vi "comm.vi"() -> ()   [LabVIEW 2015]
uses:
  G_SEN.vi
  G_NAV.vi
panel:
  out "time loop":dbl
  out "time IBEO":dbl format="%#_20g"
  out "Waveform Chart":T1(graph)
  out "output cluster 2":T2 {"Header"."Data type" format="%x"}
  out "value":T3 {"Data type" format="%x"}
  out "scan data 2202":string
  out "object data 2221":string
  out "Ibeo error out":errorcluster
  in  "Ibeo reconn?":bool=TRUE
  in  "Sensor reconn?":bool=TRUE
  in  "Sensor Port":u16=6553
  out "error out":errorcluster
  out "send error":errorcluster
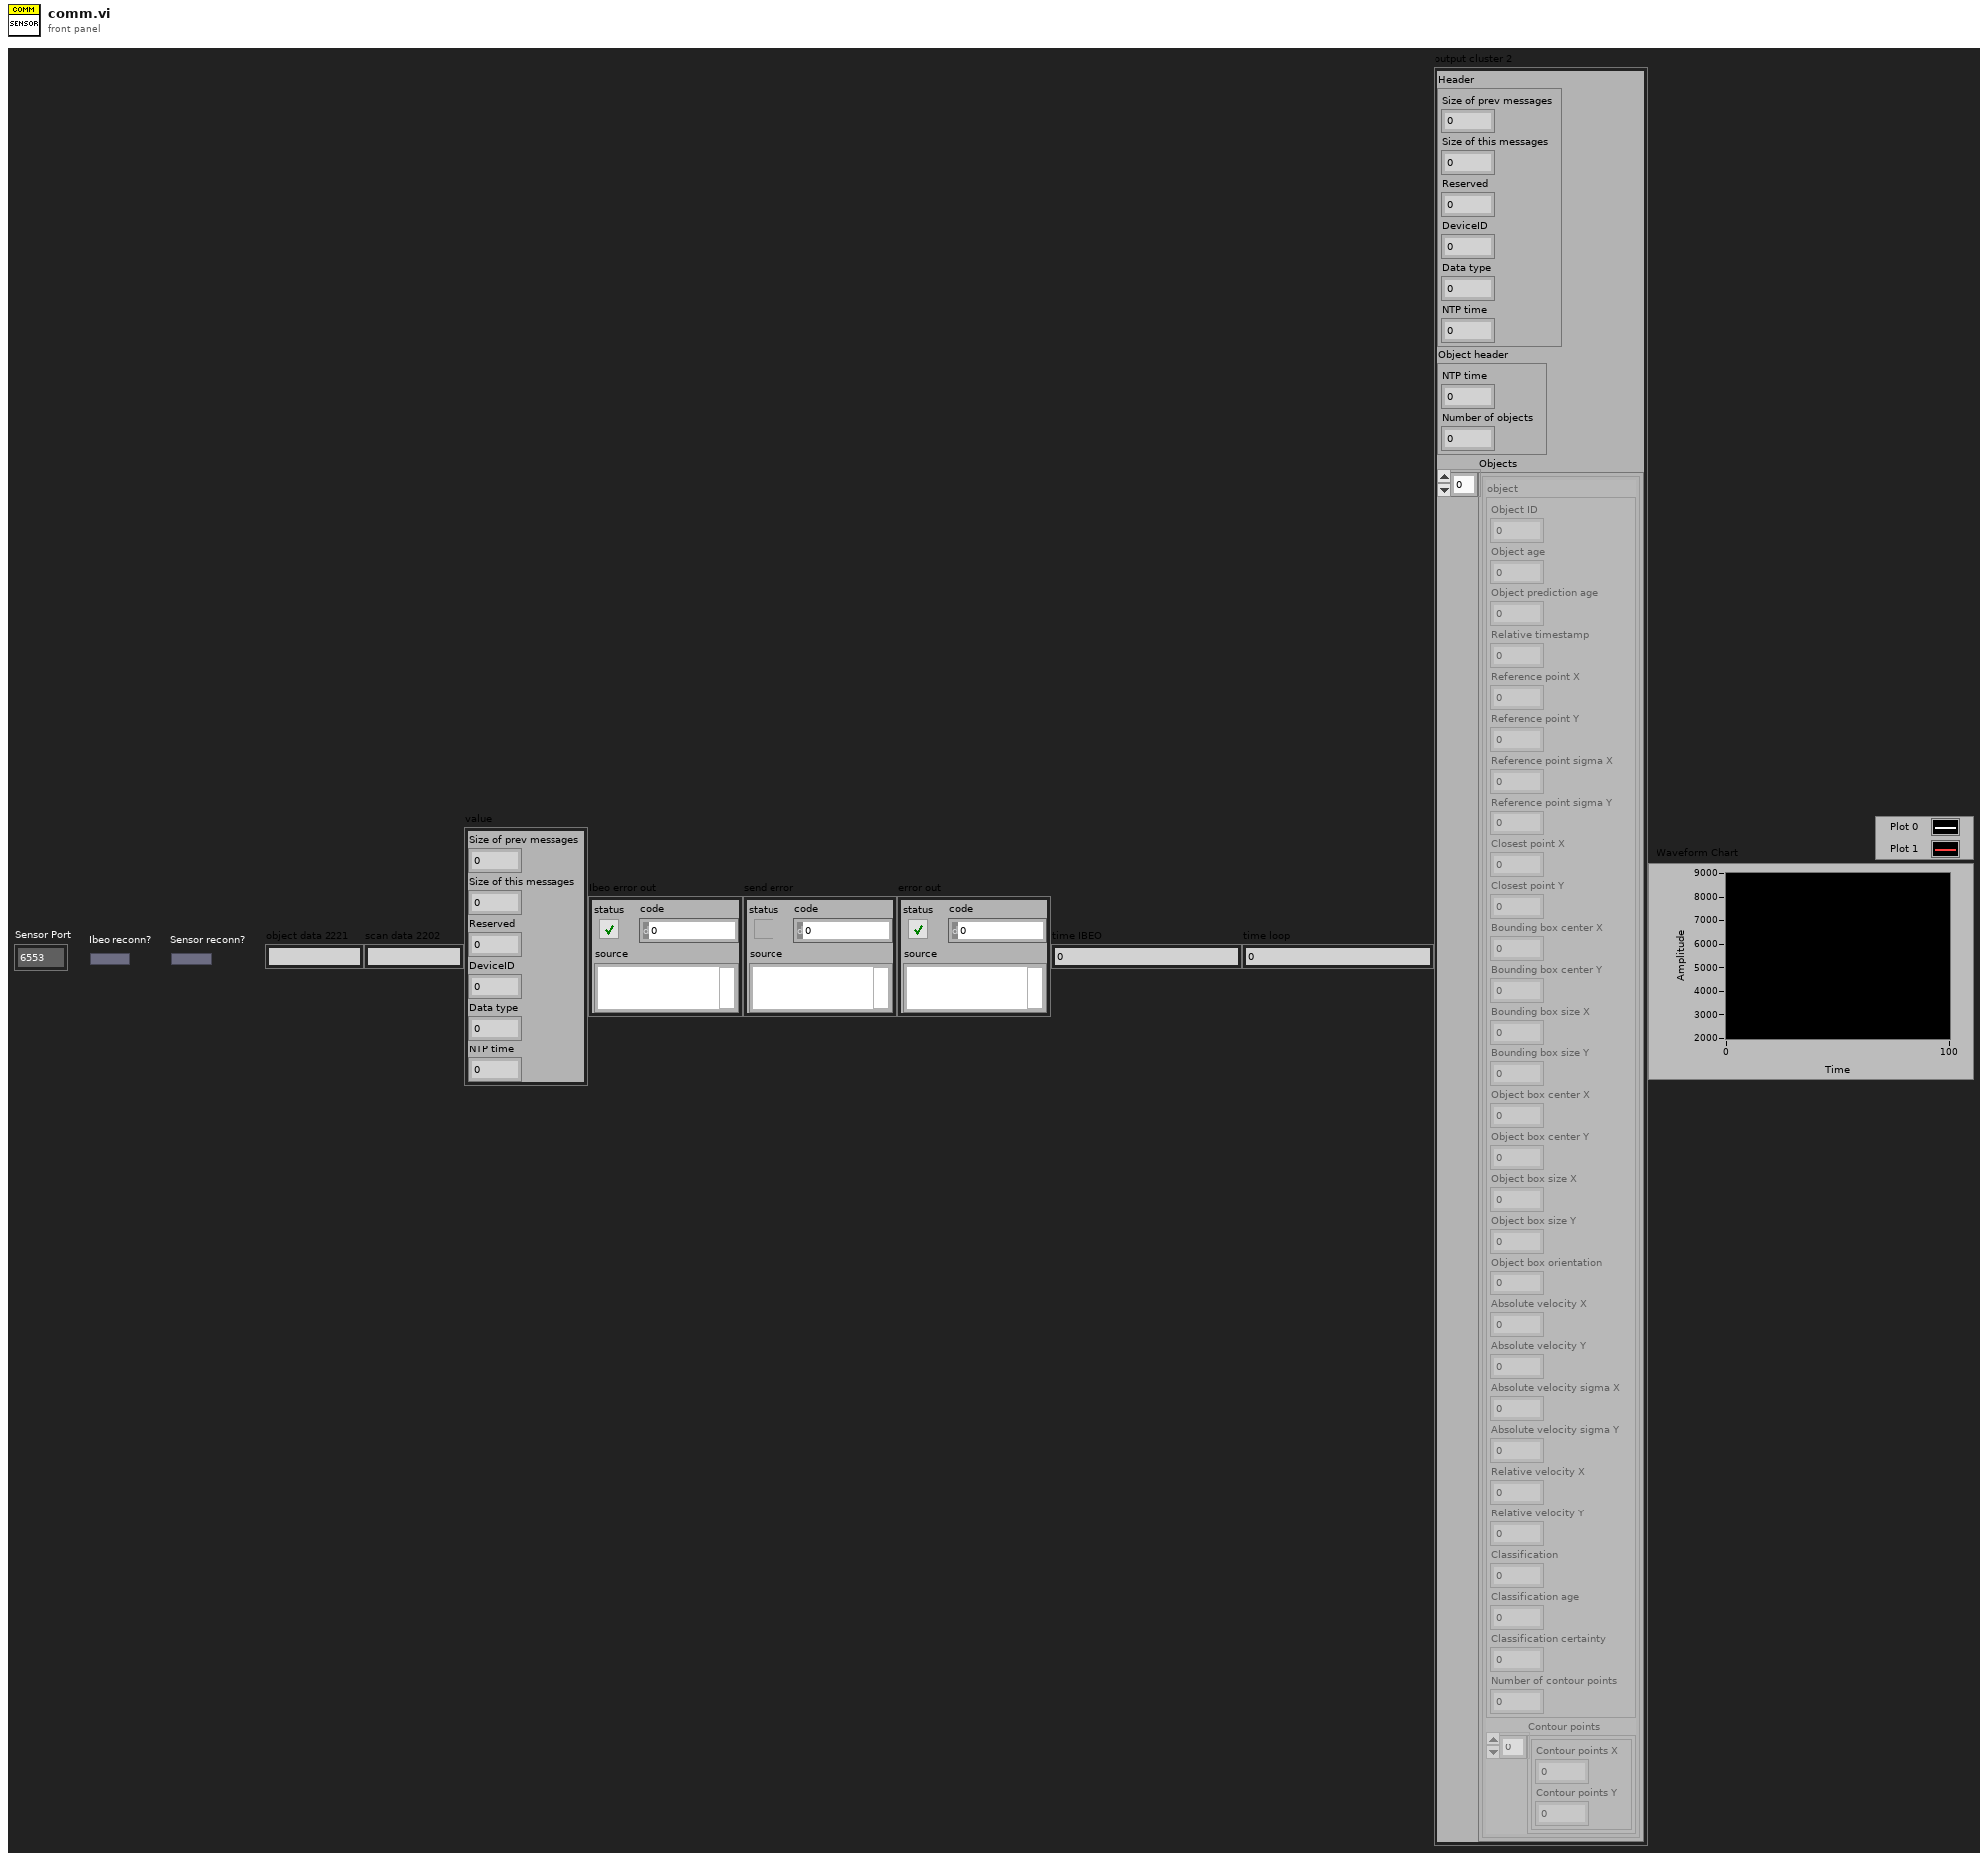
[diagram p1: front panel]
types:
  T1 = cluster{"Data type":u16, "Size of this messages":u32}
  T2 = cluster{"Header":cluster{"Size of prev messages":u32, "Size of this messages":u32, "Reserved":u8, "DeviceID":u8, "Data type":u16, "NTP time":u64}, "Object header":cluster{"NTP time":u64, "Number of objects":u16}, "Objects":cluster{"object":cluster{"Object ID":u16, "Object age ":u16, "Object prediction age":u16, "Relative timestamp":u16, "Reference point X":dbl, "Reference point Y":dbl, "Reference point sigma X":dbl, "Reference point sigma Y":dbl, "Closest point X":dbl, "Closest point Y":dbl, "Bounding box center X":dbl, "Bounding box center Y":dbl, "Bounding box size X":dbl, "Bounding box size Y":dbl, "Object box center X":dbl, "Object box center Y":dbl, "Object box size X":dbl, "Object box size Y":dbl, "Object box orientation":dbl, "Absolute velocity X":dbl, "Absolute velocity Y":dbl, "Absolute velocity sigma X":dbl, "Absolute velocity sigma Y":dbl, "Relative velocity X":dbl, "Relative velocity Y":dbl, "Classification":u16, "Classification age":u16, "Classification certainty":u16, "Number of contour points":u16}, "Contour points":cluster{"Contour points X":dbl, "Contour points Y":dbl}[]}[]}
  T3 = cluster{"Size of prev messages":u32, "Size of this messages":u32, "Reserved":u8, "DeviceID":u8, "Data type":u16, "NTP time":u64}
  T4 = cluster{"global_x":sgl, " global_y":sgl, "yaw":sgl, "objCount":u16, "total":u16}
  T5 = enum16{"big-endian, network order", "native, host order", "little-endian"}
  T6 = cluster{"GPSTime":dbl, "attitude[2]":dbl, "lcc[0]":dbl, "lcc[1]":dbl, "heading_GPS":dbl}
  T7 = cluster{"Header":cluster{"Size of prev messages":u32, "Size of this messages":u32, "Reserved":u8, "DeviceID":u8, "Data type":u16, "NTP time":u64}, "Scan header":cluster{"Scan number":u16, "scanner status":u16, "Sync phase offset":u16, "Scan start time NTP":u64, "Scan end time NTP":u64, "Angle ticks per rotation":u16, "Start angle":dbl, "End angle":dbl, "Scan points":u16, "Mounting position yaw angle ":dbl, "Mounting position pitch angle":dbl, "Mounting position roll angle":dbl, "Mounting position x":dbl, "Mounting position y":dbl, "Mounting position z":dbl, "Reserved":u16}, "Scan points":cluster{"flags":u8, "Echo":u8, "Radial distance":dbl, "Horizontal angle":dbl, "Vertical angle":dbl, "Echo pulse width":u16, "Reserved":u16}[]}
  T8 = cluster{"Header":cluster{"Size of prev messages":u32, "Size of this messages":u32, "Reserved":u8, "DeviceID":u8, "Data type":u16, "NTP time":u64}, "Scan header":cluster{"NTP time":u64, "Scan end Time offset":u32, "flags":u32, "Scan number":u16, "Scan points":u16, "Number of Scan infos":u8, "reserved":u8, "reserved 2":u16}, "Scanner info":cluster{"Device ID ":u8, "Scanner type":u8, "Scan number":u16, "Reserved 4":u32, "Start angle":sgl, "End angle":sgl, "Scan start time ":u64, "Scan end time ":u64, "Scan start time from device":u64, "Scan end time from device":u64, "Scan frequency":sgl, "Beam tilt":sgl, "scan flags":u32, "Yaw angle ":sgl, "Pitch angle ":sgl, "Roll angle":sgl, "Offset x ":sgl, "Offset y":sgl, "Offset z":sgl, "Reserved 8 1":u64, "Reserved 8 2":u64, "Reserved 8 3":u64, "Reserved 8 4":u64, "Reserved 8 5":u64, "Reserved 8 6":u64, "Reserved 8 7":u64, "Reserved 8 8":u64}, "Scan points":cluster{"X  position":sgl, "Y  position":sgl, "Z  position":sgl, "Echo width":sgl, "Device ID ":u8, "Layer":u8, "Echo":u8, "Reserved":u8, "Timestamp":u32, "flags":u16, "Reserved 2":u16}[]}
  T9 = cluster{"Header":cluster{"Size of prev messages":u32, "Size of this messages":u32, "Reserved":u8, "DeviceID":u8, "Data type":u16, "NTP time":u64}, "Object header":cluster{"NTP time":u64, "Number of objects":u16}, "Objects":cluster{"object":cluster{"Object ID":u16, "Reserved 2 1":u16, "Object age ":u32, "Timestamp NTP ":u64, "Object hidden status age":u16, "Classification":u8, "Classification certainty":u8, "Classification age":u32, "Bounding box center X":sgl, "Bounding box center Y":sgl, "Bounding box size X":sgl, "Bounding box size Y":sgl, "Object box center X":sgl, "Object box center Y":sgl, "Object box center sigma X":sgl, "Object box center sigma Y":sgl, "Object box size X":sgl, "Object box size Y":sgl, "Reserved 8 1":u64, "Yaw angle":sgl, "Reserved 4":u32, "Relative velocity X":sgl, "Relative velocity Y":sgl, "Relative velocity sigma X":sgl, "Relative velocity sigma Y":sgl, "Absolute velocity X":sgl, "Absolute velocity Y":sgl, "Absolute velocity sigma X":sgl, "Absolute velocity sigma Y":sgl, "Reserved 8 3":u64, "Reserved 8 4":u64, "Reserved 2 2":u16, "Number of contour points":u8, "Index of closest point":u8}, "Contour Points":cluster{"contour points X":sgl, "contour points Y":sgl}[]}[]}
  T10 = cluster{"Scan number":u16, "scanner status":u16, "Sync phase offset":u16, "Scan start time NTP":u64, "Scan end time NTP":u64, "Angle ticks per rotation":u16, "Start angle":i16, "End angle":i16, "Scan points":u16, "Mounting position yaw angle ":i16, "Mounting position pitch angle":i16, "Mounting position roll angle":i16, "Mounting position x":i16, "Mounting position y":i16, "Mounting position z":i16, "Reserved":u16}
  T11 = cluster{"flags":u8, "Echo":u8, "Radial distance":dbl, "Horizontal angle":dbl, "Vertical angle":dbl, "Echo pulse width":u16, "Reserved":u16}
  T12 = cluster{"Layer/Echo":u8, "flags":u8, "Horizontal angle":i16, "Radial distance":u16, "Echo pulse width":u16, "Reserved":u16}
  T13 = cluster{"Scan number":u16, "scanner status":u16, "Sync phase offset":u16, "Scan start time NTP":u64, "Scan end time NTP":u64, "Angle ticks per rotation":u16, "Start angle":dbl, "End angle":dbl, "Scan points":u16, "Mounting position yaw angle ":dbl, "Mounting position pitch angle":dbl, "Mounting position roll angle":dbl, "Mounting position x":dbl, "Mounting position y":dbl, "Mounting position z":dbl, "Reserved":u16}
  T14 = cluster{"Device ID ":u8, "Scanner type":u8, "Scan number":u16, "Reserved 4":u32, "Start angle":sgl, "End angle":sgl, "Scan start time ":u64, "Scan end time ":u64, "Scan start time from device":u64, "Scan end time from device":u64, "Scan frequency":sgl, "Beam tilt":sgl, "scan flags":u32, "Yaw angle ":sgl, "Pitch angle ":sgl, "Roll angle":sgl, "Offset x ":sgl, "Offset y":sgl, "Offset z":sgl, "Reserved 8 1":u64, "Reserved 8 2":u64, "Reserved 8 3":u64, "Reserved 8 4":u64, "Reserved 8 5":u64, "Reserved 8 6":u64, "Reserved 8 7":u64, "Reserved 8 8":u64}
  T15 = cluster{"NTP time":u64, "Scan end Time offset":u32, "flags":u32, "Scan number":u16, "Scan points":u16, "Number of Scan infos":u8, "reserved":u8, "reserved 2":u16}
  T16 = cluster{"X  position":sgl, "Y  position":sgl, "Z  position":sgl, "Echo width":sgl, "Device ID ":u8, "Layer":u8, "Echo":u8, "Reserved":u8, "Timestamp":u32, "flags":u16, "Reserved 2":u16}
  T17 = cluster{"Object ID":u16, "Object age ":u16, "Object prediction age":u16, "Relative timestamp":u16, "Reference point X":i16, "Reference point Y":i16, "Reference point sigma X":i16, "Reference point sigma Y":i16, "Closest point X":i16, "Closest point Y":i16, "Bounding box center X":i16, "Bounding box center Y":i16, "Bounding box size X":u16, "Bounding box size Y":u16, "Object box center X":i16, "Object box center Y":i16, "Object box size X":u16, "Object box size Y":u16, "Object box orientation":i16, "Absolute velocity X":i16, "Absolute velocity Y":i16, "Absolute velocity sigma X":u16, "Absolute velocity sigma Y":u16, "Relative velocity X":i16, "Relative velocity Y":i16, "Classification":u16, "Classification age":u16, "Classification certainty":u16, "Number of contour points":u16}
  T18 = cluster{"contour points X":i16, "contour points Y":i16}
  T19 = cluster{"contour points X":dbl, "contour points Y":dbl}
  T20 = cluster{"Object ID":u16, "Object age ":u16, "Object prediction age":u16, "Relative timestamp":u16, "Reference point X":dbl, "Reference point Y":dbl, "Reference point sigma X":dbl, "Reference point sigma Y":dbl, "Closest point X":dbl, "Closest point Y":dbl, "Bounding box center X":dbl, "Bounding box center Y":dbl, "Bounding box size X":dbl, "Bounding box size Y":dbl, "Object box center X":dbl, "Object box center Y":dbl, "Object box size X":dbl, "Object box size Y":dbl, "Object box orientation":dbl, "Absolute velocity X":dbl, "Absolute velocity Y":dbl, "Absolute velocity sigma X":dbl, "Absolute velocity sigma Y":dbl, "Relative velocity X":dbl, "Relative velocity Y":dbl, "Classification":u16, "Classification age":u16, "Classification certainty":u16, "Number of contour points":u16}
  T21 = cluster{"Object ID":dbl, "Object age ":dbl, "Object prediction age":dbl, "Relative timestamp":dbl, "Reference point X":dbl, "Reference point Y":dbl, "Reference point sigma X":dbl, "Reference point sigma Y":dbl, "Closest point X":dbl, "Closest point Y":dbl, "Bounding box center X":dbl, "Bounding box center Y":dbl, "Bounding box size X":dbl, "Bounding box size Y":dbl, "Object box center X":dbl, "Object box center Y":dbl, "Object box size X":dbl, "Object box size Y":dbl, "Object box orientation":dbl, "Absolute velocity X":dbl, "Absolute velocity Y":dbl, "Absolute velocity sigma X":dbl, "Absolute velocity sigma Y":dbl, "Relative velocity X":dbl, "Relative velocity Y":dbl, "Classification":dbl, "Classification age":dbl, "Classification certainty":dbl, "Number of contour points":dbl}
  T22 = cluster{"object":cluster{"Object ID":u16, "Object age ":u16, "Object prediction age":u16, "Relative timestamp":u16, "Reference point X":dbl, "Reference point Y":dbl, "Reference point sigma X":dbl, "Reference point sigma Y":dbl, "Closest point X":dbl, "Closest point Y":dbl, "Bounding box center X":dbl, "Bounding box center Y":dbl, "Bounding box size X":dbl, "Bounding box size Y":dbl, "Object box center X":dbl, "Object box center Y":dbl, "Object box size X":dbl, "Object box size Y":dbl, "Object box orientation":dbl, "Absolute velocity X":dbl, "Absolute velocity Y":dbl, "Absolute velocity sigma X":dbl, "Absolute velocity sigma Y":dbl, "Relative velocity X":dbl, "Relative velocity Y":dbl, "Classification":u16, "Classification age":u16, "Classification certainty":u16, "Number of contour points":u16}, cluster{"contour points X":dbl, "contour points Y":dbl}[]}
  T23 = cluster{"Object ID":u16, "Reserved 2 1":u16, "Object age ":u32, "Timestamp NTP ":u64, "Object hidden status age":u16, "Classification":u8, "Classification certainty":u8, "Classification age":u32, "Bounding box center X":sgl, "Bounding box center Y":sgl, "Bounding box size X":sgl, "Bounding box size Y":sgl, "Object box center X":sgl, "Object box center Y":sgl, "Object box center sigma X":sgl, "Object box center sigma Y":sgl, "Object box size X":sgl, "Object box size Y":sgl, "Reserved 8 1":u64, "Yaw angle":sgl, "Reserved 4":u32, "Relative velocity X":sgl, "Relative velocity Y":sgl, "Relative velocity sigma X":sgl, "Relative velocity sigma Y":sgl, "Absolute velocity X":sgl, "Absolute velocity Y":sgl, "Absolute velocity sigma X":sgl, "Absolute velocity sigma Y":sgl, "Reserved 8 3":u64, "Reserved 8 4":u64, "Reserved 2 2":u16, "Number of contour points":u8, "Index of closest point":u8}
  T24 = cluster{"contour points X":sgl, "contour points Y":sgl}
  T25 = cluster{"object":cluster{"Object ID":u16, "Reserved 2 1":u16, "Object age ":u32, "Timestamp NTP ":u64, "Object hidden status age":u16, "Classification":u8, "Classification certainty":u8, "Classification age":u32, "Bounding box center X":sgl, "Bounding box center Y":sgl, "Bounding box size X":sgl, "Bounding box size Y":sgl, "Object box center X":sgl, "Object box center Y":sgl, "Object box center sigma X":sgl, "Object box center sigma Y":sgl, "Object box size X":sgl, "Object box size Y":sgl, "Reserved 8 1":u64, "Yaw angle":sgl, "Reserved 4":u32, "Relative velocity X":sgl, "Relative velocity Y":sgl, "Relative velocity sigma X":sgl, "Relative velocity sigma Y":sgl, "Absolute velocity X":sgl, "Absolute velocity Y":sgl, "Absolute velocity sigma X":sgl, "Absolute velocity sigma Y":sgl, "Reserved 8 3":u64, "Reserved 8 4":u64, "Reserved 2 2":u16, "Number of contour points":u8, "Index of closest point":u8}, cluster{"contour points X":sgl, "contour points Y":sgl}[]}
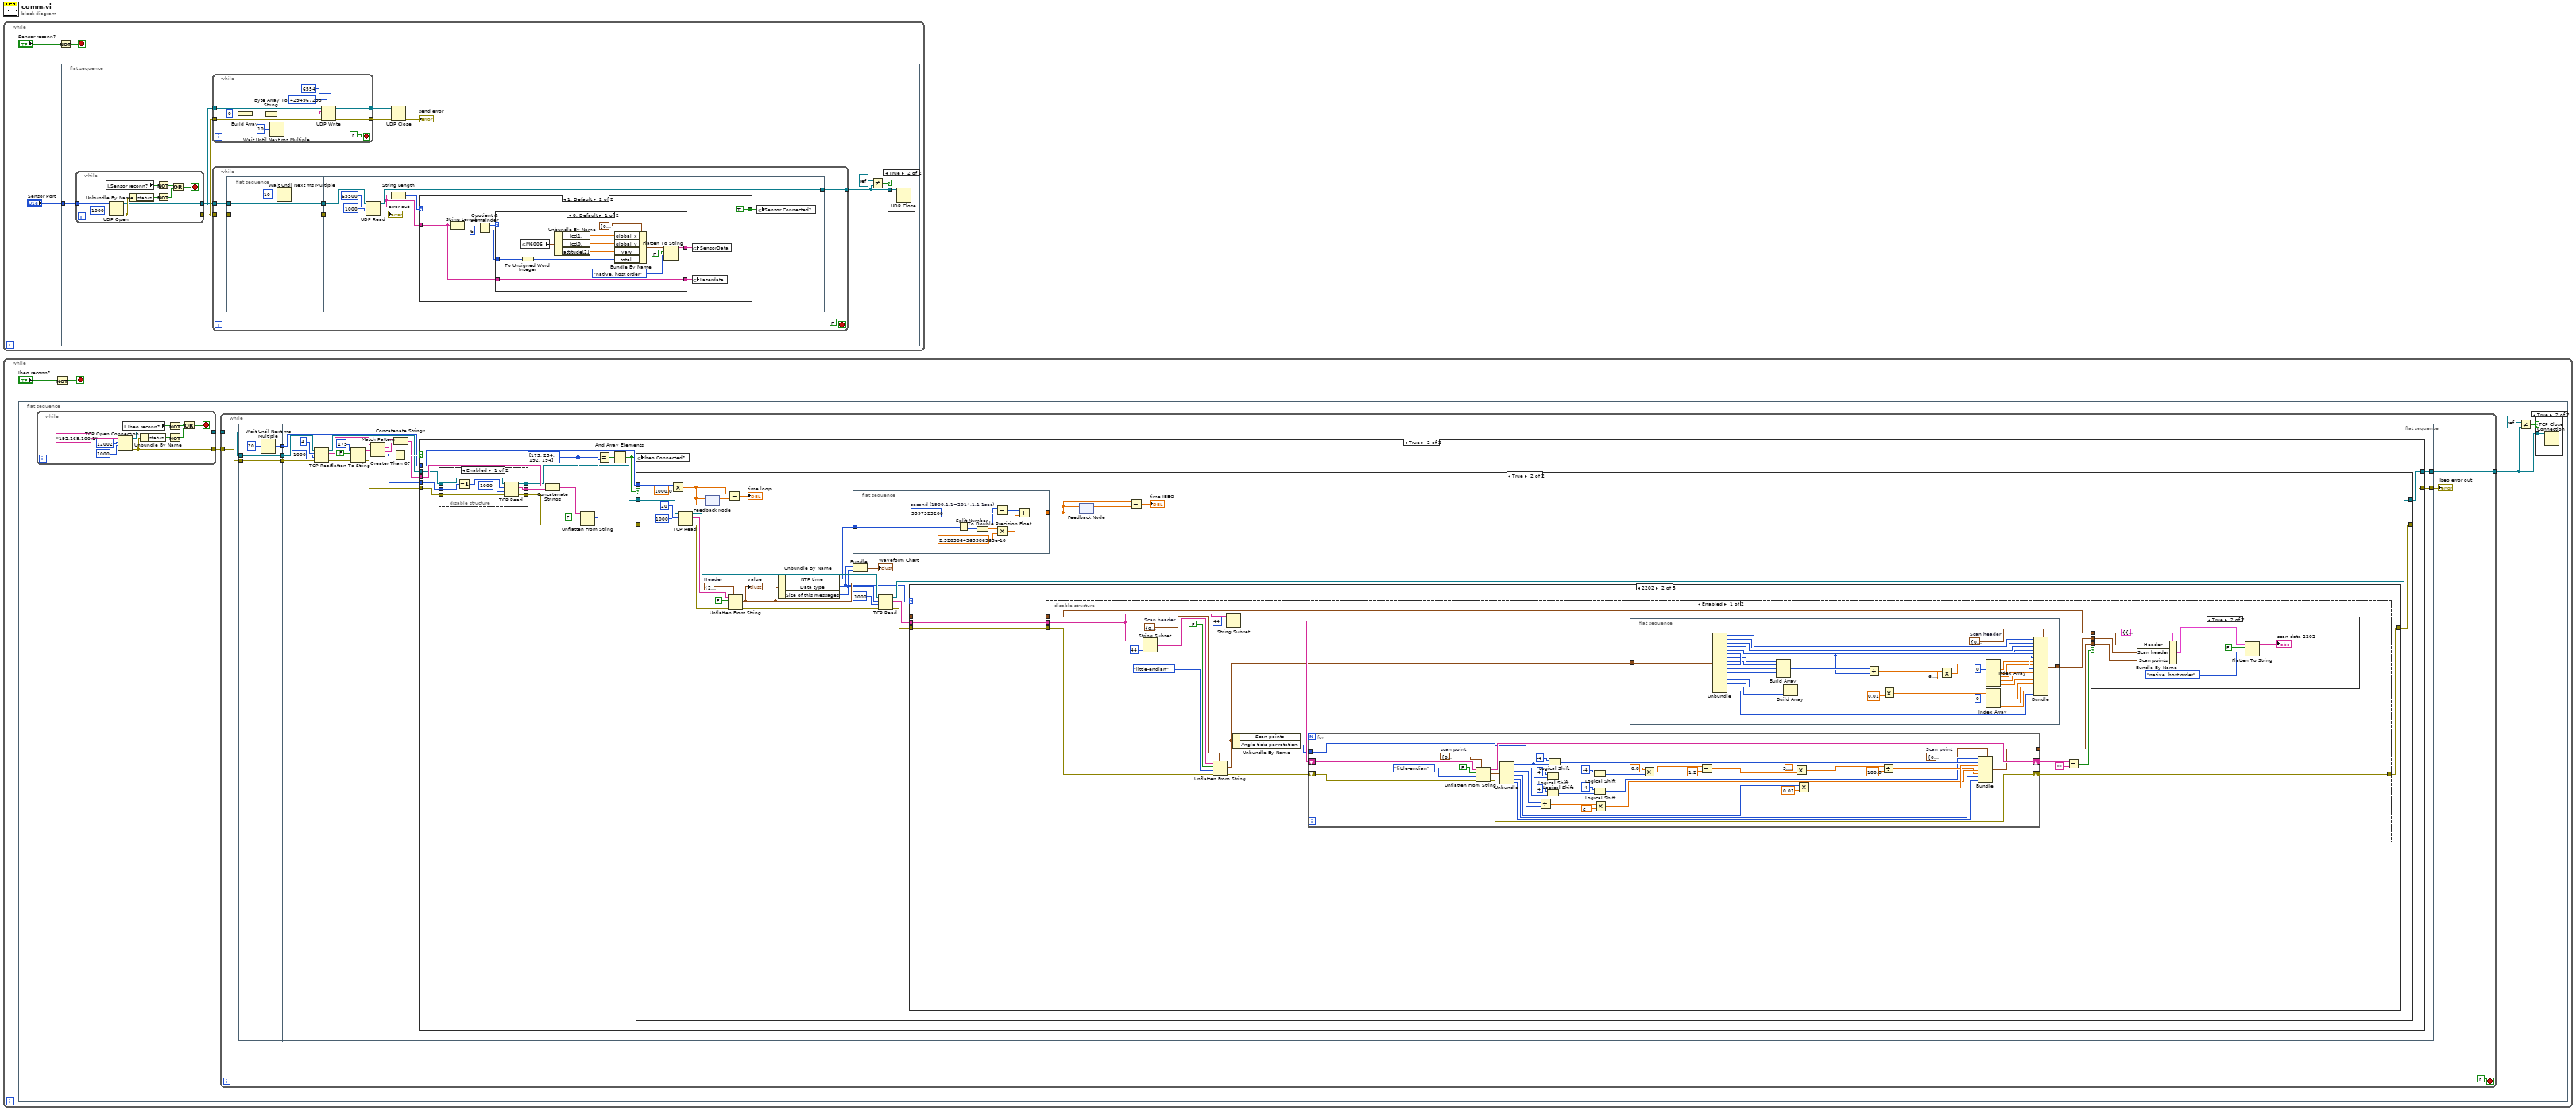
[diagram p0: block diagram]
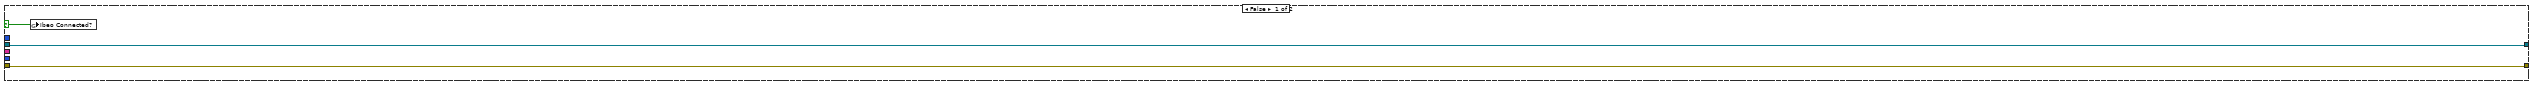
[diagram p3: hidden frame]
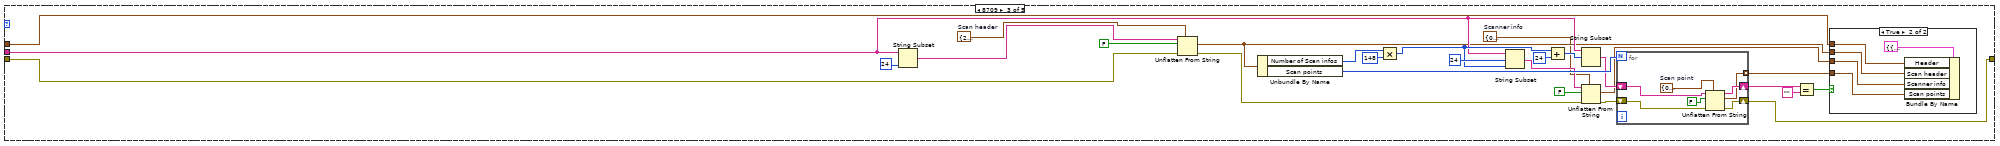
[diagram p9: hidden frame]
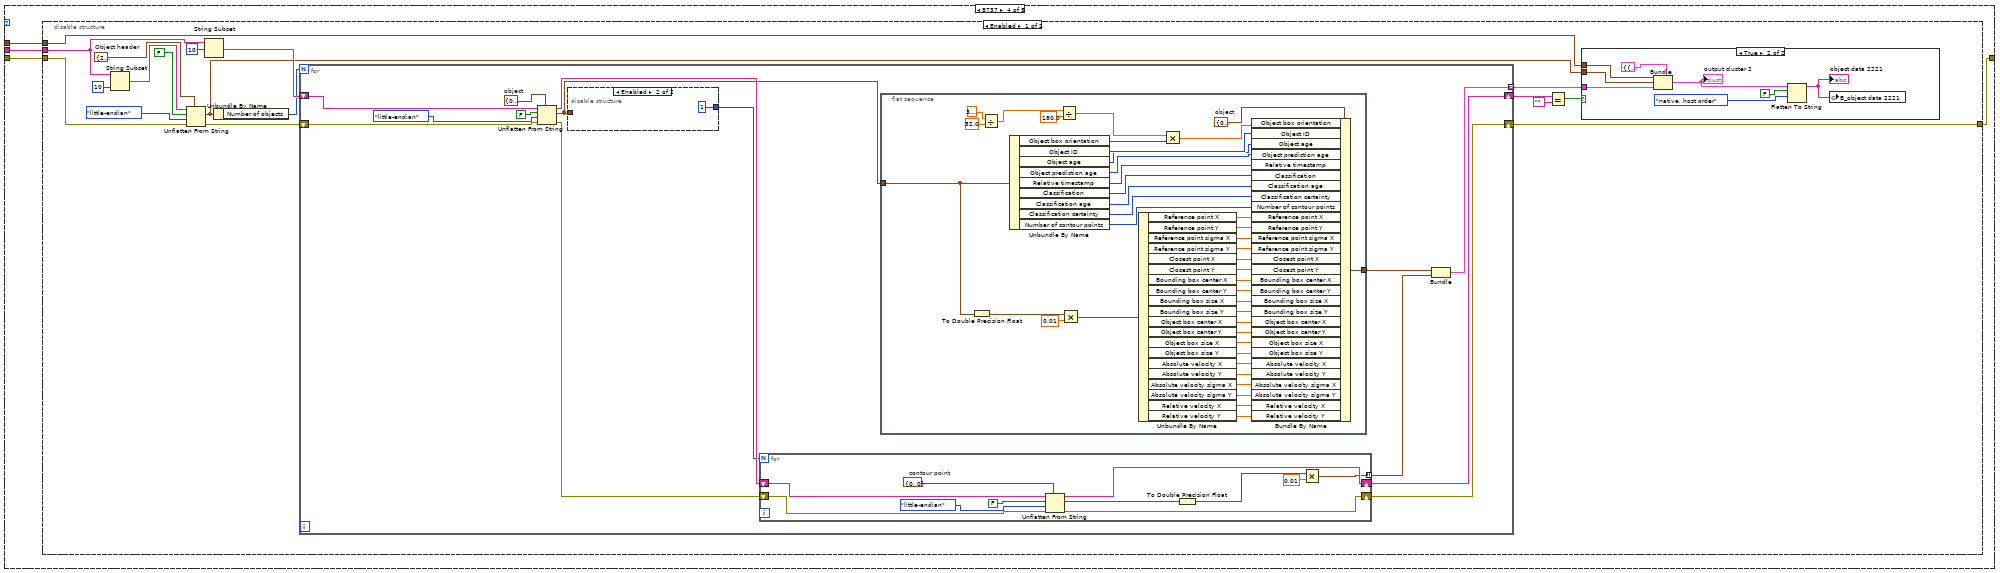
[diagram p11: hidden frame]
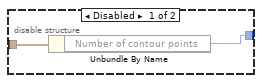
[diagram p13: hidden frame]
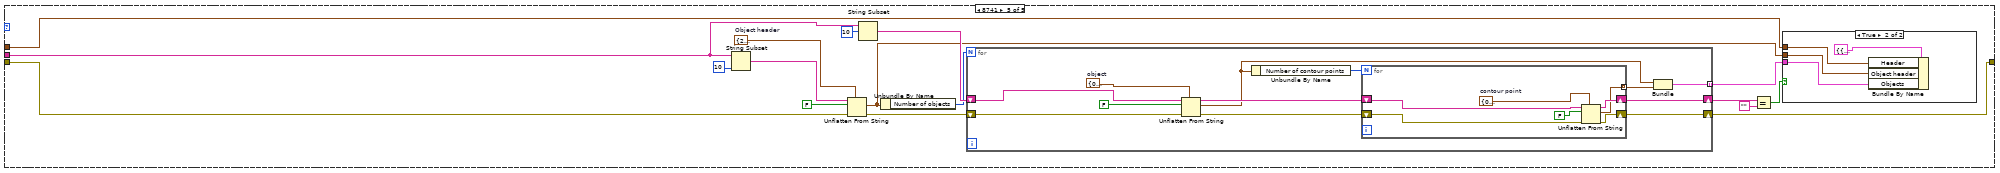
[diagram p15: hidden frame]
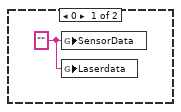
[diagram p18: hidden frame]
diagram:
  n1 = while {
    stop <- w2 stop-if-true
    n2 = Not(x="Sensor reconn?") -> (.not. x?=w2:bool)
    n3 = flat-sequence {
      tunnel: "Sensor Port" -> [w10]
      frame #0 {
        n4 = while {
          tunnel: [w64] -> w5
          tunnel: [w67] -> w6
          tunnel: w10 -> [w66]
          stop <- w68 stop-if-true
          n5 = local read "Sensor reconn?"() -> (w70:bool)
          n6 = UDP Open(9:1000 ("timeout ms (25000)"), 11:w66) -> (port=w64:refnum<k16>, 0:w67:errorcluster)  [unwired: 3 in, 1 out]
          n7 = Unbundle By Name(w67) -> ("status"=w69:bool)
          n8 = Not(x=w70) -> (.not. x?=w71:bool)
          n9 = Not(x=w69) -> (.not. x?=w65:bool)
          n10 = Or(x=w71, y=w65) -> (x .or. y?=w68:bool)
        }
        n11 = while {
          tunnel: w5 -> [w22]
          tunnel: w6 -> [w21]
          tunnel: [w20] -> w7
          tunnel: [w19] -> w8
          stop <- FALSE stop-if-true
          n12 = Build Array(u8 0 ("element")) -> (w13:u8[])
          n13 = Byte Array To String(unsigned byte array=w13) -> (string=w17:string)
          n14 = Wait Until Next ms Multiple(millisecond multiple=u32 10) -> ()  [unwired: 1 out]
          n15 = UDP Write(address=u32 4294967295, port or service name=u16 6554, connection ID=w22, data in=w17, 8:w21) -> (error out=w20:errorcluster, 3:w19:refnum<k16>)  [unwired: 1 in]
        }
        n16 = while {
          tunnel: w6 -> [w29]
          tunnel: w5 -> [w30]
          tunnel: [w25] -> w4
          stop <- FALSE stop-if-true
          n17 = flat-sequence {
            tunnel: w29 -> [w32]
            tunnel: w30 -> [w33]
            tunnel: [w33] -> w27
            tunnel: [w32] -> w26
            tunnel: w27 -> [w42]
            tunnel: w26 -> [w41]
            tunnel: [w34] -> w25
            frame #0 {
              n18 = Wait Until Next ms Multiple(millisecond multiple=u32 10 ("milliseconds to wait")) -> ()  [unwired: 1 out]
            }
            frame #1 {
              n19 = UDP Read(connection ID=w42, max size (548)=65500, timeout ms (25000)=1000, 8:w41) -> (data out=w37:string, error out=→"error out":errorcluster, 3:w34:refnum<k16>)  [unwired: 2 out]
              n20 = String Length(string=w37) -> (length=w38:i32)
              n21 = case shown="1, Default" w38 {
                tunnel: w37 -> [_ w45]
                tunnel: [_ TRUE] -> w36
                frame 0 {
                  w43 = "" ("Laserdata")
                  n22 = global write "G_SEN.vi" "SensorData"(w43) -> ()
                  n23 = global write "G_SEN.vi" "Laserdata"(w43) -> ()
                }
                frame 1, Default {
                  n24 = String Length(string=w45) -> (length=w50:i32)
                  n25 = Quotient & Remainder(x=w50, y=6) -> (x-y*floor(x/y)=w47:i32, floor(x/y)=w48:i32)
                  n26 = case shown="0, Default" w47 {
                    tunnel: [w55 _] -> w51
                    tunnel: w48 -> [w53 _]
                    tunnel: [w52 _] -> w46
                    tunnel: w45 -> [w52 _]
                    frame 0, Default {
                      n27 = To Unsigned Word Integer(number=w53) -> (unsigned 16bit integer=w54:u16)
                      n28 = global read "G_NAV.vi" "M6006"() -> (w60:T6)
                      n29 = Unbundle By Name(w60) -> ("lcc[1]"=w61:dbl, "lcc[0]"=w62:dbl, "attitude[2]"=w63:dbl)
                      n30 = Bundle By Name(cluster=T4 {"global_x"=0.0, " global_y"=0.0, "yaw"=0.0, "objCount"=0, "total"=0} ("sensor"), "global_x"=w61, "global_y"=w62, "yaw"=w63, "total"=w54) -> (w57:T4)
                      n31 = Flatten To String(anything=w57, prepend array or string size? (T)=FALSE, byte order (0:big-endian, network order)=T5."native, host order") -> (data string=w55:string)  [unwired: 1 in, 2 out]
                    }
                    frame 1 {
                    }
                  }
                  n32 = global write "G_SEN.vi" "SensorData"(w51) -> ()
                  n33 = global write "G_SEN.vi" "Laserdata"(w46) -> ()
                }
              }
              n34 = global write "G_SEN.vi" "Sensor Connected?"(w36) -> ()
            }
          }
        }
        n35 = UDP Close(connection ID=w8, 8:w7) -> (error out=→"send error":errorcluster)  [unwired: 1 out]
        n36 = Not Equal?(x=refnum<k16> refnum ("connection ID"), y=w4) -> (x != y?=w11:bool)
        n37 = case shown="True" w11 {
          tunnel: w4 -> [_ w24]
          frame False {
          }
          frame True {
            n38 = UDP Close(connection ID=w24) -> ()  [unwired: 1 in, 2 out]
          }
        }
      }
    }
  }
  n39 = while {
    stop <- w73 stop-if-true
    n40 = flat-sequence {
      frame #0 {
        n41 = while {
          tunnel: [w469] -> w77
          tunnel: [w471] -> w78
          stop <- w472 stop-if-true
          n42 = TCP Open Connection(address="192.168.100.1", remote port or service name=u16 12002 ("Sensor Port 2"), timeout ms (60000)=1000 ("timeout ms (25000)")) -> (connection ID=w469:refnum<k5>, error out=w471:errorcluster)  [unwired: 2 in]
          n43 = local read "Ibeo reconn?"() -> (w474:bool)
          n44 = Unbundle By Name(w471) -> ("status"=w473:bool)
          n45 = Not(x=w474) -> (.not. x?=w475:bool)
          n46 = Not(x=w473) -> (.not. x?=w470:bool)
          n47 = Or(x=w475, y=w470) -> (x .or. y?=w472:bool)
        }
        n48 = while {
          tunnel: w78 -> [w87]
          tunnel: w77 -> [w88]
          tunnel: [w83] -> w76
          stop <- FALSE stop-if-true
          n49 = flat-sequence {
            tunnel: w87 -> [w91]
            tunnel: w88 -> [w92]
            tunnel: [w92] -> w85
            tunnel: [w91] -> w84
            tunnel: [w89] -> w81
            tunnel: w85 -> [w111]
            tunnel: w84 -> [w98]
            tunnel: [w110] -> w83
            tunnel: [w95] -> w82
            tunnel: w81 -> [w93]
            frame #0 {
              n50 = Wait Until Next ms Multiple(millisecond multiple=u32 20 ("milliseconds to wait")) -> (millisecond timer value=w89:u32)
            }
            frame #1 {
              n51 = TCP Read(connection ID=w111, bytes to read=4 ("count (1)"), error in (no error)=w98, 9:1000 ("timeout ms (25000)")) -> (connection ID out=w99:refnum<k5>, data out=w105:string, error out=w97:errorcluster)  [unwired: 1 in]
              n52 = Flatten To String(anything=u8 175, prepend array or string size? (T)=FALSE, error in (no error)=w97) -> (data string=w106:string, error out=w96:errorcluster)  [unwired: 1 in, 1 out]
              n53 = Match Pattern(string=w105, regular expression=w106) -> (match substring=w102:string, after substring=w101:string, offset past match=w103:i32)  [unwired: 1 in, 1 out]
              n54 = Greater Than 0?(x=w103) -> (x > 0?=w104:bool)
              n55 = Concatenate Strings(w102, w101) -> (w100:string)
              n56 = case shown="True" w104 {
                selector: w104 -> [w112 _]
                tunnel: w103 -> [_ w131]
                tunnel: w99 -> [w114 w125]
                tunnel: w100 -> [_ w130]
                tunnel: [w114 w124] -> w110
                tunnel: w96 -> [w113 w121]
                tunnel: [w113 w118] -> w95
                tunnel: w93 -> [_ w116]
                frame False {
                  n57 = global write "G_SEN.vi" "Ibeo Connected?"(w112) -> ()
                }
                frame True {
                  w122 = u8[] [175, 254, 192, 194] ("value")
                  n58 = disable-structure shown="Enabled" {
                    disable-tunnel: w131 -> [w139 _]
                    disable-tunnel: [w137 _] -> w129
                    disable-tunnel: w125 -> [w136 w140]
                    disable-tunnel: w121 -> [w135 _]
                    disable-tunnel: [w134 _] -> w120
                    disable-tunnel: [w132 w140] -> w117
                    frame Enabled {
                      n59 = Decrement(x=w139) -> (x-1=w138:i32)
                      n60 = TCP Read(connection ID=w136, bytes to read=w138, error in (no error)=w135, 9:1000 ("timeout ms (25000)")) -> (connection ID out=w132:refnum<k5>, data out=w137:string, error out=w134:errorcluster)  [unwired: 1 in]
                    }
                    frame Disabled {
                    }
                  }
                  n61 = Concatenate Strings(w130, w129) -> (w127:string)
                  n62 = Unflatten From String(type=w122, binary string=w127, data includes array or string size? (T)=FALSE, error in (no error)=w120) -> (value=w123:u8[], error out=w119:errorcluster)  [unwired: 1 in, 1 out]
                  n63 = Equal?(x=w122, y=w123) -> (x = y?=w126:bool[])
                  n64 = And Array Elements(Boolean array=w126) -> (logical AND=w115:bool)
                  n65 = global write "G_SEN.vi" "Ibeo Connected?"(w115) -> ()
                  n66 = case shown="True" w115 {
                    tunnel: w117 -> [w142 w170]
                    tunnel: [w142 w164] -> w124
                    tunnel: w119 -> [w141 w161]
                    tunnel: [w141 w157] -> w118
                    tunnel: w116 -> [_ w150]
                    frame False {
                    }
                    frame True {
                      w168 = T3 {"Size of prev messages"=20, "Size of this messages"=20, "Reserved"=20, "DeviceID"=20, "Data type"=20, "NTP time"=20}  # Header
                      n67 = Multiply(x=w150, y=1000.0) -> (x*y=w147:dbl)
                      n68 = TCP Read(connection ID=w170, bytes to read=20 ("count (1)"), error in (no error)=w161, 9:1000 ("timeout ms (25000)")) -> (connection ID out=w165:refnum<k5>, data out=w167:string, error out=w160:errorcluster)  [unwired: 1 in]
                      n69 = feedback-in #1(w147) -> ()
                      n70 = feedback #1(w147) -> (w148:dbl)
                      n71 = Subtract(x=w147, y=w148) -> (x-y=→"time loop":dbl)
                      n72 = Unflatten From String(type=w168, binary string=w167, data includes array or string size? (T)=FALSE, error in (no error)=w160) -> (value=w162:T3, error out=w159:errorcluster)  [unwired: 1 in, 1 out]
                      "value" <- w162
                      n73 = Unbundle By Name(w162) -> ("NTP time"=w156:u64, "Data type"=w153:u16, "Size of this messages"=w152:u32)
                      n74 = flat-sequence {
                        tunnel: w156 -> [w179]
                        tunnel: [w178] -> w146
                        frame #0 {
                          w173 = u32 3597523200  # second (1900.1.1~2014.1.1-1sec)
                          n75 = Split Number(x=w179) -> (hi(x)=w172:u32, lo(x)=w177:u32)
                          n76 = To Double Precision Float(number=w177) -> (double precision float=w176:dbl)
                          n77 = Subtract(x=w172, y=w173) -> (x-y=w171:u32)
                          n78 = Multiply(x=w176, y=2.3283064365386963e-10) -> (x*y=w174:dbl)
                          n79 = Add(x=w171, y=w174) -> (x+y=w178:dbl)
                        }
                      }
                      n80 = Bundle("Data type"=w153, "Size of this messages"=w152) -> (→"Waveform Chart":T1)  [unwired: 1 in]
                      n81 = TCP Read(connection ID=w165, bytes to read=w152, error in (no error)=w159, 9:1000 ("timeout ms (25000)")) -> (connection ID out=w164:refnum<k5>, data out=w163:string, error out=w158:errorcluster)  [unwired: 1 in]
                      n82 = case shown="2202" w153 {
                        tunnel: w163 -> [_ w184 w307 w331 w438]
                        tunnel: w162 -> [_ w183 w302 w330 w435]
                        tunnel: w158 -> [w180 w182 w292 w329 w429]
                        tunnel: [w180 w181 w289 w328 w427] -> w157
                        frame 0, Default {
                        }
                        frame 8706 {
                          n83 = disable-structure shown="Enabled" {
                            disable-tunnel: w184 -> [w201 _]
                            disable-tunnel: w183 -> [w196 _]
                            disable-tunnel: w182 -> [w188 _]
                            disable-tunnel: [w186 _] -> w181
                            frame Enabled {
                              w199 = T10 {"Scan number"=0, "scanner status"=0, "Sync phase offset"=0, "Scan start time NTP"=0, "Scan end time NTP"=0, "Angle ticks per rotation"=0, "Start angle"=0, "End angle"=0, "Scan points"=0, "Mounting position yaw angle "=0, "Mounting position pitch angle"=0, "Mounting position roll angle"=0, "Mounting position x"=0, "Mounting position y"=0, "Mounting position z"=0, "Reserved"=0}  # Scan header
                              n84 = String Subset(string=w201, length (rest)=44 ("length (rest)")) -> (substring=w203:string)  [unwired: 1 in]
                              n85 = Unflatten From String(type=w199, binary string=w203, data includes array or string size? (T)=FALSE, byte order (0:big-endian, network order)=T5."little-endian", error in (no error)=w188) -> (value=w194:T10, error out=w187:errorcluster)  [unwired: 1 out]
                              n86 = String Subset(string=w201, offset (0)=u16 44 ("y")) -> (substring=w200:string)  [unwired: 1 in]
                              n87 = Unbundle By Name(w194) -> ("Scan points"=w197:u16, "Angle ticks per rotation"=w195:u16)
                              n88 = for {
                                N: w197 -> [_]
                                shift-right: [w285] -> w189
                                shift-left: w200 -> [w288]
                                tunnel: w195 -> [w272]
                                tunnel: [w268] -> w193 mode=indexing
                                shift-right: [w266] -> w186
                                shift-left: w187 -> [w267]
                                w279 = T11 {"flags"=0, "Echo"=0, "Radial distance"=0.0, "Horizontal angle"=0.0, "Vertical angle"=0.0, "Echo pulse width"=0, "Reserved"=0}  # Scan point
                                w286 = T12 {"Layer/Echo"=0, "flags"=0, "Horizontal angle"=0, "Radial distance"=0, "Echo pulse width"=0, "Reserved"=0}  # scan point
                                n89 = Unflatten From String(type=w286, binary string=w288, data includes array or string size? (T)=FALSE, byte order (0:big-endian, network order)=T5."little-endian", error in (no error)=w267) -> (rest of the binary string=w285:string, value=w284:T12, error out=w266:errorcluster)
                                n90 = Unbundle(w284) -> ("Layer/Echo"=w274:u8, "flags"=w250:u8, "Horizontal angle"=w273:i16, "Radial distance"=w254:u16, "Echo pulse width"=w261:u16, "Reserved"=w260:u16)
                                n91 = Divide(x=w273, y=w272) -> (x/y=w271:dbl)
                                n92 = Logical Shift(y=i16 4, x=w274) -> (x << y=w282:u8)
                                n93 = Logical Shift(y=i16 4, x=w250) -> (x << y=w252:u8)
                                n94 = Logical Shift(y=i16 -4, x=w274) -> (x << y=w264:u8)
                                n95 = Logical Shift(y=i16 -4, x=w282) -> (x << y=w278:u8)
                                n96 = Logical Shift(y=i16 -4, x=w252) -> (x << y=w249:u8)
                                n97 = Multiply(x=w271, y=6.283185307179586) -> (x*y=w262:dbl)
                                n98 = Multiply(x=0.8, y=w278) -> (x*y=w276:dbl)
                                n99 = Subtract(x=w276, y=1.2) -> (x-y=w259:dbl)
                                n100 = Multiply(x=3.141592653589793, y=w259) -> (x*y=w257:dbl)
                                n101 = Multiply(x=w254, y=0.01) -> (x*y=w263:dbl)
                                n102 = Divide(x=w257, y=180.0) -> (x/y=w255:dbl)
                                n103 = Bundle(cluster=w279, "flags"=w249, "Echo"=w264, "Radial distance"=w263, "Horizontal angle"=w262, "Vertical angle"=w255, "Echo pulse width"=w261, "Reserved"=w260) -> (w268:T11)
                              }
                              n104 = flat-sequence {
                                tunnel: w194 -> [w248]
                                tunnel: [w246] -> w192
                                frame #0 {
                                w247 = T13 {"Scan number"=0, "scanner status"=0, "Sync phase offset"=0, "Scan start time NTP"=0, "Scan end time NTP"=0, "Angle ticks per rotation"=0, "Start angle"=0.0, "End angle"=0.0, "Scan points"=0, "Mounting position yaw angle "=0.0, "Mounting position pitch angle"=0.0, "Mounting position roll angle"=0.0, "Mounting position x"=0.0, "Mounting position y"=0.0, "Mounting position z"=0.0, "Reserved"=0}  # Scan header
                                n105 = Unbundle(w248) -> ("Scan number"=w245:u16, "scanner status"=w244:u16, "Sync phase offset"=w243:u16, "Scan start time NTP"=w242:u64, "Scan end time NTP"=w241:u64, "Angle ticks per rotation"=w232:u16, "Start angle"=w238:i16, "End angle"=w237:i16, "Scan points"=w239:u16, "Mounting position yaw angle"=w236:i16, "Mounting position pitch angle"=w235:i16, "Mounting position roll angle"=w234:i16, "Mounting position x"=w223:i16, "Mounting position y"=w222:i16, "Mounting position z"=w221:i16, "Reserved"=w213:u16)
                                n106 = Build Array(w238, w237, w236, w235, w234) -> (w233:i16[])
                                n107 = Build Array(w223, w222, w221) -> (w220:i16[])
                                n108 = Divide(x=w233, y=w232) -> (x/y=w240:dbl[])
                                n109 = Multiply(x=w220, y=0.01) -> (x*y=w218:dbl[])
                                n110 = Multiply(x=w240, y=6.283185307179586) -> (x*y=w230:dbl[])
                                n111 = Index Array(array=w230, index #1=0 ("index")) -> (element #1=w228:dbl, element #2=w227:dbl, element #3=w226:dbl, element #4=w225:dbl, element #5=w224:dbl)  [unwired: 4 in]
                                n112 = Index Array(array=w218, index #1=0 ("index")) -> (element #1=w216:dbl, element #2=w215:dbl, element #3=w214:dbl)  [unwired: 2 in]
                                n113 = Bundle(cluster=w247, "Scan number"=w245, "scanner status"=w244, "Sync phase offset"=w243, "Scan start time NTP"=w242, "Scan end time NTP"=w241, "Angle ticks per rotation"=w232, "Start angle"=w228, "End angle"=w227, "Scan points"=w239, "Mounting position yaw angle"=w226, "Mounting position pitch angle"=w225, "Mounting position roll angle"=w224, "Mounting position x"=w216, "Mounting position y"=w215, "Mounting position z"=w214, "Reserved"=w213) -> (w246:T13)
                                }
                              }
                              n114 = Equal?(x=w189, y="") -> (x = y?=w190:bool)
                              n115 = case shown="True" w190 {
                                tunnel: w196 -> [_ w209]
                                tunnel: w193 -> [_ w207]
                                tunnel: w192 -> [_ w208]
                                frame False {
                                }
                                frame True {
                                n116 = Bundle By Name(cluster=T7 {"Header"={"Size of prev messages"=0, "Size of this messages"=0, "Reserved"=0, "DeviceID"=0, "Data type"=0, "NTP time"=0}, "Scan header"={"Scan number"=0, "scanner status"=0, "Sync phase offset"=0, "Scan start time NTP"=0, "Scan end time NTP"=0, "Angle ticks per rotation"=0, "Start angle"=0.0, "End angle"=0.0, "Scan points"=0, "Mounting position yaw angle "=0.0, "Mounting position pitch angle"=0.0, "Mounting position roll angle"=0.0, "Mounting position x"=0.0, "Mounting position y"=0.0, "Mounting position z"=0.0, "Reserved"=0}, "Scan points"=[]} ("output cluster"), "Header"=w209, "Scan header"=w208, "Scan points"=w207) -> (w205:T7)
                                n117 = Flatten To String(anything=w205, prepend array or string size? (T)=FALSE, byte order (0:big-endian, network order)=T5."native, host order") -> (data string=→"scan data 2202":string)  [unwired: 1 in, 2 out]
                                }
                              }
                            }
                            frame Disabled {
                            }
                          }
                        }
                        frame 8709 {
                          w299 = T14 {"Device ID "=0, "Scanner type"=0, "Scan number"=0, "Reserved 4"=0, "Start angle"=0.0, "End angle"=0.0, "Scan start time "=0, "Scan end time "=0, "Scan start time from device"=0, "Scan end time from device"=0, "Scan frequency"=0.0, "Beam tilt"=0.0, "scan flags"=0, "Yaw angle "=0.0, "Pitch angle "=0.0, "Roll angle"=0.0, "Offset x "=0.0, "Offset y"=0.0, "Offset z"=0.0, "Reserved 8 1"=0, "Reserved 8 2"=0, "Reserved 8 3"=0, "Reserved 8 4"=0, "Reserved 8 5"=0, "Reserved 8 6"=0, "Reserved 8 7"=0, "Reserved 8 8"=0}  # Scanner info
                          w301 = T15 {"NTP time"=20, "Scan end Time offset"=0, "flags"=0, "Scan number"=0, "Scan points"=0, "Number of Scan infos"=0, "reserved"=0, "reserved 2"=0}  # Scan header
                          n118 = String Subset(string=w307, length (rest)=24 ("length (rest)")) -> (substring=w314:string)  [unwired: 1 in]
                          n119 = Unflatten From String(type=w301, binary string=w314, data includes array or string size? (T)=FALSE, error in (no error)=w292) -> (value=w300:T15, error out=w291:errorcluster)  [unwired: 1 in, 1 out]
                          n120 = Unbundle By Name(w300) -> ("Number of Scan infos"=w311:u8, "Scan points"=w305:u16)
                          n121 = Multiply(x=w311, y=u8 148) -> (x*y=w309:u8)
                          n122 = String Subset(string=w307, offset (0)=24 ("length (rest)"), length (rest)=w309) -> (substring=w303:string)
                          n123 = Add(x=w309, y=u8 24) -> (x+y=w306:u8)
                          n124 = String Subset(string=w307, offset (0)=w306) -> (substring=w304:string)  [unwired: 1 in]
                          n125 = Unflatten From String(type=w299, binary string=w303, data includes array or string size? (T)=FALSE, error in (no error)=w291) -> (value=w297:T14, error out=w290:errorcluster)  [unwired: 1 in, 1 out]
                          n126 = for {
                            N: w305 -> [_]
                            shift-right: [w326] -> w295
                            shift-left: w304 -> [w327]
                            tunnel: [w323] -> w296 mode=indexing
                            shift-right: [w321] -> w289
                            shift-left: w290 -> [w322]
                            w324 = T16 {"X  position"=0.0, "Y  position"=0.0, "Z  position"=0.0, "Echo width"=0.0, "Device ID "=0, "Layer"=0, "Echo"=0, "Reserved"=0, "Timestamp"=0, "flags"=0, "Reserved 2"=0}  # Scan point
                            n127 = Unflatten From String(type=w324, binary string=w327, data includes array or string size? (T)=FALSE, error in (no error)=w322) -> (rest of the binary string=w326:string, value=w323:T16, error out=w321:errorcluster)  [unwired: 1 in]
                          }
                          n128 = Equal?(x=w295, y="") -> (x = y?=w293:bool)
                          n129 = case shown="True" w293 {
                            tunnel: w302 -> [_ w320]
                            tunnel: w300 -> [_ w319]
                            tunnel: w297 -> [_ w317]
                            tunnel: w296 -> [_ w316]
                            frame False {
                            }
                            frame True {
                              n130 = Bundle By Name(cluster=T8 {"Header"={"Size of prev messages"=20, "Size of this messages"=20, "Reserved"=20, "DeviceID"=20, "Data type"=20, "NTP time"=20}, "Scan header"={"NTP time"=20, "Scan end Time offset"=0, "flags"=0, "Scan number"=0, "Scan points"=0, "Number of Scan infos"=0, "reserved"=0, "reserved 2"=0}, "Scanner info"={"Device ID "=0, "Scanner type"=0, "Scan number"=0, "Reserved 4"=0, "Start angle"=0.0, "End angle"=0.0, "Scan start time "=0, "Scan end time "=0, "Scan start time from device"=0, "Scan end time from device"=0, "Scan frequency"=0.0, "Beam tilt"=0.0, "scan flags"=0, "Yaw angle "=0.0, "Pitch angle "=0.0, "Roll angle"=0.0, "Offset x "=0.0, "Offset y"=0.0, "Offset z"=0.0, "Reserved 8 1"=0, "Reserved 8 2"=0, "Reserved 8 3"=0, "Reserved 8 4"=0, "Reserved 8 5"=0, "Reserved 8 6"=0, "Reserved 8 7"=0, "Reserved 8 8"=0}, "Scan points"=[{"X  position"=10.364575, "Y  position"=7.7589917, "Z  position"=0.37767413, "Echo width"=1.3199999, "Device ID "=120, "Layer"=1, "Echo"=0, "Reserved"=0, "Timestamp"=0, "flags"=4, "Reserved 2"=0}, {"X  position"=10.398567, "Y  position"=7.661636, "Z  position"=0.3780232, "Echo width"=1.16, "Device ID "=120, "Layer"=1, "Echo"=0, "Reserved"=0, "Timestamp"=0, "flags"=20, "Reserved 2"=0}, {"X  position"=10.5718775, "Y  position"=7.7176, "Z  position"=0.23073287, "Echo width"=1.16, "Device ID "=120, "Layer"=0, "Echo"=0, "Reserved"=0, "Timestamp"=0, "flags"=1, "Reserved 2"=0}, {"X  position"=10.397608, "Y  position"=7.527418, "Z  position"=0.37872133, "Echo width"=1.56, "Device ID "=120, "Layer"=1, "Echo"=0, "Reserved"=0, "Timestamp"=0, "flags"=0, "Reserved 2"=0}, {"X  position"=10.454857, "Y  position"=7.4581714, "Z  position"=0.23638731, "Echo width"=1.0, "Device ID "=120, "Layer"=0, "Echo"=0, "Reserved"=0, "Timestamp"=0, "flags"=16, "Reserved 2"=0}, {"X  position"=10.401655, "Y  position"=7.4011188, "Z  position"=0.37934965, "Echo width"=1.4399999, "Device ID "=120, "Layer"=1, "Echo"=0, "Reserved"=0, "Timestamp"=0, "flags"=16, "Reserved 2"=0}, {"X  position"=10.595379, "Y  position"=7.4769697, "Z  position"=0.23408365, "Echo width"=1.24, "Device ID "=120, "Layer"=0, "Echo"=0, "Reserved"=0, "Timestamp"=0, "flags"=0, "Reserved 2"=0}, {"X  position"=10.417795, "Y  position"=7.289835, "Z  position"=0.37983832, "Echo width"=1.4399999, "Device ID "=120, "Layer"=1, "Echo"=0, "Reserved"=0, "Timestamp"=0, "flags"=0, "Reserved 2"=0}, {"X  position"=10.583961, "Y  position"=7.335657, "Z  position"=0.23638731, "Echo width"=1.0, "Device ID "=120, "Layer"=0, "Echo"=0, "Reserved"=0, "Timestamp"=0, "flags"=16, "Reserved 2"=0}, {"X  position"=10.474199, "Y  position"=7.221996, "Z  position"=0.37990814, "Echo width"=1.4399999, "Device ID "=120, "Layer"=1, "Echo"=0, "Reserved"=0, "Timestamp"=0, "flags"=16, "Reserved 2"=0}, {"X  position"=10.486532, "Y  position"=7.1095467, "Z  position"=0.24120408, "Echo width"=1.4399999, "Device ID "=120, "Layer"=0, "Echo"=0, "Reserved"=0, "Timestamp"=0, "flags"=0, "Reserved 2"=0}, {"X  position"=10.487894, "Y  position"=7.1109333, "Z  position"=0.38039684, "Echo width"=1.56, "Device ID "=120, "Layer"=1, "Echo"=0, "Reserved"=0, "Timestamp"=0, "flags"=0, "Reserved 2"=0}, {"X  position"=10.505892, "Y  position"=7.0058913, "Z  position"=0.24246061, "Echo width"=1.0799999, "Device ID "=120, "Layer"=0, "Echo"=0, "Reserved"=0, "Timestamp"=0, "flags"=16, "Reserved 2"=0}, {"X  position"=10.514328, "Y  position"=7.014328, "Z  position"=0.3807459, "Echo width"=1.48, "Device ID "=120, "Layer"=1, "Echo"=0, "Reserved"=0, "Timestamp"=0, "flags"=16, "Reserved 2"=0}, {"X  position"=10.652332, "Y  position"=7.028578, "Z  position"=0.23994753, "Echo width"=1.5999999, "Device ID "=120, "Layer"=0, "Echo"=0, "Reserved"=0, "Timestamp"=0, "flags"=0, "Reserved 2"=0}, {"X  position"=10.561007, "Y  position"=6.9388323, "Z  position"=0.3808855, "Echo width"=1.8, "Device ID "=120, "Layer"=1, "Echo"=0, "Reserved"=0, "Timestamp"=0, "flags"=0, "Reserved 2"=0}, {"X  position"=10.634285, "Y  position"=6.8894997, "Z  position"=0.24225119, "Echo width"=0.88, "Device ID "=120, "Layer"=0, "Echo"=0, "Reserved"=0, "Timestamp"=0, "flags"=16, "Reserved 2"=0}, {"X  position"=10.592518, "Y  position"=6.8491645, "Z  position"=0.38116476, "Echo width"=1.8, "Device ID "=120, "Layer"=1, "Echo"=0, "Reserved"=0, "Timestamp"=0, "flags"=16, "Reserved 2"=0}, {"X  position"=10.657875, "Y  position"=6.792569, "Z  position"=0.2432983, "Echo width"=1.64, "Device ID "=120, "Layer"=0, "Echo"=0, "Reserved"=0, "Timestamp"=0, "flags"=0, "Reserved 2"=0}, {"X  position"=10.623003, "Y  position"=6.7594767, "Z  position"=0.381444, "Echo width"=1.68, "Device ID "=120, "Layer"=1, "Echo"=0, "Reserved"=0, "Timestamp"=0, "flags"=0, "Reserved 2"=0}, {"X  position"=10.72419, "Y  position"=6.736666, "Z  position"=0.24308887, "Echo width"=1.24, "Device ID "=120, "Layer"=0, "Echo"=0, "Reserved"=0, "Timestamp"=0, "flags"=16, "Reserved 2"=0}, {"X  position"=10.754852, "Y  position"=6.765259, "Z  position"=0.3807459, "Echo width"=1.48, "Device ID "=120, "Layer"=1, "Echo"=0, "Reserved"=0, "Timestamp"=0, "flags"=16, "Reserved 2"=0}, {"X  position"=10.797444, "Y  position"=6.686876, "Z  position"=0.24267004, "Echo width"=1.56, "Device ID "=120, "Layer"=0, "Echo"=0, "Reserved"=0, "Timestamp"=0, "flags"=0, "Reserved 2"=0}, {"X  position"=10.857848, "Y  position"=6.7422256, "Z  position"=0.38032702, "Echo width"=1.5999999, "Device ID "=120, "Layer"=1, "Echo"=0, "Reserved"=0, "Timestamp"=0, "flags"=0, "Reserved 2"=0}, {"X  position"=10.929818, "Y  position"=6.6898384, "Z  position"=0.24057579, "Echo width"=1.24, "Device ID "=120, "Layer"=0, "Echo"=0, "Reserved"=0, "Timestamp"=0, "flags"=16, "Reserved 2"=0}, {"X  position"=10.931267, "Y  position"=6.691143, "Z  position"=0.3801874, "Echo width"=1.48, "Device ID "=120, "Layer"=1, "Echo"=0, "Reserved"=0, "Timestamp"=0, "flags"=16, "Reserved 2"=0}, {"X  position"=11.032841, "Y  position"=6.6644955, "Z  position"=0.23931925, "Echo width"=1.52, "Device ID "=120, "Layer"=0, "Echo"=0, "Reserved"=0, "Timestamp"=0, "flags"=0, "Reserved 2"=0}, {"X  position"=11.0792465, "Y  position"=6.705551, "Z  position"=0.37934965, "Echo width"=1.36, "Device ID "=120, "Layer"=1, "Echo"=0, "Reserved"=0, "Timestamp"=0, "flags"=0, "Reserved 2"=0}, {"X  position"=11.256713, "Y  position"=6.7428074, "Z  position"=0.23471192, "Echo width"=1.0, "Device ID "=120, "Layer"=0, "Echo"=0, "Reserved"=0, "Timestamp"=0, "flags"=16, "Reserved 2"=0}, {"X  position"=11.190304, "Y  position"=6.6850786, "Z  position"=0.37886095, "Echo width"=1.3199999, "Device ID "=120, "Layer"=1, "Echo"=0, "Reserved"=0, "Timestamp"=0, "flags"=16, "Reserved 2"=0}, {"X  position"=11.490114, "Y  position"=6.8242025, "Z  position"=0.22989514, "Echo width"=1.64, "Device ID "=120, "Layer"=0, "Echo"=0, "Reserved"=0, "Timestamp"=0, "flags"=0, "Reserved 2"=0}, {"X  position"=11.324387, "Y  position"=6.682658, "Z  position"=0.37816283, "Echo width"=1.88, "Device ID "=120, "Layer"=1, "Echo"=0, "Reserved"=0, "Timestamp"=0, "flags"=0, "Reserved 2"=0}, {"X  position"=11.579996, "Y  position"=6.779922, "Z  position"=0.22905746, "Echo width"=1.0799999, "Device ID "=120, "Layer"=0, "Echo"=0, "Reserved"=0, "Timestamp"=0, "flags"=16, "Reserved 2"=0}, {"X  position"=11.497309, "Y  position"=6.710539, "Z  position"=0.37711564, "Echo width"=1.48, "Device ID "=120, "Layer"=1, "Echo"=0, "Reserved"=0, "Timestamp"=0, "flags"=16, "Reserved 2"=0}, {"X  position"=11.661998, "Y  position"=6.728232, "Z  position"=0.22842918, "Echo width"=1.52, "Device ID "=120, "Layer"=0, "Echo"=0, "Reserved"=0, "Timestamp"=0, "flags"=0, "Reserved 2"=0}, {"X  position"=11.748466, "Y  position"=6.7995105, "Z  position"=0.37537032, "Echo width"=1.48, "Device ID "=120, "Layer"=1, "Echo"=0, "Reserved"=0, "Timestamp"=0, "flags"=0, "Reserved 2"=0}, {"X  position"=11.767018, "Y  position"=6.6945, "Z  position"=0.22717266, "Echo width"=1.0, "Device ID "=120, "Layer"=0, "Echo"=0, "Reserved"=0, "Timestamp"=0, "flags"=16, "Reserved 2"=0}, {"X  position"=11.7919445, "Y  position"=6.7146845, "Z  position"=0.37550995, "Echo width"=1.1999999, "Device ID "=120, "Layer"=1, "Echo"=0, "Reserved"=0, "Timestamp"=0, "flags"=16, "Reserved 2"=0}, {"X  position"=11.926841, "Y  position"=6.703012, "Z  position"=0.22445014, "Echo width"=1.4399999, "Device ID "=120, "Layer"=0, "Echo"=0, "Reserved"=0, "Timestamp"=0, "flags"=0, "Reserved 2"=0}, {"X  position"=10.903293, "Y  position"=5.888845, "Z  position"=0.38395727, "Echo width"=1.76, "Device ID "=120, "Layer"=1, "Echo"=0, "Reserved"=0, "Timestamp"=0, "flags"=0, "Reserved 2"=1}, {"X  position"=10.93719, "Y  position"=5.81057, "Z  position"=0.25230354, "Echo width"=1.24, "Device ID "=120, "Layer"=0, "Echo"=0, "Reserved"=0, "Timestamp"=0, "flags"=16, "Reserved 2"=1}, {"X  position"=10.820442, "Y  position"=5.719356, "Z  position"=0.38514408, "Echo width"=1.5999999, "Device ID "=120, "Layer"=1, "Echo"=0, "Reserved"=0, "Timestamp"=0, "flags"=16, "Reserved 2"=1}, {"X  position"=11.011408, "Y  position"=5.7637057, "Z  position"=0.2516753, "Echo width"=1.88, "Device ID "=120, "Layer"=0, "Echo"=0, "Reserved"=0, "Timestamp"=0, "flags"=0, "Reserved 2"=1}, {"X  position"=10.751072, "Y  position"=5.5639434, "Z  position"=0.38619128, "Echo width"=1.7199999, "Device ID "=120, "Layer"=1, "Echo"=0, "Reserved"=0, "Timestamp"=0, "flags"=0, "Reserved 2"=1}, {"X  position"=10.901727, "Y  position"=5.5776014, "Z  position"=0.2558638, "Echo width"=1.68, "Device ID "=120, "Layer"=0, "Echo"=0, "Reserved"=0, "Timestamp"=0, "flags"=16, "Reserved 2"=1}, {"X  position"=10.815323, "Y  position"=5.512491, "Z  position"=0.38605165, "Echo width"=1.68, "Device ID "=120, "Layer"=1, "Echo"=0, "Reserved"=0, "Timestamp"=0, "flags"=16, "Reserved 2"=1}, {"X  position"=10.853677, "Y  position"=5.441435, "Z  position"=0.25837684, "Echo width"=1.9599999, "Device ID "=120, "Layer"=0, "Echo"=0, "Reserved"=0, "Timestamp"=0, "flags"=0, "Reserved 2"=1}, {"X  position"=10.718458, "Y  position"=5.341378, "Z  position"=0.38730827, "Echo width"=1.7199999, "Device ID "=120, "Layer"=1, "Echo"=0, "Reserved"=0, "Timestamp"=0, "flags"=0, "Reserved 2"=1}, {"X  position"=10.771467, "Y  position"=5.28303, "Z  position"=0.26172763, "Echo width"=1.52, "Device ID "=120, "Layer"=0, "Echo"=0, "Reserved"=0, "Timestamp"=0, "flags"=16, "Reserved 2"=1}, {"X  position"=10.756706, "Y  position"=5.2723055, "Z  position"=0.3873781, "Echo width"=1.64, "Device ID "=120, "Layer"=1, "Echo"=0, "Reserved"=0, "Timestamp"=0, "flags"=16, "Reserved 2"=1}, {"X  position"=7.138298, "Y  position"=2.595173, "Z  position"=0.35638738, "Echo width"=1.88, "Device ID "=120, "Layer"=0, "Echo"=0, "Reserved"=0, "Timestamp"=0, "flags"=0, "Reserved 2"=2}, {"X  position"=7.1634307, "Y  position"=2.6130996, "Z  position"=0.41858432, "Echo width"=2.44, "Device ID "=120, "Layer"=1, "Echo"=0, "Reserved"=0, "Timestamp"=0, "flags"=0, "Reserved 2"=2}, {"X  position"=7.150298, "Y  position"=2.579776, "Z  position"=0.4812062, "Echo width"=2.1599998, "Device ID "=120, "Layer"=2, "Echo"=0, "Reserved"=0, "Timestamp"=0, "flags"=0, "Reserved 2"=2}, {"X  position"=7.0679407, "Y  position"=2.5215714, "Z  position"=0.54151833, "Echo width"=1.3199999, "Device ID "=120, "Layer"=3, "Echo"=0, "Reserved"=0, "Timestamp"=0, "flags"=0, "Reserved 2"=2}, {"X  position"=7.324601, "Y  position"=2.6780145, "Z  position"=0.3521989, "Echo width"=1.7199999, "Device ID "=120, "Layer"=0, "Echo"=0, "Reserved"=0, "Timestamp"=0, "flags"=17, "Reserved 2"=0}, {"X  position"=7.169712, "Y  position"=2.5695598, "Z  position"=0.41872394, "Echo width"=5.12, "Device ID "=120, "Layer"=1, "Echo"=0, "Reserved"=0, "Timestamp"=0, "flags"=16, "Reserved 2"=2}, {"X  position"=7.164456, "Y  position"=2.5421236, "Z  position"=0.4811364, "Echo width"=2.28, "Device ID "=120, "Layer"=2, "Echo"=0, "Reserved"=0, "Timestamp"=0, "flags"=16, "Reserved 2"=2}, {"X  position"=7.0980244, "Y  position"=2.4960382, "Z  position"=0.5417278, "Echo width"=1.52, "Device ID "=120, "Layer"=3, "Echo"=0, "Reserved"=0, "Timestamp"=0, "flags"=16, "Reserved 2"=2}, {"X  position"=7.3560643, "Y  position"=2.6501997, "Z  position"=0.35198948, "Echo width"=1.7199999, "Device ID "=120, "Layer"=0, "Echo"=0, "Reserved"=0, "Timestamp"=0, "flags"=1, "Reserved 2"=0}, {"X  position"=7.2002363, "Y  position"=2.5431018, "Z  position"=0.41865414, "Echo width"=6.2, "Device ID "=120, "Layer"=1, "Echo"=0, "Reserved"=0, "Timestamp"=0, "flags"=0, "Reserved 2"=2}, {"X  position"=7.2030315, "Y  position"=2.5213046, "Z  position"=0.48127604, "Echo width"=2.24, "Device ID "=120, "Layer"=2, "Echo"=0, "Reserved"=0, "Timestamp"=0, "flags"=0, "Reserved 2"=2}, {"X  position"=7.1609893, "Y  position"=2.4926789, "Z  position"=0.5427749, "Echo width"=1.5999999, "Device ID "=120, "Layer"=3, "Echo"=0, "Reserved"=0, "Timestamp"=0, "flags"=0, "Reserved 2"=2}, {"X  position"=6.9977713, "Y  position"=2.3592765, "Z  position"=0.361623, "Echo width"=0.39999998, "Device ID "=120, "Layer"=0, "Echo"=0, "Reserved"=0, "Timestamp"=0, "flags"=4113, "Reserved 2"=0}, {"X  position"=10.818796, "Y  position"=4.9365907, "Z  position"=0.26507843, "Echo width"=1.52, "Device ID "=120, "Layer"=0, "Echo"=1, "Reserved"=0, "Timestamp"=0, "flags"=16, "Reserved 2"=1}, {"X  position"=7.2388678, "Y  position"=2.5218985, "Z  position"=0.4185145, "Echo width"=1.92, "Device ID "=120, "Layer"=1, "Echo"=0, "Reserved"=0, "Timestamp"=0, "flags"=4112, "Reserved 2"=2}, {"X  position"=10.795353, "Y  position"=4.9207783, "Z  position"=0.38856488, "Echo width"=1.48, "Device ID "=120, "Layer"=1, "Echo"=1, "Reserved"=0, "Timestamp"=0, "flags"=16, "Reserved 2"=1}, {"X  position"=7.216578, "Y  position"=2.483338, "Z  position"=0.4812062, "Echo width"=1.24, "Device ID "=120, "Layer"=2, "Echo"=0, "Reserved"=0, "Timestamp"=0, "flags"=16, "Reserved 2"=2}, {"X  position"=7.2574186, "Y  position"=2.5106268, "Z  position"=0.54465973, "Echo width"=1.04, "Device ID "=120, "Layer"=3, "Echo"=0, "Reserved"=0, "Timestamp"=0, "flags"=16, "Reserved 2"=2}, {"X  position"=10.894945, "Y  position"=4.894607, "Z  position"=0.26424074, "Echo width"=1.8399999, "Device ID "=120, "Layer"=0, "Echo"=0, "Reserved"=0, "Timestamp"=0, "flags"=0, "Reserved 2"=1}, {"X  position"=7.2440557, "Y  position"=2.4781363, "Z  position"=0.41865414, "Echo width"=1.0, "Device ID "=120, "Layer"=1, "Echo"=0, "Reserved"=0, "Timestamp"=0, "flags"=4096, "Reserved 2"=2}, {"X  position"=10.804662, "Y  position"=4.8348503, "Z  position"=0.38884413, "Echo width"=1.9599999, "Device ID "=120, "Layer"=1, "Echo"=1, "Reserved"=0, "Timestamp"=0, "flags"=0, "Reserved 2"=1}, {"X  position"=10.900951, "Y  position"=4.852277, "Z  position"=0.51178414, "Echo width"=1.52, "Device ID "=120, "Layer"=2, "Echo"=0, "Reserved"=0, "Timestamp"=0, "flags"=0, "Reserved 2"=1}, {"X  position"=10.932953, "Y  position"=4.873257, "Z  position"=0.6361781, "Echo width"=1.36, "Device ID "=120, "Layer"=3, "Echo"=0, "Reserved"=0, "Timestamp"=0, "flags"=0, "Reserved 2"=1}, {"X  position"=10.903836, "Y  position"=4.808108, "Z  position"=0.26507843, "Echo width"=1.68, "Device ID "=120, "Layer"=0, "Echo"=0, "Reserved"=0, "Timestamp"=0, "flags"=16, "Reserved 2"=1}, {"X  position"=10.813029, "Y  position"=4.749137, "Z  position"=0.3891234, "Echo width"=1.8399999, "Device ID "=120, "Layer"=1, "Echo"=0, "Reserved"=0, "Timestamp"=0, "flags"=16, "Reserved 2"=1}, {"X  position"=10.934604, "Y  position"=4.782098, "Z  position"=0.51171434, "Echo width"=1.4, "Device ID "=120, "Layer"=2, "Echo"=0, "Reserved"=0, "Timestamp"=0, "flags"=16, "Reserved 2"=1}, {"X  position"=10.966789, "Y  position"=4.8028, "Z  position"=0.6359687, "Echo width"=1.04, "Device ID "=120, "Layer"=3, "Echo"=0, "Reserved"=0, "Timestamp"=0, "flags"=16, "Reserved 2"=1}, {"X  position"=10.996104, "Y  position"=4.7755456, "Z  position"=0.2638219, "Echo width"=2.08, "Device ID "=120, "Layer"=0, "Echo"=0, "Reserved"=0, "Timestamp"=0, "flags"=0, "Reserved 2"=1}, {"X  position"=10.854195, "Y  position"=4.6851387, "Z  position"=0.3891234, "Echo width"=1.9599999, "Device ID "=120, "Layer"=1, "Echo"=0, "Reserved"=0, "Timestamp"=0, "flags"=0, "Reserved 2"=1}, {"X  position"=10.959137, "Y  position"=4.7063656, "Z  position"=0.5115747, "Echo width"=1.64, "Device ID "=120, "Layer"=2, "Echo"=0, "Reserved"=0, "Timestamp"=0, "flags"=0, "Reserved 2"=1}, {"X  position"=10.966139, "Y  position"=4.7107825, "Z  position"=0.63492155, "Echo width"=1.52, "Device ID "=120, "Layer"=3, "Echo"=0, "Reserved"=0, "Timestamp"=0, "flags"=0, "Reserved 2"=1}, {"X  position"=10.918794, "Y  position"=4.635777, "Z  position"=0.26675382, "Echo width"=1.64, "Device ID "=120, "Layer"=0, "Echo"=0, "Reserved"=0, "Timestamp"=0, "flags"=16, "Reserved 2"=1}, {"X  position"=10.894799, "Y  position"=4.6207833, "Z  position"=0.3891234, "Echo width"=1.8399999, "Device ID "=120, "Layer"=1, "Echo"=0, "Reserved"=0, "Timestamp"=0, "flags"=16, "Reserved 2"=1}, {"X  position"=10.965911, "Y  position"=4.6200457, "Z  position"=0.51129544, "Echo width"=1.56, "Device ID "=120, "Layer"=2, "Echo"=0, "Reserved"=0, "Timestamp"=0, "flags"=16, "Reserved 2"=1}, {"X  position"=10.98996, "Y  position"=4.6349277, "Z  position"=0.6345027, "Echo width"=1.24, "Device ID "=120, "Layer"=3, "Echo"=0, "Reserved"=0, "Timestamp"=0, "flags"=16, "Reserved 2"=1}, {"X  position"=10.958965, "Y  position"=4.57086, "Z  position"=0.26675382, "Echo width"=1.88, "Device ID "=120, "Layer"=0, "Echo"=0, "Reserved"=0, "Timestamp"=0, "flags"=0, "Reserved 2"=1}, {"X  position"=10.968946, "Y  position"=4.576976, "Z  position"=0.38884413, "Echo width"=1.9599999, "Device ID "=120, "Layer"=1, "Echo"=0, "Reserved"=0, "Timestamp"=0, "flags"=0, "Reserved 2"=1}, {"X  position"=11.014492, "Y  position"=4.5599055, "Z  position"=0.5113653, "Echo width"=1.8, "Device ID "=120, "Layer"=2, "Echo"=0, "Reserved"=0, "Timestamp"=0, "flags"=0, "Reserved 2"=1}, {"X  position"=11.081405, "Y  position"=4.6005096, "Z  position"=0.63575923, "Echo width"=1.64, "Device ID "=120, "Layer"=3, "Echo"=0, "Reserved"=0, "Timestamp"=0, "flags"=0, "Reserved 2"=1}, {"X  position"=10.9985695, "Y  position"=4.505595, "Z  position"=0.26675382, "Echo width"=1.64, "Device ID "=120, "Layer"=0, "Echo"=0, "Reserved"=0, "Timestamp"=0, "flags"=16, "Reserved 2"=1}, {"X  position"=11.025745, "Y  position"=4.5219245, "Z  position"=0.38870454, "Echo width"=1.8, "Device ID "=120, "Layer"=1, "Echo"=0, "Reserved"=0, "Timestamp"=0, "flags"=16, "Reserved 2"=1}, {"X  position"=11.045404, "Y  position"=4.489044, "Z  position"=0.51129544, "Echo width"=1.56, "Device ID "=120, "Layer"=2, "Echo"=0, "Reserved"=0, "Timestamp"=0, "flags"=16, "Reserved 2"=1}, {"X  position"=11.104078, "Y  position"=4.5239515, "Z  position"=0.6353404, "Echo width"=1.1999999, "Device ID "=120, "Layer"=3, "Echo"=0, "Reserved"=0, "Timestamp"=0, "flags"=16, "Reserved 2"=1}, {"X  position"=11.080673, "Y  position"=4.4653583, "Z  position"=0.2657067, "Echo width"=1.76, "Device ID "=120, "Layer"=0, "Echo"=0, "Reserved"=0, "Timestamp"=0, "flags"=0, "Reserved 2"=1}, {"X  position"=11.090767, "Y  position"=4.471304, "Z  position"=0.3884951, "Echo width"=1.88, "Device ID "=120, "Layer"=1, "Echo"=0, "Reserved"=0, "Timestamp"=0, "flags"=0, "Reserved 2"=1}, {"X  position"=11.162034, "Y  position"=4.468366, "Z  position"=0.5119238, "Echo width"=1.8, "Device ID "=120, "Layer"=2, "Echo"=0, "Reserved"=0, "Timestamp"=0, "flags"=0, "Reserved 2"=1}, {"X  position"=11.229632, "Y  position"=4.507788, "Z  position"=0.63743466, "Echo width"=1.56, "Device ID "=120, "Layer"=3, "Echo"=0, "Reserved"=0, "Timestamp"=0, "flags"=4096, "Reserved 2"=1}, {"X  position"=14.580579, "Y  position"=6.4620023, "Z  position"=0.71869123, "Echo width"=1.16, "Device ID "=120, "Layer"=3, "Echo"=1, "Reserved"=0, "Timestamp"=0, "flags"=4, "Reserved 2"=0}, {"X  position"=11.17996, "Y  position"=4.434027, "Z  position"=0.26424074, "Echo width"=1.52, "Device ID "=120, "Layer"=0, "Echo"=0, "Reserved"=0, "Timestamp"=0, "flags"=16, "Reserved 2"=1}, {"X  position"=11.224758, "Y  position"=4.4598913, "Z  position"=0.38772714, "Echo width"=1.68, "Device ID "=120, "Layer"=1, "Echo"=0, "Reserved"=0, "Timestamp"=0, "flags"=16, "Reserved 2"=1}, {"X  position"=11.261507, "Y  position"=4.436067, "Z  position"=0.5124124, "Echo width"=1.56, "Device ID "=120, "Layer"=2, "Echo"=0, "Reserved"=0, "Timestamp"=0, "flags"=16, "Reserved 2"=1}, {"X  position"=11.277355, "Y  position"=4.4451246, "Z  position"=0.63764405, "Echo width"=1.0, "Device ID "=120, "Layer"=3, "Echo"=0, "Reserved"=0, "Timestamp"=0, "flags"=16, "Reserved 2"=1}, {"X  position"=11.331483, "Y  position"=4.43084, "Z  position"=0.2615182, "Echo width"=1.76, "Device ID "=120, "Layer"=0, "Echo"=0, "Reserved"=0, "Timestamp"=0, "flags"=0, "Reserved 2"=1}, {"X  position"=11.376528, "Y  position"=4.456325, "Z  position"=0.3868196, "Echo width"=1.8399999, "Device ID "=120, "Layer"=1, "Echo"=0, "Reserved"=0, "Timestamp"=0, "flags"=0, "Reserved 2"=1}, {"X  position"=11.40462, "Y  position"=4.4268003, "Z  position"=0.51325023, "Echo width"=1.3199999, "Device ID "=120, "Layer"=2, "Echo"=0, "Reserved"=0, "Timestamp"=0, "flags"=0, "Reserved 2"=1}, {"X  position"=11.4205265, "Y  position"=4.435708, "Z  position"=0.64015716, "Echo width"=1.24, "Device ID "=120, "Layer"=3, "Echo"=0, "Reserved"=0, "Timestamp"=0, "flags"=0, "Reserved 2"=1}, {"X  position"=11.6409235, "Y  position"=4.512587, "Z  position"=0.25502607, "Echo width"=1.8, "Device ID "=120, "Layer"=0, "Echo"=0, "Reserved"=0, "Timestamp"=0, "flags"=16, "Reserved 2"=1}, {"X  position"=11.581289, "Y  position"=4.479532, "Z  position"=0.38549316, "Echo width"=1.52, "Device ID "=120, "Layer"=1, "Echo"=0, "Reserved"=0, "Timestamp"=0, "flags"=16, "Reserved 2"=1}, {"X  position"=11.556922, "Y  position"=4.420179, "Z  position"=0.5141578, "Echo width"=1.0799999, "Device ID "=120, "Layer"=2, "Echo"=0, "Reserved"=0, "Timestamp"=0, "flags"=16, "Reserved 2"=1}, {"X  position"=11.546586, "Y  position"=4.4145083, "Z  position"=0.6422514, "Echo width"=1.48, "Device ID "=120, "Layer"=3, "Echo"=0, "Reserved"=0, "Timestamp"=0, "flags"=16, "Reserved 2"=1}, {"X  position"=11.8908615, "Y  position"=4.5558667, "Z  position"=0.24999988, "Echo width"=1.8399999, "Device ID "=120, "Layer"=0, "Echo"=0, "Reserved"=0, "Timestamp"=0, "flags"=0, "Reserved 2"=1}, {"X  position"=11.743103, "Y  position"=4.4756403, "Z  position"=0.38451576, "Echo width"=1.5999999, "Device ID "=120, "Layer"=1, "Echo"=0, "Reserved"=0, "Timestamp"=0, "flags"=0, "Reserved 2"=1}, {"X  position"=11.718511, "Y  position"=4.415965, "Z  position"=0.51513517, "Echo width"=1.52, "Device ID "=120, "Layer"=2, "Echo"=0, "Reserved"=0, "Timestamp"=0, "flags"=0, "Reserved 2"=1}, {"X  position"=11.7169075, "Y  position"=4.415104, "Z  position"=0.6453928, "Echo width"=1.4, "Device ID "=120, "Layer"=3, "Echo"=0, "Reserved"=0, "Timestamp"=0, "flags"=0, "Reserved 2"=1}, {"X  position"=11.8243685, "Y  position"=4.4261456, "Z  position"=0.252513, "Echo width"=1.56, "Device ID "=120, "Layer"=0, "Echo"=0, "Reserved"=0, "Timestamp"=0, "flags"=16, "Reserved 2"=1}, {"X  position"=11.896626, "Y  position"=4.4645658, "Z  position"=0.3836082, "Echo width"=1.4, "Device ID "=120, "Layer"=1, "Echo"=0, "Reserved"=0, "Timestamp"=0, "flags"=16, "Reserved 2"=1}, {"X  position"=12.004568, "Y  position"=4.427198, "Z  position"=0.24916218, "Echo width"=1.92, "Device ID "=120, "Layer"=0, "Echo"=0, "Reserved"=0, "Timestamp"=0, "flags"=0, "Reserved 2"=1}, {"X  position"=12.032836, "Y  position"=4.4419136, "Z  position"=0.38284028, "Echo width"=1.8, "Device ID "=120, "Layer"=1, "Echo"=0, "Reserved"=0, "Timestamp"=0, "flags"=0, "Reserved 2"=1}, {"X  position"=12.132146, "Y  position"=4.4458475, "Z  position"=0.51778805, "Echo width"=1.76, "Device ID "=120, "Layer"=2, "Echo"=0, "Reserved"=0, "Timestamp"=0, "flags"=0, "Reserved 2"=1}, {"X  position"=12.388221, "Y  position"=4.577735, "Z  position"=0.6594242, "Echo width"=1.1999999, "Device ID "=120, "Layer"=3, "Echo"=0, "Reserved"=0, "Timestamp"=0, "flags"=4100, "Reserved 2"=0}, {"X  position"=14.379183, "Y  position"=5.6031475, "Z  position"=0.7063352, "Echo width"=1.1999999, "Device ID "=120, "Layer"=3, "Echo"=1, "Reserved"=0, "Timestamp"=0, "flags"=4, "Reserved 2"=0}, {"X  position"=12.185409, "Y  position"=4.425437, "Z  position"=0.2458114, "Echo width"=1.5999999, "Device ID "=120, "Layer"=0, "Echo"=0, "Reserved"=0, "Timestamp"=0, "flags"=16, "Reserved 2"=1}, {"X  position"=12.231651, "Y  position"=4.4489985, "Z  position"=0.38158363, "Echo width"=1.68, "Device ID "=120, "Layer"=1, "Echo"=0, "Reserved"=0, "Timestamp"=0, "flags"=16, "Reserved 2"=1}, {"X  position"=12.331346, "Y  position"=4.451365, "Z  position"=0.51904464, "Echo width"=1.48, "Device ID "=120, "Layer"=2, "Echo"=0, "Reserved"=0, "Timestamp"=0, "flags"=16, "Reserved 2"=1}, {"X  position"=16.311438, "Y  position"=6.457496, "Z  position"=0.7505237, "Echo width"=1.5999999, "Device ID "=120, "Layer"=3, "Echo"=0, "Reserved"=0, "Timestamp"=0, "flags"=16, "Reserved 2"=3}, {"X  position"=12.402644, "Y  position"=4.4386945, "Z  position"=0.24162291, "Echo width"=1.88, "Device ID "=120, "Layer"=0, "Echo"=0, "Reserved"=0, "Timestamp"=0, "flags"=0, "Reserved 2"=1}, {"X  position"=12.422277, "Y  position"=4.4484835, "Z  position"=0.38039684, "Echo width"=1.8399999, "Device ID "=120, "Layer"=1, "Echo"=0, "Reserved"=0, "Timestamp"=0, "flags"=0, "Reserved 2"=1}, {"X  position"=12.52232, "Y  position"=4.449316, "Z  position"=0.5202315, "Echo width"=1.7199999, "Device ID "=120, "Layer"=2, "Echo"=0, "Reserved"=0, "Timestamp"=0, "flags"=0, "Reserved 2"=1}, {"X  position"=12.726796, "Y  position"=4.550153, "Z  position"=0.6654975, "Echo width"=0.71999997, "Device ID "=120, "Layer"=3, "Echo"=0, "Reserved"=0, "Timestamp"=0, "flags"=4100, "Reserved 2"=0}, {"X  position"=15.049188, "Y  position"=5.6954293, "Z  position"=0.71973836, "Echo width"=3.52, "Device ID "=120, "Layer"=3, "Echo"=1, "Reserved"=0, "Timestamp"=0, "flags"=4, "Reserved 2"=0}, {"X  position"=10.706747, "Y  position"=3.5149653, "Z  position"=0.2820418, "Echo width"=0.64, "Device ID "=120, "Layer"=0, "Echo"=0, "Reserved"=0, "Timestamp"=0, "flags"=16, "Reserved 2"=4}, {"X  position"=10.824993, "Y  position"=3.572638, "Z  position"=0.3931027, "Echo width"=1.12, "Device ID "=120, "Layer"=1, "Echo"=0, "Reserved"=0, "Timestamp"=0, "flags"=16, "Reserved 2"=4}, {"X  position"=15.809844, "Y  position"=5.9375644, "Z  position"=0.7362828, "Echo width"=0.32, "Device ID "=120, "Layer"=3, "Echo"=0, "Reserved"=0, "Timestamp"=0, "flags"=18, "Reserved 2"=5}, {"X  position"=10.619836, "Y  position"=3.3959877, "Z  position"=0.2847643, "Echo width"=1.48, "Device ID "=120, "Layer"=0, "Echo"=0, "Reserved"=0, "Timestamp"=0, "flags"=0, "Reserved 2"=4}, {"X  position"=10.729532, "Y  position"=3.44831, "Z  position"=0.3940801, "Echo width"=1.52, "Device ID "=120, "Layer"=1, "Echo"=0, "Reserved"=0, "Timestamp"=0, "flags"=0, "Reserved 2"=4}, {"X  position"=10.771641, "Y  position"=3.429529, "Z  position"=0.5061293, "Echo width"=1.48, "Device ID "=120, "Layer"=2, "Echo"=0, "Reserved"=0, "Timestamp"=0, "flags"=0, "Reserved 2"=4}, {"X  position"=11.005331, "Y  position"=3.5397441, "Z  position"=0.6238221, "Echo width"=1.48, "Device ID "=120, "Layer"=3, "Echo"=0, "Reserved"=0, "Timestamp"=0, "flags"=4, "Reserved 2"=0}, {"X  position"=10.56765, "Y  position"=3.2956994, "Z  position"=0.2866491, "Echo width"=1.24, "Device ID "=120, "Layer"=0, "Echo"=0, "Reserved"=0, "Timestamp"=0, "flags"=16, "Reserved 2"=4}, {"X  position"=10.677782, "Y  position"=3.347055, "Z  position"=0.3947084, "Echo width"=1.4399999, "Device ID "=120, "Layer"=1, "Echo"=0, "Reserved"=0, "Timestamp"=0, "flags"=16, "Reserved 2"=4}, {"X  position"=10.665075, "Y  position"=3.303145, "Z  position"=0.50508213, "Echo width"=0.84, "Device ID "=120, "Layer"=2, "Echo"=0, "Reserved"=0, "Timestamp"=0, "flags"=16, "Reserved 2"=4}, {"X  position"=10.623434, "Y  position"=3.246336, "Z  position"=0.28602085, "Echo width"=1.5999999, "Device ID "=120, "Layer"=0, "Echo"=0, "Reserved"=0, "Timestamp"=0, "flags"=0, "Reserved 2"=4}, {"X  position"=10.606625, "Y  position"=3.2386756, "Z  position"=0.39547634, "Echo width"=1.56, "Device ID "=120, "Layer"=1, "Echo"=0, "Reserved"=0, "Timestamp"=0, "flags"=0, "Reserved 2"=4}, {"X  position"=10.7027445, "Y  position"=3.2445998, "Z  position"=0.5051519, "Echo width"=1.28, "Device ID "=120, "Layer"=2, "Echo"=0, "Reserved"=0, "Timestamp"=0, "flags"=0, "Reserved 2"=4}, {"X  position"=10.929232, "Y  position"=3.3466246, "Z  position"=0.6206807, "Echo width"=1.56, "Device ID "=120, "Layer"=3, "Echo"=0, "Reserved"=0, "Timestamp"=0, "flags"=4, "Reserved 2"=0}, {"X  position"=10.560158, "Y  position"=3.1433845, "Z  position"=0.28811508, "Echo width"=1.3199999, "Device ID "=120, "Layer"=0, "Echo"=0, "Reserved"=0, "Timestamp"=0, "flags"=16, "Reserved 2"=4}, {"X  position"=10.625481, "Y  position"=3.1724684, "Z  position"=0.39554617, "Echo width"=1.52, "Device ID "=120, "Layer"=1, "Echo"=0, "Reserved"=0, "Timestamp"=0, "flags"=16, "Reserved 2"=4}, {"X  position"=10.611797, "Y  position"=3.1292655, "Z  position"=0.5042444, "Echo width"=0.68, "Device ID "=120, "Layer"=2, "Echo"=0, "Reserved"=0, "Timestamp"=0, "flags"=16, "Reserved 2"=4}, {"X  position"=10.541476, "Y  position"=3.061721, "Z  position"=0.28916222, "Echo width"=1.7199999, "Device ID "=120, "Layer"=0, "Echo"=0, "Reserved"=0, "Timestamp"=0, "flags"=0, "Reserved 2"=4}, {"X  position"=10.533679, "Y  position"=3.0583308, "Z  position"=0.39645374, "Echo width"=2.0, "Device ID "=120, "Layer"=1, "Echo"=0, "Reserved"=0, "Timestamp"=0, "flags"=0, "Reserved 2"=4}, {"X  position"=10.684772, "Y  position"=3.0868218, "Z  position"=0.50459343, "Echo width"=1.64, "Device ID "=120, "Layer"=2, "Echo"=0, "Reserved"=0, "Timestamp"=0, "flags"=0, "Reserved 2"=4}, {"X  position"=11.142666, "Y  position"=3.2835486, "Z  position"=0.62424093, "Echo width"=2.2, "Device ID "=120, "Layer"=3, "Echo"=0, "Reserved"=0, "Timestamp"=0, "flags"=4, "Reserved 2"=0}, {"X  position"=10.521912, "Y  position"=2.9806247, "Z  position"=0.29020935, "Echo width"=1.56, "Device ID "=120, "Layer"=0, "Echo"=0, "Reserved"=0, "Timestamp"=0, "flags"=16, "Reserved 2"=4}, {"X  position"=10.514076, "Y  position"=2.9772987, "Z  position"=0.39680278, "Echo width"=1.8, "Device ID "=120, "Layer"=1, "Echo"=0, "Reserved"=0, "Timestamp"=0, "flags"=16, "Reserved 2"=4}, {"X  position"=10.720657, "Y  position"=3.027873, "Z  position"=0.5046632, "Echo width"=1.28, "Device ID "=120, "Layer"=2, "Echo"=0, "Reserved"=0, "Timestamp"=0, "flags"=16, "Reserved 2"=4}, {"X  position"=10.547654, "Y  position"=2.919234, "Z  position"=0.29020935, "Echo width"=1.88, "Device ID "=120, "Layer"=0, "Echo"=0, "Reserved"=0, "Timestamp"=0, "flags"=0, "Reserved 2"=4}, {"X  position"=10.521313, "Y  position"=2.9083233, "Z  position"=0.3969424, "Echo width"=1.9599999, "Device ID "=120, "Layer"=1, "Echo"=0, "Reserved"=0, "Timestamp"=0, "flags"=0, "Reserved 2"=4}, {"X  position"=10.73755, "Y  position"=2.9609597, "Z  position"=0.50459343, "Echo width"=1.5999999, "Device ID "=120, "Layer"=2, "Echo"=0, "Reserved"=0, "Timestamp"=0, "flags"=0, "Reserved 2"=4}, {"X  position"=10.773152, "Y  position"=2.9755251, "Z  position"=0.6146074, "Echo width"=1.48, "Device ID "=120, "Layer"=3, "Echo"=0, "Reserved"=0, "Timestamp"=0, "flags"=4, "Reserved 2"=0}, {"X  position"=10.498703, "Y  position"=2.8276591, "Z  position"=0.29188472, "Echo width"=1.64, "Device ID "=120, "Layer"=0, "Echo"=0, "Reserved"=0, "Timestamp"=0, "flags"=16, "Reserved 2"=4}, {"X  position"=10.509338, "Y  position"=2.8319566, "Z  position"=0.39722165, "Echo width"=1.88, "Device ID "=120, "Layer"=1, "Echo"=0, "Reserved"=0, "Timestamp"=0, "flags"=16, "Reserved 2"=4}, {"X  position"=10.660948, "Y  position"=2.856928, "Z  position"=0.5038255, "Echo width"=1.3199999, "Device ID "=120, "Layer"=2, "Echo"=0, "Reserved"=0, "Timestamp"=0, "flags"=16, "Reserved 2"=4}, {"X  position"=13.918957, "Y  position"=4.156742, "Z  position"=0.68497396, "Echo width"=0.71999997, "Device ID "=120, "Layer"=3, "Echo"=0, "Reserved"=0, "Timestamp"=0, "flags"=16, "Reserved 2"=6}, {"X  position"=10.485903, "Y  position"=2.7518203, "Z  position"=0.2927224, "Echo width"=1.88, "Device ID "=120, "Layer"=0, "Echo"=0, "Reserved"=0, "Timestamp"=0, "flags"=0, "Reserved 2"=4}, {"X  position"=10.524481, "Y  position"=2.767017, "Z  position"=0.39729148, "Echo width"=2.0, "Device ID "=120, "Layer"=1, "Echo"=0, "Reserved"=0, "Timestamp"=0, "flags"=0, "Reserved 2"=4}, {"X  position"=10.592407, "Y  position"=2.7580862, "Z  position"=0.5031274, "Echo width"=1.52, "Device ID "=120, "Layer"=2, "Echo"=0, "Reserved"=0, "Timestamp"=0, "flags"=0, "Reserved 2"=4}, {"X  position"=10.628296, "Y  position"=2.7720428, "Z  position"=0.61020947, "Echo width"=1.4, "Device ID "=120, "Layer"=3, "Echo"=0, "Reserved"=0, "Timestamp"=0, "flags"=4096, "Reserved 2"=4}, {"X  position"=14.001424, "Y  position"=4.083781, "Z  position"=0.68602103, "Echo width"=1.64, "Device ID "=120, "Layer"=3, "Echo"=1, "Reserved"=0, "Timestamp"=0, "flags"=0, "Reserved 2"=6}, {"X  position"=10.472316, "Y  position"=2.6764214, "Z  position"=0.29356012, "Echo width"=1.56, "Device ID "=120, "Layer"=0, "Echo"=0, "Reserved"=0, "Timestamp"=0, "flags"=16, "Reserved 2"=4}, {"X  position"=10.520353, "Y  position"=2.6948614, "Z  position"=0.3975009, "Echo width"=1.88, "Device ID "=120, "Layer"=1, "Echo"=0, "Reserved"=0, "Timestamp"=0, "flags"=16, "Reserved 2"=4}, {"X  position"=10.597503, "Y  position"=2.6890035, "Z  position"=0.50298774, "Echo width"=1.16, "Device ID "=120, "Layer"=2, "Echo"=0, "Reserved"=0, "Timestamp"=0, "flags"=16, "Reserved 2"=4}, {"X  position"=10.586769, "Y  position"=2.684937, "Z  position"=0.60874355, "Echo width"=0.68, "Device ID "=120, "Layer"=3, "Echo"=0, "Reserved"=0, "Timestamp"=0, "flags"=4112, "Reserved 2"=4}, {"X  position"=14.214298, "Y  position"=4.0592847, "Z  position"=0.6900001, "Echo width"=1.36, "Device ID "=120, "Layer"=3, "Echo"=1, "Reserved"=0, "Timestamp"=0, "flags"=16, "Reserved 2"=6}, {"X  position"=10.495407, "Y  position"=2.6154754, "Z  position"=0.29356012, "Echo width"=1.8399999, "Device ID "=120, "Layer"=0, "Echo"=0, "Reserved"=0, "Timestamp"=0, "flags"=0, "Reserved 2"=4}, {"X  position"=10.571703, "Y  position"=2.6440012, "Z  position"=0.39729148, "Echo width"=2.0, "Device ID "=120, "Layer"=1, "Echo"=0, "Reserved"=0, "Timestamp"=0, "flags"=0, "Reserved 2"=4}, {"X  position"=10.658225, "Y  position"=2.6408088, "Z  position"=0.503267, "Echo width"=1.76, "Device ID "=120, "Layer"=2, "Echo"=0, "Reserved"=0, "Timestamp"=0, "flags"=0, "Reserved 2"=4}, {"X  position"=10.638069, "Y  position"=2.633373, "Z  position"=0.6093718, "Echo width"=1.36, "Device ID "=120, "Layer"=3, "Echo"=0, "Reserved"=0, "Timestamp"=0, "flags"=4096, "Reserved 2"=4}, {"X  position"=14.390013, "Y  position"=4.017538, "Z  position"=0.69314146, "Echo width"=1.8399999, "Device ID "=120, "Layer"=3, "Echo"=1, "Reserved"=0, "Timestamp"=0, "flags"=0, "Reserved 2"=6}, {"X  position"=10.555544, "Y  position"=2.5680077, "Z  position"=0.2927224, "Echo width"=1.7199999, "Device ID "=120, "Layer"=0, "Echo"=0, "Reserved"=0, "Timestamp"=0, "flags"=16, "Reserved 2"=4}, {"X  position"=10.556919, "Y  position"=2.5685086, "Z  position"=0.39757073, "Echo width"=1.92, "Device ID "=120, "Layer"=1, "Echo"=0, "Reserved"=0, "Timestamp"=0, "flags"=16, "Reserved 2"=4}, {"X  position"=10.671586, "Y  position"=2.5748627, "Z  position"=0.5031972, "Echo width"=1.56, "Device ID "=120, "Layer"=2, "Echo"=0, "Reserved"=0, "Timestamp"=0, "flags"=16, "Reserved 2"=4}, {"X  position"=10.651369, "Y  position"=2.5676038, "Z  position"=0.6091624, "Echo width"=1.0799999, "Device ID "=120, "Layer"=3, "Echo"=0, "Reserved"=0, "Timestamp"=0, "flags"=16, "Reserved 2"=4}, {"X  position"=10.577684, "Y  position"=2.5063396, "Z  position"=0.2927224, "Echo width"=2.24, "Device ID "=120, "Layer"=0, "Echo"=0, "Reserved"=0, "Timestamp"=0, "flags"=0, "Reserved 2"=4}, {"X  position"=10.569639, "Y  position"=2.5034907, "Z  position"=0.39764053, "Echo width"=2.08, "Device ID "=120, "Layer"=1, "Echo"=0, "Reserved"=0, "Timestamp"=0, "flags"=0, "Reserved 2"=4}, {"X  position"=10.674901, "Y  position"=2.5055876, "Z  position"=0.50305754, "Echo width"=1.8399999, "Device ID "=120, "Layer"=2, "Echo"=0, "Reserved"=0, "Timestamp"=0, "flags"=0, "Reserved 2"=4}, {"X  position"=10.69238, "Y  position"=2.5116916, "Z  position"=0.60958123, "Echo width"=1.48, "Device ID "=120, "Layer"=3, "Echo"=0, "Reserved"=0, "Timestamp"=0, "flags"=0, "Reserved 2"=4}, {"X  position"=10.561474, "Y  position"=2.4314606, "Z  position"=0.29356012, "Echo width"=1.9599999, "Device ID "=120, "Layer"=0, "Echo"=0, "Reserved"=0, "Timestamp"=0, "flags"=16, "Reserved 2"=4}, {"X  position"=10.600671, "Y  position"=2.444957, "Z  position"=0.39757073, "Echo width"=1.9599999, "Device ID "=120, "Layer"=1, "Echo"=0, "Reserved"=0, "Timestamp"=0, "flags"=16, "Reserved 2"=4}, {"X  position"=10.639679, "Y  position"=2.4235945, "Z  position"=0.5026387, "Echo width"=1.56, "Device ID "=120, "Layer"=2, "Echo"=0, "Reserved"=0, "Timestamp"=0, "flags"=16, "Reserved 2"=4}, {"X  position"=10.657221, "Y  position"=2.4295492, "Z  position"=0.60832465, "Echo width"=1.0799999, "Device ID "=120, "Layer"=3, "Echo"=0, "Reserved"=0, "Timestamp"=0, "flags"=16, "Reserved 2"=4}, {"X  position"=10.6108675, "Y  position"=2.379263, "Z  position"=0.29293185, "Echo width"=2.04, "Device ID "=120, "Layer"=0, "Echo"=0, "Reserved"=0, "Timestamp"=0, "flags"=0, "Reserved 2"=4}, {"X  position"=10.574322, "Y  position"=2.3670352, "Z  position"=0.39791977, "Echo width"=2.12, "Device ID "=120, "Layer"=1, "Echo"=0, "Reserved"=0, "Timestamp"=0, "flags"=0, "Reserved 2"=4}, {"X  position"=10.632067, "Y  position"=2.3518028, "Z  position"=0.50242925, "Echo width"=1.8, "Device ID "=120, "Layer"=2, "Echo"=0, "Reserved"=0, "Timestamp"=0, "flags"=0, "Reserved 2"=4}, {"X  position"=10.7066345, "Y  position"=2.376392, "Z  position"=0.60895294, "Echo width"=1.52, "Device ID "=120, "Layer"=3, "Echo"=0, "Reserved"=0, "Timestamp"=0, "flags"=4096, "Reserved 2"=4}, {"X  position"=14.210257, "Y  position"=3.531713, "Z  position"=0.6862305, "Echo width"=1.1999999, "Device ID "=120, "Layer"=3, "Echo"=1, "Reserved"=0, "Timestamp"=0, "flags"=4, "Reserved 2"=0}, {"X  position"=10.659884, "Y  position"=2.3263874, "Z  position"=0.29230356, "Echo width"=1.8399999, "Device ID "=120, "Layer"=0, "Echo"=0, "Reserved"=0, "Timestamp"=0, "flags"=16, "Reserved 2"=4}, {"X  position"=10.6327505, "Y  position"=2.3175712, "Z  position"=0.39764053, "Echo width"=2.0, "Device ID "=120, "Layer"=1, "Echo"=0, "Reserved"=0, "Timestamp"=0, "flags"=16, "Reserved 2"=4}, {"X  position"=10.6904125, "Y  position"=2.3016694, "Z  position"=0.5027085, "Echo width"=1.5999999, "Device ID "=120, "Layer"=2, "Echo"=0, "Reserved"=0, "Timestamp"=0, "flags"=16, "Reserved 2"=4}, {"X  position"=10.698532, "Y  position"=2.3042686, "Z  position"=0.60832465, "Echo width"=1.0, "Device ID "=120, "Layer"=3, "Echo"=0, "Reserved"=0, "Timestamp"=0, "flags"=16, "Reserved 2"=4}, {"X  position"=10.641773, "Y  position"=2.2517924, "Z  position"=0.29314128, "Echo width"=2.08, "Device ID "=120, "Layer"=0, "Echo"=0, "Reserved"=0, "Timestamp"=0, "flags"=0, "Reserved 2"=4}, {"X  position"=10.652702, "Y  position"=2.2552385, "Z  position"=0.39764053, "Echo width"=2.08, "Device ID "=120, "Layer"=1, "Echo"=0, "Reserved"=0, "Timestamp"=0, "flags"=0, "Reserved 2"=4}, {"X  position"=10.681576, "Y  position"=2.2299385, "Z  position"=0.50249904, "Echo width"=1.8399999, "Device ID "=120, "Layer"=2, "Echo"=0, "Reserved"=0, "Timestamp"=0, "flags"=0, "Reserved 2"=4}, {"X  position"=10.737463, "Y  position"=2.2472923, "Z  position"=0.60874355, "Echo width"=1.48, "Device ID "=120, "Layer"=3, "Echo"=0, "Reserved"=0, "Timestamp"=0, "flags"=4096, "Reserved 2"=4}, {"X  position"=14.318003, "Y  position"=3.3590794, "Z  position"=0.6872776, "Echo width"=1.36, "Device ID "=120, "Layer"=3, "Echo"=1, "Reserved"=0, "Timestamp"=0, "flags"=4, "Reserved 2"=0}, {"X  position"=10.699394, "Y  position"=2.201076, "Z  position"=0.29230356, "Echo width"=1.8399999, "Device ID "=120, "Layer"=0, "Echo"=0, "Reserved"=0, "Timestamp"=0, "flags"=16, "Reserved 2"=4}, {"X  position"=10.6721115, "Y  position"=2.1927345, "Z  position"=0.39764053, "Echo width"=1.76, "Device ID "=120, "Layer"=1, "Echo"=0, "Reserved"=0, "Timestamp"=0, "flags"=16, "Reserved 2"=4}, {"X  position"=10.719912, "Y  position"=2.1729472, "Z  position"=0.5026387, "Echo width"=1.52, "Device ID "=120, "Layer"=2, "Echo"=0, "Reserved"=0, "Timestamp"=0, "flags"=16, "Reserved 2"=4}, {"X  position"=10.823813, "Y  position"=2.204218, "Z  position"=0.61020947, "Echo width"=1.1999999, "Device ID "=120, "Layer"=3, "Echo"=0, "Reserved"=0, "Timestamp"=0, "flags"=16, "Reserved 2"=4}, {"X  position"=10.689571, "Y  position"=2.129648, "Z  position"=0.29293185, "Echo width"=2.0, "Device ID "=120, "Layer"=0, "Echo"=0, "Reserved"=0, "Timestamp"=0, "flags"=0, "Reserved 2"=4}, {"X  position"=10.690973, "Y  position"=2.1300633, "Z  position"=0.39764053, "Echo width"=1.8, "Device ID "=120, "Layer"=1, "Echo"=0, "Reserved"=0, "Timestamp"=0, "flags"=0, "Reserved 2"=4}, {"X  position"=10.748199, "Y  position"=2.1126575, "Z  position"=0.5027085, "Echo width"=1.8, "Device ID "=120, "Layer"=2, "Echo"=0, "Reserved"=0, "Timestamp"=0, "flags"=0, "Reserved 2"=4}, {"X  position"=10.833172, "Y  position"=2.137425, "Z  position"=0.6100001, "Echo width"=1.7199999, "Device ID "=120, "Layer"=3, "Echo"=0, "Reserved"=0, "Timestamp"=0, "flags"=0, "Reserved 2"=4}, {"X  position"=10.717491, "Y  position"=2.0695825, "Z  position"=0.2927224, "Echo width"=1.5999999, "Device ID "=120, "Layer"=0, "Echo"=0, "Reserved"=0, "Timestamp"=0, "flags"=16, "Reserved 2"=4}, {"X  position"=10.853472, "Y  position"=2.1085744, "Z  position"=0.39659336, "Echo width"=1.64, "Device ID "=120, "Layer"=1, "Echo"=0, "Reserved"=0, "Timestamp"=0, "flags"=16, "Reserved 2"=4}, {"X  position"=10.727862, "Y  position"=2.038468, "Z  position"=0.50242925, "Echo width"=1.28, "Device ID "=120, "Layer"=2, "Echo"=0, "Reserved"=0, "Timestamp"=0, "flags"=16, "Reserved 2"=4}, {"X  position"=10.861167, "Y  position"=2.0760639, "Z  position"=0.61020947, "Echo width"=1.24, "Device ID "=120, "Layer"=3, "Echo"=0, "Reserved"=0, "Timestamp"=0, "flags"=16, "Reserved 2"=4}, {"X  position"=10.821985, "Y  position"=2.0305662, "Z  position"=0.2908376, "Echo width"=1.7199999, "Device ID "=120, "Layer"=0, "Echo"=0, "Reserved"=0, "Timestamp"=0, "flags"=0, "Reserved 2"=4}, {"X  position"=10.881229, "Y  position"=2.0469959, "Z  position"=0.39652354, "Echo width"=1.68, "Device ID "=120, "Layer"=1, "Echo"=0, "Reserved"=0, "Timestamp"=0, "flags"=0, "Reserved 2"=4}, {"X  position"=10.841852, "Y  position"=2.0016186, "Z  position"=0.5031274, "Echo width"=1.56, "Device ID "=120, "Layer"=2, "Echo"=0, "Reserved"=0, "Timestamp"=0, "flags"=0, "Reserved 2"=4}, {"X  position"=11.014045, "Y  position"=2.0485637, "Z  position"=0.6131414, "Echo width"=1.52, "Device ID "=120, "Layer"=3, "Echo"=0, "Reserved"=0, "Timestamp"=0, "flags"=4096, "Reserved 2"=4}, {"X  position"=14.062104, "Y  position"=2.8795602, "Z  position"=0.6793195, "Echo width"=1.12, "Device ID "=120, "Layer"=3, "Echo"=1, "Reserved"=0, "Timestamp"=0, "flags"=4, "Reserved 2"=0}, {"X  position"=10.878055, "Y  position"=1.9769437, "Z  position"=0.2899999, "Echo width"=1.1999999, "Device ID "=120, "Layer"=0, "Echo"=0, "Reserved"=0, "Timestamp"=0, "flags"=16, "Reserved 2"=4}, {"X  position"=10.90847, "Y  position"=1.9850936, "Z  position"=0.39645374, "Echo width"=1.3199999, "Device ID "=120, "Layer"=1, "Echo"=0, "Reserved"=0, "Timestamp"=0, "flags"=16, "Reserved 2"=4}, {"X  position"=10.917061, "Y  position"=1.9527493, "Z  position"=0.50354624, "Echo width"=1.1999999, "Device ID "=120, "Layer"=2, "Echo"=0, "Reserved"=0, "Timestamp"=0, "flags"=16, "Reserved 2"=4}, {"X  position"=11.089645, "Y  position"=1.998187, "Z  position"=0.614398, "Echo width"=1.1999999, "Device ID "=120, "Layer"=3, "Echo"=0, "Reserved"=0, "Timestamp"=0, "flags"=16, "Reserved 2"=4}, {"X  position"=11.040216, "Y  position"=1.9500325, "Z  position"=0.28685856, "Echo width"=1.5999999, "Device ID "=120, "Layer"=0, "Echo"=0, "Reserved"=0, "Timestamp"=0, "flags"=0, "Reserved 2"=4}, {"X  position"=11.022324, "Y  position"=1.9454052, "Z  position"=0.3957556, "Echo width"=1.48, "Device ID "=120, "Layer"=1, "Echo"=0, "Reserved"=0, "Timestamp"=0, "flags"=0, "Reserved 2"=4}, {"X  position"=11.050125, "Y  position"=1.9174875, "Z  position"=0.504384, "Echo width"=1.36, "Device ID "=120, "Layer"=2, "Echo"=0, "Reserved"=0, "Timestamp"=0, "flags"=0, "Reserved 2"=4}, {"X  position"=11.194006, "Y  position"=1.9540285, "Z  position"=0.6162828, "Echo width"=1.4399999, "Device ID "=120, "Layer"=3, "Echo"=0, "Reserved"=0, "Timestamp"=0, "flags"=0, "Reserved 2"=4}, {"X  position"=11.095749, "Y  position"=1.8938329, "Z  position"=0.28602085, "Echo width"=1.0799999, "Device ID "=120, "Layer"=0, "Echo"=0, "Reserved"=0, "Timestamp"=0, "flags"=16, "Reserved 2"=4}, {"X  position"=11.136042, "Y  position"=1.9038789, "Z  position"=0.39505747, "Echo width"=1.04, "Device ID "=120, "Layer"=1, "Echo"=0, "Reserved"=0, "Timestamp"=0, "flags"=16, "Reserved 2"=4}, {"X  position"=11.183128, "Y  position"=1.8800497, "Z  position"=0.5052217, "Echo width"=1.16, "Device ID "=120, "Layer"=2, "Echo"=0, "Reserved"=0, "Timestamp"=0, "flags"=16, "Reserved 2"=4}, {"X  position"=11.201054, "Y  position"=1.8844358, "Z  position"=0.61607337, "Echo width"=1.16, "Device ID "=120, "Layer"=3, "Echo"=0, "Reserved"=0, "Timestamp"=0, "flags"=16, "Reserved 2"=4}, {"X  position"=11.432798, "Y  position"=1.9044963, "Z  position"=0.27910984, "Echo width"=1.76, "Device ID "=120, "Layer"=0, "Echo"=0, "Reserved"=0, "Timestamp"=0, "flags"=0, "Reserved 2"=4}, {"X  position"=11.482962, "Y  position"=1.9165398, "Z  position"=0.39268383, "Echo width"=1.8399999, "Device ID "=120, "Layer"=1, "Echo"=0, "Reserved"=0, "Timestamp"=0, "flags"=0, "Reserved 2"=4}, {"X  position"=11.617785, "Y  position"=1.9114847, "Z  position"=0.5082237, "Echo width"=1.7199999, "Device ID "=120, "Layer"=2, "Echo"=0, "Reserved"=0, "Timestamp"=0, "flags"=0, "Reserved 2"=4}, {"X  position"=11.557813, "Y  position"=1.8973631, "Z  position"=0.6234032, "Echo width"=1.68, "Device ID "=120, "Layer"=3, "Echo"=0, "Reserved"=0, "Timestamp"=0, "flags"=0, "Reserved 2"=4}, {"X  position"=11.809553, "Y  position"=1.9184116, "Z  position"=0.27136117, "Echo width"=1.28, "Device ID "=120, "Layer"=0, "Echo"=0, "Reserved"=0, "Timestamp"=0, "flags"=16, "Reserved 2"=4}, {"X  position"=11.879377, "Y  position"=1.9345318, "Z  position"=0.38996115, "Echo width"=1.4399999, "Device ID "=120, "Layer"=1, "Echo"=0, "Reserved"=0, "Timestamp"=0, "flags"=16, "Reserved 2"=4}, {"X  position"=11.926751, "Y  position"=1.9067793, "Z  position"=0.51031804, "Echo width"=1.36, "Device ID "=120, "Layer"=2, "Echo"=0, "Reserved"=0, "Timestamp"=0, "flags"=16, "Reserved 2"=4}, {"X  position"=14.401936, "Y  position"=2.4668562, "Z  position"=0.6841362, "Echo width"=1.3199999, "Device ID "=120, "Layer"=3, "Echo"=0, "Reserved"=0, "Timestamp"=0, "flags"=16, "Reserved 2"=7}, {"X  position"=12.128564, "Y  position"=1.9129066, "Z  position"=0.26486897, "Echo width"=1.4, "Device ID "=120, "Layer"=0, "Echo"=0, "Reserved"=0, "Timestamp"=0, "flags"=4097, "Reserved 2"=0}, {"X  position"=17.008972, "Y  position"=2.9948673, "Z  position"=0.1601569, "Echo width"=1.36, "Device ID "=120, "Layer"=0, "Echo"=1, "Reserved"=0, "Timestamp"=0, "flags"=1, "Reserved 2"=0}, {"X  position"=12.247399, "Y  position"=1.9392518, "Z  position"=0.3874479, "Echo width"=1.36, "Device ID "=120, "Layer"=1, "Echo"=0, "Reserved"=0, "Timestamp"=0, "flags"=4, "Reserved 2"=0}, {"X  position"=12.431673, "Y  position"=1.9392565, "Z  position"=0.5138087, "Echo width"=1.28, "Device ID "=120, "Layer"=2, "Echo"=0, "Reserved"=0, "Timestamp"=0, "flags"=4100, "Reserved 2"=0}, {"X  position"=14.493582, "Y  position"=2.3869407, "Z  position"=0.5285392, "Echo width"=1.1999999, "Device ID "=120, "Layer"=2, "Echo"=1, "Reserved"=0, "Timestamp"=0, "flags"=4, "Reserved 2"=0}, {"X  position"=14.374196, "Y  position"=2.3610196, "Z  position"=0.68308914, "Echo width"=1.8399999, "Device ID "=120, "Layer"=3, "Echo"=0, "Reserved"=0, "Timestamp"=0, "flags"=0, "Reserved 2"=7}, {"X  position"=12.7041445, "Y  position"=1.9564012, "Z  position"=0.38430634, "Echo width"=0.79999995, "Device ID "=120, "Layer"=1, "Echo"=0, "Reserved"=0, "Timestamp"=0, "flags"=4113, "Reserved 2"=0}, {"X  position"=17.115482, "Y  position"=2.8940604, "Z  position"=0.35282084, "Echo width"=1.7199999, "Device ID "=120, "Layer"=1, "Echo"=1, "Reserved"=0, "Timestamp"=0, "flags"=20, "Reserved 2"=0}, {"X  position"=14.443327, "Y  position"=2.2762153, "Z  position"=0.6841362, "Echo width"=1.3199999, "Device ID "=120, "Layer"=3, "Echo"=0, "Reserved"=0, "Timestamp"=0, "flags"=16, "Reserved 2"=7}, {"X  position"=13.012981, "Y  position"=1.9354382, "Z  position"=0.24664909, "Echo width"=1.24, "Device ID "=120, "Layer"=0, "Echo"=0, "Reserved"=0, "Timestamp"=0, "flags"=1, "Reserved 2"=0}, {"X  position"=13.142223, "Y  position"=1.9617326, "Z  position"=0.38130438, "Echo width"=1.28, "Device ID "=120, "Layer"=1, "Echo"=0, "Reserved"=0, "Timestamp"=0, "flags"=4, "Reserved 2"=0}, {"X  position"=13.680304, "Y  position"=2.0249882, "Z  position"=0.52246547, "Echo width"=1.5999999, "Device ID "=120, "Layer"=2, "Echo"=0, "Reserved"=0, "Timestamp"=0, "flags"=0, "Reserved 2"=7}, {"X  position"=14.080351, "Y  position"=2.1045628, "Z  position"=0.6759687, "Echo width"=1.5999999, "Device ID "=120, "Layer"=3, "Echo"=0, "Reserved"=0, "Timestamp"=0, "flags"=0, "Reserved 2"=7}, {"X  position"=13.610514, "Y  position"=1.9652848, "Z  position"=0.378093, "Echo width"=0.59999996, "Device ID "=120, "Layer"=1, "Echo"=0, "Reserved"=0, "Timestamp"=0, "flags"=16, "Reserved 2"=7}, {"X  position"=13.93337, "Y  position"=1.9808372, "Z  position"=0.52414095, "Echo width"=0.91999996, "Device ID "=120, "Layer"=2, "Echo"=0, "Reserved"=0, "Timestamp"=0, "flags"=16, "Reserved 2"=7}, {"X  position"=14.07867, "Y  position"=2.0084233, "Z  position"=0.67554986, "Echo width"=1.12, "Device ID "=120, "Layer"=3, "Echo"=0, "Reserved"=0, "Timestamp"=0, "flags"=16, "Reserved 2"=7}, {"X  position"=14.1856365, "Y  position"=1.9804657, "Z  position"=0.22235589, "Echo width"=1.5999999, "Device ID "=120, "Layer"=0, "Echo"=0, "Reserved"=0, "Timestamp"=0, "flags"=4, "Reserved 2"=0}, {"X  position"=14.2172165, "Y  position"=1.9863187, "Z  position"=0.37390426, "Echo width"=1.68, "Device ID "=120, "Layer"=1, "Echo"=0, "Reserved"=0, "Timestamp"=0, "flags"=4, "Reserved 2"=0}, {"X  position"=14.3930645, "Y  position"=1.9697869, "Z  position"=0.52728254, "Echo width"=1.76, "Device ID "=120, "Layer"=2, "Echo"=0, "Reserved"=0, "Timestamp"=0, "flags"=4, "Reserved 2"=0}, {"X  position"=14.154822, "Y  position"=1.9267058, "Z  position"=0.6768064, "Echo width"=1.5999999, "Device ID "=120, "Layer"=3, "Echo"=0, "Reserved"=0, "Timestamp"=0, "flags"=0, "Reserved 2"=7}, {"X  position"=17.156288, "Y  position"=2.407972, "Z  position"=0.15952864, "Echo width"=1.8, "Device ID "=120, "Layer"=0, "Echo"=0, "Reserved"=0, "Timestamp"=0, "flags"=16, "Reserved 2"=8}, {"X  position"=17.188494, "Y  position"=2.413651, "Z  position"=0.35296047, "Echo width"=1.76, "Device ID "=120, "Layer"=1, "Echo"=0, "Reserved"=0, "Timestamp"=0, "flags"=16, "Reserved 2"=8}, {"X  position"=17.731083, "Y  position"=2.4453473, "Z  position"=0.5508094, "Echo width"=1.4399999, "Device ID "=120, "Layer"=2, "Echo"=0, "Reserved"=0, "Timestamp"=0, "flags"=4096, "Reserved 2"=8}, {"X  position"=23.240206, "Y  position"=3.3919878, "Z  position"=0.58983463, "Echo width"=1.0799999, "Device ID "=120, "Layer"=2, "Echo"=1, "Reserved"=0, "Timestamp"=0, "flags"=2, "Reserved 2"=9}, {"X  position"=14.476686, "Y  position"=1.8861396, "Z  position"=0.6832985, "Echo width"=1.4399999, "Device ID "=120, "Layer"=3, "Echo"=0, "Reserved"=0, "Timestamp"=0, "flags"=16, "Reserved 2"=7}, {"X  position"=10.639141, "Y  position"=1.1946825, "Z  position"=0.29837686, "Echo width"=1.3199999, "Device ID "=120, "Layer"=0, "Echo"=0, "Reserved"=0, "Timestamp"=0, "flags"=4096, "Reserved 2"=10}, {"X  position"=17.216225, "Y  position"=2.2953086, "Z  position"=0.15869093, "Echo width"=1.5999999, "Device ID "=120, "Layer"=0, "Echo"=1, "Reserved"=0, "Timestamp"=0, "flags"=0, "Reserved 2"=8}, {"X  position"=10.679984, "Y  position"=1.2015172, "Z  position"=0.39917642, "Echo width"=1.28, "Device ID "=120, "Layer"=1, "Echo"=0, "Reserved"=0, "Timestamp"=0, "flags"=4096, "Reserved 2"=10}, {"X  position"=17.248486, "Y  position"=2.3007073, "Z  position"=0.35268122, "Echo width"=1.64, "Device ID "=120, "Layer"=1, "Echo"=1, "Reserved"=0, "Timestamp"=0, "flags"=0, "Reserved 2"=8}, {"X  position"=10.62594, "Y  position"=1.1605331, "Z  position"=0.5004047, "Echo width"=1.28, "Device ID "=120, "Layer"=2, "Echo"=0, "Reserved"=0, "Timestamp"=0, "flags"=4096, "Reserved 2"=10}, {"X  position"=17.465656, "Y  position"=2.274452, "Z  position"=0.5487848, "Echo width"=1.4, "Device ID "=120, "Layer"=2, "Echo"=1, "Reserved"=0, "Timestamp"=0, "flags"=0, "Reserved 2"=8}, {"X  position"=10.762699, "Y  position"=1.1828058, "Z  position"=0.60413617, "Echo width"=1.24, "Device ID "=120, "Layer"=3, "Echo"=0, "Reserved"=0, "Timestamp"=0, "flags"=4096, "Reserved 2"=10}, {"X  position"=14.157223, "Y  position"=1.7356391, "Z  position"=0.6761781, "Echo width"=1.9599999, "Device ID "=120, "Layer"=3, "Echo"=1, "Reserved"=0, "Timestamp"=0, "flags"=0, "Reserved 2"=7}, {"X  position"=10.402428, "Y  position"=1.0932372, "Z  position"=0.30361247, "Echo width"=1.48, "Device ID "=120, "Layer"=0, "Echo"=0, "Reserved"=0, "Timestamp"=0, "flags"=16, "Reserved 2"=10}, {"X  position"=10.4136505, "Y  position"=1.0950146, "Z  position"=0.40113115, "Echo width"=1.56, "Device ID "=120, "Layer"=1, "Echo"=0, "Reserved"=0, "Timestamp"=0, "flags"=16, "Reserved 2"=10}, {"X  position"=10.477662, "Y  position"=1.073965, "Z  position"=0.4992877, "Echo width"=1.56, "Device ID "=120, "Layer"=2, "Echo"=0, "Reserved"=0, "Timestamp"=0, "flags"=16, "Reserved 2"=10}, {"X  position"=10.664049, "Y  position"=1.1026527, "Z  position"=0.6018325, "Echo width"=1.16, "Device ID "=120, "Layer"=3, "Echo"=0, "Reserved"=0, "Timestamp"=0, "flags"=16, "Reserved 2"=10}, {"X  position"=10.342489, "Y  position"=1.0226169, "Z  position"=0.30507845, "Echo width"=1.8, "Device ID "=120, "Layer"=0, "Echo"=0, "Reserved"=0, "Timestamp"=0, "flags"=0, "Reserved 2"=10}, {"X  position"=10.403162, "Y  position"=1.0316845, "Z  position"=0.4012708, "Echo width"=1.76, "Device ID "=120, "Layer"=1, "Echo"=0, "Reserved"=0, "Timestamp"=0, "flags"=0, "Reserved 2"=10}, {"X  position"=10.496664, "Y  position"=1.0144681, "Z  position"=0.4993575, "Echo width"=1.92, "Device ID "=120, "Layer"=2, "Echo"=0, "Reserved"=0, "Timestamp"=0, "flags"=0, "Reserved 2"=10}, {"X  position"=10.544772, "Y  position"=1.0214434, "Z  position"=0.59911, "Echo width"=1.68, "Device ID "=120, "Layer"=3, "Echo"=0, "Reserved"=0, "Timestamp"=0, "flags"=0, "Reserved 2"=10}, {"X  position"=10.262047, "Y  position"=0.9503438, "Z  position"=0.30696326, "Echo width"=1.64, "Device ID "=120, "Layer"=0, "Echo"=0, "Reserved"=0, "Timestamp"=0, "flags"=16, "Reserved 2"=10}, {"X  position"=10.233658, "Y  position"=0.946354, "Z  position"=0.40252742, "Echo width"=1.56, "Device ID "=120, "Layer"=1, "Echo"=0, "Reserved"=0, "Timestamp"=0, "flags"=16, "Reserved 2"=10}, {"X  position"=10.445801, "Y  position"=0.945282, "Z  position"=0.49893862, "Echo width"=1.68, "Device ID "=120, "Layer"=2, "Echo"=0, "Reserved"=0, "Timestamp"=0, "flags"=16, "Reserved 2"=10}, {"X  position"=10.454353, "Y  position"=0.94644594, "Z  position"=0.59701574, "Echo width"=1.36, "Device ID "=120, "Layer"=3, "Echo"=0, "Reserved"=0, "Timestamp"=0, "flags"=16, "Reserved 2"=10}, {"X  position"=10.270082, "Y  position"=0.89129835, "Z  position"=0.30696326, "Echo width"=1.8399999, "Device ID "=120, "Layer"=0, "Echo"=0, "Reserved"=0, "Timestamp"=0, "flags"=0, "Reserved 2"=10}, {"X  position"=10.320974, "Y  position"=0.8979983, "Z  position"=0.40196893, "Echo width"=1.9599999, "Device ID "=120, "Layer"=1, "Echo"=0, "Reserved"=0, "Timestamp"=0, "flags"=0, "Reserved 2"=10}, {"X  position"=10.3446665, "Y  position"=0.87075156, "Z  position"=0.49817067, "Echo width"=1.5999999, "Device ID "=120, "Layer"=2, "Echo"=0, "Reserved"=0, "Timestamp"=0, "flags"=0, "Reserved 2"=10}, {"X  position"=10.3532505, "Y  position"=0.8718435, "Z  position"=0.59471214, "Echo width"=1.5999999, "Device ID "=120, "Layer"=3, "Echo"=0, "Reserved"=0, "Timestamp"=0, "flags"=4096, "Reserved 2"=10}, {"X  position"=14.300563, "Y  position"=1.3740052, "Z  position"=0.6780629, "Echo width"=1.3199999, "Device ID "=120, "Layer"=3, "Echo"=1, "Reserved"=0, "Timestamp"=0, "flags"=4, "Reserved 2"=0}, {"X  position"=10.277603, "Y  position"=0.83218503, "Z  position"=0.30696326, "Echo width"=1.8, "Device ID "=120, "Layer"=0, "Echo"=0, "Reserved"=0, "Timestamp"=0, "flags"=16, "Reserved 2"=10}, {"X  position"=10.268999, "Y  position"=0.83112866, "Z  position"=0.4023878, "Echo width"=1.8, "Device ID "=120, "Layer"=1, "Echo"=0, "Reserved"=0, "Timestamp"=0, "flags"=16, "Reserved 2"=10}, {"X  position"=10.322214, "Y  position"=0.8074623, "Z  position"=0.49796125, "Echo width"=1.1999999, "Device ID "=120, "Layer"=2, "Echo"=0, "Reserved"=0, "Timestamp"=0, "flags"=16, "Reserved 2"=10}, {"X  position"=10.350669, "Y  position"=0.8108301, "Z  position"=0.5945027, "Echo width"=1.28, "Device ID "=120, "Layer"=3, "Echo"=0, "Reserved"=0, "Timestamp"=0, "flags"=16, "Reserved 2"=10}, {"X  position"=10.23494, "Y  position"=0.7673494, "Z  position"=0.3080104, "Echo width"=2.04, "Device ID "=120, "Layer"=0, "Echo"=0, "Reserved"=0, "Timestamp"=0, "flags"=0, "Reserved 2"=10}, {"X  position"=10.285931, "Y  position"=0.77315915, "Z  position"=0.40231797, "Echo width"=2.0, "Device ID "=120, "Layer"=1, "Echo"=0, "Reserved"=0, "Timestamp"=0, "flags"=0, "Reserved 2"=10}, {"X  position"=10.319059, "Y  position"=0.7468085, "Z  position"=0.49789143, "Echo width"=1.5999999, "Device ID "=120, "Layer"=2, "Echo"=0, "Reserved"=0, "Timestamp"=0, "flags"=0, "Reserved 2"=10}, {"X  position"=10.337606, "Y  position"=0.7488398, "Z  position"=0.59408385, "Echo width"=1.68, "Device ID "=120, "Layer"=3, "Echo"=0, "Reserved"=0, "Timestamp"=0, "flags"=0, "Reserved 2"=10}, {"X  position"=10.271208, "Y  position"=0.7116827, "Z  position"=0.3073821, "Echo width"=1.8399999, "Device ID "=120, "Layer"=0, "Echo"=0, "Reserved"=0, "Timestamp"=0, "flags"=16, "Reserved 2"=10}, {"X  position"=10.222803, "Y  position"=0.7065951, "Z  position"=0.40280667, "Echo width"=1.88, "Device ID "=120, "Layer"=1, "Echo"=0, "Reserved"=0, "Timestamp"=0, "flags"=16, "Reserved 2"=10}, {"X  position"=10.2556715, "Y  position"=0.6802604, "Z  position"=0.49740273, "Echo width"=1.28, "Device ID "=120, "Layer"=2, "Echo"=0, "Reserved"=0, "Timestamp"=0, "flags"=16, "Reserved 2"=10}, {"X  position"=10.284197, "Y  position"=0.6831327, "Z  position"=0.5928273, "Echo width"=1.4399999, "Device ID "=120, "Layer"=3, "Echo"=0, "Reserved"=0, "Timestamp"=0, "flags"=16, "Reserved 2"=10}, {"X  position"=10.247305, "Y  position"=0.64969164, "Z  position"=0.3080104, "Echo width"=2.04, "Device ID "=120, "Layer"=0, "Echo"=0, "Reserved"=0, "Timestamp"=0, "flags"=0, "Reserved 2"=10}, {"X  position"=10.29839, "Y  position"=0.6546105, "Z  position"=0.40231797, "Echo width"=2.0, "Device ID "=120, "Layer"=1, "Echo"=0, "Reserved"=0, "Timestamp"=0, "flags"=0, "Reserved 2"=10}, {"X  position"=10.331055, "Y  position"=0.6276858, "Z  position"=0.49789143, "Echo width"=1.64, "Device ID "=120, "Layer"=2, "Echo"=0, "Reserved"=0, "Timestamp"=0, "flags"=0, "Reserved 2"=10}, {"X  position"=10.349634, "Y  position"=0.62939304, "Z  position"=0.59408385, "Echo width"=1.68, "Device ID "=120, "Layer"=3, "Echo"=0, "Reserved"=0, "Timestamp"=0, "flags"=0, "Reserved 2"=10}, {"X  position"=10.262678, "Y  position"=0.5916577, "Z  position"=0.30780095, "Echo width"=1.8, "Device ID "=120, "Layer"=0, "Echo"=0, "Reserved"=0, "Timestamp"=0, "flags"=16, "Reserved 2"=10}, {"X  position"=10.234112, "Y  position"=0.5891584, "Z  position"=0.40280667, "Echo width"=1.88, "Device ID "=120, "Layer"=1, "Echo"=0, "Reserved"=0, "Timestamp"=0, "flags"=16, "Reserved 2"=10}, {"X  position"=10.366169, "Y  position"=0.5705346, "Z  position"=0.49810088, "Echo width"=1.4399999, "Device ID "=120, "Layer"=2, "Echo"=0, "Reserved"=0, "Timestamp"=0, "flags"=16, "Reserved 2"=10}, {"X  position"=10.255232, "Y  position"=0.56131643, "Z  position"=0.5919896, "Echo width"=1.48, "Device ID "=120, "Layer"=3, "Echo"=0, "Reserved"=0, "Timestamp"=0, "flags"=16, "Reserved 2"=10}, {"X  position"=10.217749, "Y  position"=0.5286983, "Z  position"=0.30884808, "Echo width"=2.0, "Device ID "=120, "Layer"=0, "Echo"=0, "Reserved"=0, "Timestamp"=0, "flags"=0, "Reserved 2"=10}, {"X  position"=10.229028, "Y  position"=0.529586, "Z  position"=0.4028765, "Echo width"=2.0, "Device ID "=120, "Layer"=1, "Echo"=0, "Reserved"=0, "Timestamp"=0, "flags"=0, "Reserved 2"=10}, {"X  position"=10.380857, "Y  position"=0.51133615, "Z  position"=0.49817067, "Echo width"=1.68, "Device ID "=120, "Layer"=2, "Echo"=0, "Reserved"=0, "Timestamp"=0, "flags"=0, "Reserved 2"=10}, {"X  position"=10.279814, "Y  position"=0.5038272, "Z  position"=0.5924084, "Echo width"=1.76, "Device ID "=120, "Layer"=3, "Echo"=0, "Reserved"=0, "Timestamp"=0, "flags"=4096, "Reserved 2"=10}, {"X  position"=13.96883, "Y  position"=0.7779685, "Z  position"=0.6698954, "Echo width"=0.79999995, "Device ID "=120, "Layer"=3, "Echo"=1, "Reserved"=0, "Timestamp"=0, "flags"=4, "Reserved 2"=0}, {"X  position"=10.23208, "Y  position"=0.4707529, "Z  position"=0.30863866, "Echo width"=1.68, "Device ID "=120, "Layer"=0, "Echo"=0, "Reserved"=0, "Timestamp"=0, "flags"=16, "Reserved 2"=10}, {"X  position"=10.233393, "Y  position"=0.47084472, "Z  position"=0.4028765, "Echo width"=1.92, "Device ID "=120, "Layer"=1, "Echo"=0, "Reserved"=0, "Timestamp"=0, "flags"=16, "Reserved 2"=10}, {"X  position"=10.335167, "Y  position"=0.44800055, "Z  position"=0.49782163, "Echo width"=1.48, "Device ID "=120, "Layer"=2, "Echo"=0, "Reserved"=0, "Timestamp"=0, "flags"=16, "Reserved 2"=10}, {"X  position"=10.264, "Y  position"=0.44333595, "Z  position"=0.5919896, "Echo width"=1.52, "Device ID "=120, "Layer"=3, "Echo"=0, "Reserved"=0, "Timestamp"=0, "flags"=16, "Reserved 2"=10}, {"X  position"=10.225952, "Y  position"=0.41137692, "Z  position"=0.30884808, "Echo width"=2.0, "Device ID "=120, "Layer"=0, "Echo"=0, "Reserved"=0, "Timestamp"=0, "flags"=0, "Reserved 2"=10}, {"X  position"=10.197321, "Y  position"=0.40962574, "Z  position"=0.40315574, "Echo width"=2.04, "Device ID "=120, "Layer"=1, "Echo"=0, "Reserved"=0, "Timestamp"=0, "flags"=0, "Reserved 2"=10}, {"X  position"=10.358784, "Y  position"=0.38946998, "Z  position"=0.49796125, "Echo width"=1.76, "Device ID "=120, "Layer"=2, "Echo"=0, "Reserved"=0, "Timestamp"=0, "flags"=0, "Reserved 2"=10}, {"X  position"=10.287574, "Y  position"=0.3854264, "Z  position"=0.5924084, "Echo width"=1.76, "Device ID "=120, "Layer"=3, "Echo"=0, "Reserved"=0, "Timestamp"=0, "flags"=4096, "Reserved 2"=10}, {"X  position"=13.970831, "Y  position"=0.5945769, "Z  position"=0.66968596, "Echo width"=0.71999997, "Device ID "=120, "Layer"=3, "Echo"=1, "Reserved"=0, "Timestamp"=0, "flags"=4, "Reserved 2"=0}, {"X  position"=10.279207, "Y  position"=0.35528323, "Z  position"=0.30780095, "Echo width"=1.76, "Device ID "=120, "Layer"=0, "Echo"=0, "Reserved"=0, "Timestamp"=0, "flags"=16, "Reserved 2"=10}, {"X  position"=10.240585, "Y  position"=0.35325912, "Z  position"=0.4028765, "Echo width"=1.92, "Device ID "=120, "Layer"=1, "Echo"=0, "Reserved"=0, "Timestamp"=0, "flags"=16, "Reserved 2"=10}, {"X  position"=10.292004, "Y  position"=0.3262433, "Z  position"=0.49747255, "Echo width"=1.4, "Device ID "=120, "Layer"=2, "Echo"=0, "Reserved"=0, "Timestamp"=0, "flags"=16, "Reserved 2"=10}, {"X  position"=10.270706, "Y  position"=0.32522035, "Z  position"=0.5919896, "Echo width"=1.52, "Device ID "=120, "Layer"=3, "Echo"=0, "Reserved"=0, "Timestamp"=0, "flags"=16, "Reserved 2"=10}, {"X  position"=10.232108, "Y  position"=0.2939302, "Z  position"=0.30884808, "Echo width"=2.0, "Device ID "=120, "Layer"=0, "Echo"=0, "Reserved"=0, "Timestamp"=0, "flags"=0, "Reserved 2"=10}, {"X  position"=10.243411, "Y  position"=0.2944237, "Z  position"=0.4028765, "Echo width"=2.0, "Device ID "=120, "Layer"=1, "Echo"=0, "Reserved"=0, "Timestamp"=0, "flags"=0, "Reserved 2"=10}, {"X  position"=10.314575, "Y  position"=0.2677454, "Z  position"=0.49761218, "Echo width"=1.7199999, "Device ID "=120, "Layer"=2, "Echo"=0, "Reserved"=0, "Timestamp"=0, "flags"=0, "Reserved 2"=10}, {"X  position"=10.303257, "Y  position"=0.2673007, "Z  position"=0.59261787, "Echo width"=1.8399999, "Device ID "=120, "Layer"=3, "Echo"=0, "Reserved"=0, "Timestamp"=0, "flags"=4096, "Reserved 2"=10}, {"X  position"=14.019573, "Y  position"=0.41331518, "Z  position"=0.67052364, "Echo width"=0.76, "Device ID "=120, "Layer"=3, "Echo"=1, "Reserved"=0, "Timestamp"=0, "flags"=4, "Reserved 2"=0}, {"X  position"=10.284376, "Y  position"=0.2369156, "Z  position"=0.30780095, "Echo width"=1.76, "Device ID "=120, "Layer"=0, "Echo"=0, "Reserved"=0, "Timestamp"=0, "flags"=16, "Reserved 2"=10}, {"X  position"=10.275704, "Y  position"=0.2366128, "Z  position"=0.40266705, "Echo width"=2.0, "Device ID "=120, "Layer"=1, "Echo"=0, "Reserved"=0, "Timestamp"=0, "flags"=16, "Reserved 2"=10}, {"X  position"=10.346638, "Y  position"=0.20918372, "Z  position"=0.49782163, "Echo width"=1.4399999, "Device ID "=120, "Layer"=2, "Echo"=0, "Reserved"=0, "Timestamp"=0, "flags"=16, "Reserved 2"=10}, {"X  position"=10.275351, "Y  position"=0.2070057, "Z  position"=0.5919896, "Echo width"=1.52, "Device ID "=120, "Layer"=3, "Echo"=0, "Reserved"=0, "Timestamp"=0, "flags"=16, "Reserved 2"=10}, {"X  position"=10.236213, "Y  position"=0.17639394, "Z  position"=0.30884808, "Echo width"=2.04, "Device ID "=120, "Layer"=0, "Echo"=0, "Reserved"=0, "Timestamp"=0, "flags"=0, "Reserved 2"=10}, {"X  position"=10.237526, "Y  position"=0.17642833, "Z  position"=0.4029463, "Echo width"=2.12, "Device ID "=120, "Layer"=1, "Echo"=0, "Reserved"=0, "Timestamp"=0, "flags"=0, "Reserved 2"=10}, {"X  position"=10.328208, "Y  position"=0.14899205, "Z  position"=0.497682, "Echo width"=1.76, "Device ID "=120, "Layer"=2, "Echo"=0, "Reserved"=0, "Timestamp"=0, "flags"=0, "Reserved 2"=10}, {"X  position"=10.216927, "Y  position"=0.14656387, "Z  position"=0.59073305, "Echo width"=1.8, "Device ID "=120, "Layer"=3, "Echo"=0, "Reserved"=0, "Timestamp"=0, "flags"=4096, "Reserved 2"=10}, {"X  position"=14.03518, "Y  position"=0.22987847, "Z  position"=0.6707331, "Echo width"=1.0799999, "Device ID "=120, "Layer"=3, "Echo"=1, "Reserved"=0, "Timestamp"=0, "flags"=0, "Reserved 2"=11}, {"X  position"=10.207506, "Y  position"=0.11707995, "Z  position"=0.30947635, "Echo width"=1.9599999, "Device ID "=120, "Layer"=0, "Echo"=0, "Reserved"=0, "Timestamp"=0, "flags"=16, "Reserved 2"=10}, {"X  position"=10.218813, "Y  position"=0.1172773, "Z  position"=0.40308592, "Echo width"=2.08, "Device ID "=120, "Layer"=1, "Echo"=0, "Reserved"=0, "Timestamp"=0, "flags"=16, "Reserved 2"=10}, {"X  position"=10.309251, "Y  position"=0.08913798, "Z  position"=0.49754238, "Echo width"=1.48, "Device ID "=120, "Layer"=2, "Echo"=0, "Reserved"=0, "Timestamp"=0, "flags"=16, "Reserved 2"=10}, {"X  position"=10.237945, "Y  position"=0.088204525, "Z  position"=0.5911519, "Echo width"=1.52, "Device ID "=120, "Layer"=3, "Echo"=0, "Reserved"=0, "Timestamp"=0, "flags"=4112, "Reserved 2"=10}, {"X  position"=13.796859, "Y  position"=0.13479327, "Z  position"=0.66570693, "Echo width"=0.71999997, "Device ID "=120, "Layer"=3, "Echo"=1, "Reserved"=0, "Timestamp"=0, "flags"=16, "Reserved 2"=11}, {"X  position"=10.268257, "Y  position"=0.059065685, "Z  position"=0.3082198, "Echo width"=2.08, "Device ID "=120, "Layer"=0, "Echo"=0, "Reserved"=0, "Timestamp"=0, "flags"=0, "Reserved 2"=10}, {"X  position"=10.289576, "Y  position"=0.05925173, "Z  position"=0.40259725, "Echo width"=2.04, "Device ID "=120, "Layer"=1, "Echo"=0, "Reserved"=0, "Timestamp"=0, "flags"=0, "Reserved 2"=10}, {"X  position"=10.27977, "Y  position"=0.029582513, "Z  position"=0.49733293, "Echo width"=1.64, "Device ID "=120, "Layer"=2, "Echo"=0, "Reserved"=0, "Timestamp"=0, "flags"=0, "Reserved 2"=10}, {"X  position"=10.298443, "Y  position"=0.029663993, "Z  position"=0.5924084, "Echo width"=1.8, "Device ID "=120, "Layer"=3, "Echo"=0, "Reserved"=0, "Timestamp"=0, "flags"=4096, "Reserved 2"=10}, {"X  position"=13.907618, "Y  position"=0.045412086, "Z  position"=0.6680106, "Echo width"=0.76, "Device ID "=120, "Layer"=3, "Echo"=1, "Reserved"=0, "Timestamp"=0, "flags"=0, "Reserved 2"=11}, {"X  position"=10.288511, "Y  position"=0.0, "Z  position"=0.30780095, "Echo width"=1.92, "Device ID "=120, "Layer"=0, "Echo"=0, "Reserved"=0, "Timestamp"=0, "flags"=16, "Reserved 2"=10}, {"X  position"=10.249836, "Y  position"=0.0, "Z  position"=0.4028765, "Echo width"=1.9599999, "Device ID "=120, "Layer"=1, "Echo"=0, "Reserved"=0, "Timestamp"=0, "flags"=16, "Reserved 2"=10}, {"X  position"=10.299768, "Y  position"=-0.029669777, "Z  position"=0.49747255, "Echo width"=1.4, "Device ID "=120, "Layer"=2, "Echo"=0, "Reserved"=0, "Timestamp"=0, "flags"=16, "Reserved 2"=10}, {"X  position"=10.278448, "Y  position"=-0.029576745, "Z  position"=0.5919896, "Echo width"=1.48, "Device ID "=120, "Layer"=3, "Echo"=0, "Reserved"=0, "Timestamp"=0, "flags"=16, "Reserved 2"=10}, {"X  position"=10.268257, "Y  position"=-0.059065685, "Z  position"=0.3082198, "Echo width"=2.08, "Device ID "=120, "Layer"=0, "Echo"=0, "Reserved"=0, "Timestamp"=0, "flags"=0, "Reserved 2"=10}, {"X  position"=10.249578, "Y  position"=-0.058902677, "Z  position"=0.4028765, "Echo width"=2.04, "Device ID "=120, "Layer"=1, "Echo"=0, "Reserved"=0, "Timestamp"=0, "flags"=0, "Reserved 2"=10}, {"X  position"=10.309251, "Y  position"=-0.08913798, "Z  position"=0.49754238, "Echo width"=1.56, "Device ID "=120, "Layer"=2, "Echo"=0, "Reserved"=0, "Timestamp"=0, "flags"=0, "Reserved 2"=10}, {"X  position"=10.3379135, "Y  position"=-0.0895132, "Z  position"=0.5932461, "Echo width"=1.76, "Device ID "=120, "Layer"=3, "Echo"=0, "Reserved"=0, "Timestamp"=0, "flags"=0, "Reserved 2"=10}, {"X  position"=10.307469, "Y  position"=-0.11882481, "Z  position"=0.3073821, "Echo width"=1.8399999, "Device ID "=120, "Layer"=0, "Echo"=0, "Reserved"=0, "Timestamp"=0, "flags"=16, "Reserved 2"=10}, {"X  position"=10.258805, "Y  position"=-0.11797538, "Z  position"=0.40280667, "Echo width"=1.88, "Device ID "=120, "Layer"=1, "Echo"=0, "Reserved"=0, "Timestamp"=0, "flags"=16, "Reserved 2"=10}, {"X  position"=10.2882185, "Y  position"=-0.14811946, "Z  position"=0.49740273, "Echo width"=1.24, "Device ID "=120, "Layer"=2, "Echo"=0, "Reserved"=0, "Timestamp"=0, "flags"=16, "Reserved 2"=10}, {"X  position"=10.316881, "Y  position"=-0.14874488, "Z  position"=0.5928273, "Echo width"=1.48, "Device ID "=120, "Layer"=3, "Echo"=0, "Reserved"=0, "Timestamp"=0, "flags"=16, "Reserved 2"=10}, {"X  position"=10.316168, "Y  position"=-0.17848763, "Z  position"=0.3071727, "Echo width"=2.0, "Device ID "=120, "Layer"=0, "Echo"=0, "Reserved"=0, "Timestamp"=0, "flags"=0, "Reserved 2"=10}, {"X  position"=10.297503, "Y  position"=-0.17799892, "Z  position"=0.40252742, "Echo width"=1.9599999, "Device ID "=120, "Layer"=1, "Echo"=0, "Reserved"=0, "Timestamp"=0, "flags"=0, "Reserved 2"=10}, {"X  position"=10.376623, "Y  position"=-0.21009985, "Z  position"=0.49803105, "Echo width"=1.88, "Device ID "=120, "Layer"=2, "Echo"=0, "Reserved"=0, "Timestamp"=0, "flags"=0, "Reserved 2"=10}, {"X  position"=10.325317, "Y  position"=-0.2085323, "Z  position"=0.5930367, "Echo width"=1.52, "Device ID "=120, "Layer"=3, "Echo"=0, "Reserved"=0, "Timestamp"=0, "flags"=4096, "Reserved 2"=10}, {"X  position"=14.312581, "Y  position"=-0.3303542, "Z  position"=0.676597, "Echo width"=1.4399999, "Device ID "=120, "Layer"=3, "Echo"=1, "Reserved"=0, "Timestamp"=0, "flags"=4, "Reserved 2"=0}, {"X  position"=10.324343, "Y  position"=-0.23831126, "Z  position"=0.30696326, "Echo width"=1.68, "Device ID "=120, "Layer"=0, "Echo"=0, "Reserved"=0, "Timestamp"=0, "flags"=16, "Reserved 2"=10}, {"X  position"=10.2956915, "Y  position"=-0.23731077, "Z  position"=0.40252742, "Echo width"=1.7199999, "Device ID "=120, "Layer"=1, "Echo"=0, "Reserved"=0, "Timestamp"=0, "flags"=16, "Reserved 2"=10}, {"X  position"=10.504425, "Y  position"=-0.2752046, "Z  position"=0.49893862, "Echo width"=1.68, "Device ID "=120, "Layer"=2, "Echo"=0, "Reserved"=0, "Timestamp"=0, "flags"=16, "Reserved 2"=10}, {"X  position"=10.423138, "Y  position"=-0.27201083, "Z  position"=0.5951309, "Echo width"=1.1999999, "Device ID "=120, "Layer"=3, "Echo"=0, "Reserved"=0, "Timestamp"=0, "flags"=16, "Reserved 2"=10}, {"X  position"=10.361956, "Y  position"=-0.29959947, "Z  position"=0.30612558, "Echo width"=1.88, "Device ID "=120, "Layer"=0, "Echo"=0, "Reserved"=0, "Timestamp"=0, "flags"=0, "Reserved 2"=10}, {"X  position"=10.393265, "Y  position"=-0.30096644, "Z  position"=0.4018293, "Echo width"=1.8, "Device ID "=120, "Layer"=1, "Echo"=0, "Reserved"=0, "Timestamp"=0, "flags"=0, "Reserved 2"=10}, {"X  position"=10.48178, "Y  position"=-0.33535895, "Z  position"=0.498799, "Echo width"=1.8, "Device ID "=120, "Layer"=2, "Echo"=0, "Reserved"=0, "Timestamp"=0, "flags"=0, "Reserved 2"=10}, {"X  position"=10.560308, "Y  position"=-0.33913097, "Z  position"=0.5980629, "Echo width"=1.5999999, "Device ID "=120, "Layer"=3, "Echo"=0, "Reserved"=0, "Timestamp"=0, "flags"=0, "Reserved 2"=10}, {"X  position"=10.399015, "Y  position"=-0.36156213, "Z  position"=0.30528787, "Echo width"=1.52, "Device ID "=120, "Layer"=0, "Echo"=0, "Reserved"=0, "Timestamp"=0, "flags"=16, "Reserved 2"=10}, {"X  position"=10.410348, "Y  position"=-0.362156, "Z  position"=0.40168968, "Echo width"=1.56, "Device ID "=120, "Layer"=1, "Echo"=0, "Reserved"=0, "Timestamp"=0, "flags"=16, "Reserved 2"=10}, {"X  position"=10.45862, "Y  position"=-0.3951391, "Z  position"=0.49865937, "Echo width"=1.48, "Device ID "=120, "Layer"=2, "Echo"=0, "Reserved"=0, "Timestamp"=0, "flags"=16, "Reserved 2"=10}, {"X  position"=10.6568985, "Y  position"=-0.40639815, "Z  position"=0.60015714, "Echo width"=1.24, "Device ID "=120, "Layer"=3, "Echo"=0, "Reserved"=0, "Timestamp"=0, "flags"=16, "Reserved 2"=10}, {"X  position"=10.515348, "Y  position"=-0.4290771, "Z  position"=0.3027748, "Echo width"=1.5999999, "Device ID "=120, "Layer"=0, "Echo"=0, "Reserved"=0, "Timestamp"=0, "flags"=0, "Reserved 2"=10}, {"X  position"=10.546659, "Y  position"=-0.4309922, "Z  position"=0.40071228, "Echo width"=1.5999999, "Device ID "=120, "Layer"=1, "Echo"=0, "Reserved"=0, "Timestamp"=0, "flags"=0, "Reserved 2"=10}, {"X  position"=10.664453, "Y  position"=-0.46958303, "Z  position"=0.5001254, "Echo width"=1.3199999, "Device ID "=120, "Layer"=2, "Echo"=0, "Reserved"=0, "Timestamp"=0, "flags"=0, "Reserved 2"=10}, {"X  position"=10.792748, "Y  position"=-0.47799203, "Z  position"=0.6030891, "Echo width"=1.56, "Device ID "=120, "Layer"=3, "Echo"=0, "Reserved"=0, "Timestamp"=0, "flags"=0, "Reserved 2"=10}, {"X  position"=19.278002, "Y  position"=-1.1033052, "Z  position"=0.11869091, "Echo width"=1.0799999, "Device ID "=120, "Layer"=0, "Echo"=0, "Reserved"=0, "Timestamp"=0, "flags"=1, "Reserved 2"=0}, {"X  position"=10.831917, "Y  position"=-0.5126975, "Z  position"=0.39868772, "Echo width"=1.24, "Device ID "=120, "Layer"=1, "Echo"=0, "Reserved"=0, "Timestamp"=0, "flags"=4116, "Reserved 2"=0}, {"X  position"=19.590315, "Y  position"=-1.1251444, "Z  position"=0.33739227, "Echo width"=0.96, "Device ID "=120, "Layer"=1, "Echo"=1, "Reserved"=0, "Timestamp"=0, "flags"=1, "Reserved 2"=0}, {"X  position"=17.610744, "Y  position"=-1.0486096, "Z  position"=0.5487848, "Echo width"=1.1999999, "Device ID "=120, "Layer"=2, "Echo"=0, "Reserved"=0, "Timestamp"=0, "flags"=4112, "Reserved 2"=12}, {"X  position"=20.383036, "Y  position"=-1.2546263, "Z  position"=0.5681927, "Echo width"=1.1999999, "Device ID "=120, "Layer"=2, "Echo"=1, "Reserved"=0, "Timestamp"=0, "flags"=1, "Reserved 2"=0}, {"X  position"=14.228059, "Y  position"=-0.7972325, "Z  position"=0.6753404, "Echo width"=2.8799999, "Device ID "=120, "Layer"=3, "Echo"=0, "Reserved"=0, "Timestamp"=0, "flags"=16, "Reserved 2"=13}, {"X  position"=17.962097, "Y  position"=-1.1381918, "Z  position"=0.1461255, "Echo width"=1.64, "Device ID "=120, "Layer"=0, "Echo"=0, "Reserved"=0, "Timestamp"=0, "flags"=0, "Reserved 2"=12}, {"X  position"=18.034698, "Y  position"=-1.1439058, "Z  position"=0.34821323, "Echo width"=1.68, "Device ID "=120, "Layer"=1, "Echo"=0, "Reserved"=0, "Timestamp"=0, "flags"=0, "Reserved 2"=12}, {"X  position"=14.591503, "Y  position"=-0.9216328, "Z  position"=0.52770144, "Echo width"=1.1999999, "Device ID "=120, "Layer"=2, "Echo"=0, "Reserved"=0, "Timestamp"=0, "flags"=4096, "Reserved 2"=13}, {"X  position"=17.640919, "Y  position"=-1.1750197, "Z  position"=0.54906404, "Echo width"=1.76, "Device ID "=120, "Layer"=2, "Echo"=1, "Reserved"=0, "Timestamp"=0, "flags"=0, "Reserved 2"=12}, {"X  position"=14.061276, "Y  position"=-0.8775744, "Z  position"=0.6719896, "Echo width"=2.6799998, "Device ID "=120, "Layer"=3, "Echo"=0, "Reserved"=0, "Timestamp"=0, "flags"=0, "Reserved 2"=13}, {"X  position"=17.473545, "Y  position"=-1.2225269, "Z  position"=0.15617785, "Echo width"=1.8, "Device ID "=120, "Layer"=0, "Echo"=0, "Reserved"=0, "Timestamp"=0, "flags"=16, "Reserved 2"=12}, {"X  position"=14.308449, "Y  position"=-0.9456168, "Z  position"=0.37425333, "Echo width"=0.71999997, "Device ID "=120, "Layer"=1, "Echo"=0, "Reserved"=0, "Timestamp"=0, "flags"=4112, "Reserved 2"=13}, {"X  position"=17.40654, "Y  position"=-1.2166646, "Z  position"=0.3525416, "Echo width"=1.7199999, "Device ID "=120, "Layer"=1, "Echo"=1, "Reserved"=0, "Timestamp"=0, "flags"=16, "Reserved 2"=12}, {"X  position"=14.602954, "Y  position"=-1.0202183, "Z  position"=0.52784103, "Echo width"=1.88, "Device ID "=120, "Layer"=2, "Echo"=0, "Reserved"=0, "Timestamp"=0, "flags"=4112, "Reserved 2"=13}, {"X  position"=17.510632, "Y  position"=-1.2873964, "Z  position"=0.5482263, "Echo width"=1.3199999, "Device ID "=120, "Layer"=2, "Echo"=1, "Reserved"=0, "Timestamp"=0, "flags"=16, "Reserved 2"=12}, {"X  position"=14.531098, "Y  position"=-1.0136156, "Z  position"=0.682042, "Echo width"=2.8799999, "Device ID "=120, "Layer"=3, "Echo"=0, "Reserved"=0, "Timestamp"=0, "flags"=16, "Reserved 2"=13}, {"X  position"=17.273262, "Y  position"=-1.3262143, "Z  position"=0.1601569, "Echo width"=1.76, "Device ID "=120, "Layer"=0, "Echo"=0, "Reserved"=0, "Timestamp"=0, "flags"=0, "Reserved 2"=12}, {"X  position"=17.475021, "Y  position"=-1.3456415, "Z  position"=0.3519831, "Echo width"=1.9599999, "Device ID "=120, "Layer"=1, "Echo"=0, "Reserved"=0, "Timestamp"=0, "flags"=0, "Reserved 2"=12}, {"X  position"=17.41927, "Y  position"=-1.4015969, "Z  position"=0.5476678, "Echo width"=1.76, "Device ID "=120, "Layer"=2, "Echo"=0, "Reserved"=0, "Timestamp"=0, "flags"=0, "Reserved 2"=12}, {"X  position"=14.362673, "Y  position"=-1.0938137, "Z  position"=0.6786912, "Echo width"=1.9599999, "Device ID "=120, "Layer"=3, "Echo"=0, "Reserved"=0, "Timestamp"=0, "flags"=0, "Reserved 2"=13}, {"X  position"=14.337911, "Y  position"=-1.1391103, "Z  position"=0.22172762, "Echo width"=1.36, "Device ID "=120, "Layer"=0, "Echo"=0, "Reserved"=0, "Timestamp"=0, "flags"=16, "Reserved 2"=13}, {"X  position"=14.359915, "Y  position"=-1.141423, "Z  position"=0.37376463, "Echo width"=1.56, "Device ID "=120, "Layer"=1, "Echo"=0, "Reserved"=0, "Timestamp"=0, "flags"=16, "Reserved 2"=13}, {"X  position"=14.056622, "Y  position"=-1.1561381, "Z  position"=0.52414095, "Echo width"=1.0, "Device ID "=120, "Layer"=2, "Echo"=0, "Reserved"=0, "Timestamp"=0, "flags"=16, "Reserved 2"=13}, {"X  position"=14.153946, "Y  position"=-1.1667968, "Z  position"=0.67450273, "Echo width"=0.96, "Device ID "=120, "Layer"=3, "Echo"=0, "Reserved"=0, "Timestamp"=0, "flags"=16, "Reserved 2"=13}, {"X  position"=13.085866, "Y  position"=-1.0921714, "Z  position"=0.24790564, "Echo width"=1.48, "Device ID "=120, "Layer"=0, "Echo"=0, "Reserved"=0, "Timestamp"=0, "flags"=1, "Reserved 2"=0}, {"X  position"=13.435476, "Y  position"=-1.1320046, "Z  position"=0.3801874, "Echo width"=1.3199999, "Device ID "=120, "Layer"=1, "Echo"=0, "Reserved"=0, "Timestamp"=0, "flags"=4097, "Reserved 2"=0}, {"X  position"=21.383858, "Y  position"=-2.0376084, "Z  position"=0.3243373, "Echo width"=1.3199999, "Device ID "=120, "Layer"=1, "Echo"=1, "Reserved"=0, "Timestamp"=0, "flags"=1, "Reserved 2"=0}, {"X  position"=13.996477, "Y  position"=-1.2423401, "Z  position"=0.5237919, "Echo width"=1.52, "Device ID "=120, "Layer"=2, "Echo"=0, "Reserved"=0, "Timestamp"=0, "flags"=0, "Reserved 2"=13}, {"X  position"=14.1334305, "Y  position"=-1.2585495, "Z  position"=0.6742933, "Echo width"=1.52, "Device ID "=120, "Layer"=3, "Echo"=0, "Reserved"=0, "Timestamp"=0, "flags"=0, "Reserved 2"=13}, {"X  position"=12.123333, "Y  position"=-1.0588123, "Z  position"=0.26801038, "Echo width"=1.28, "Device ID "=120, "Layer"=0, "Echo"=0, "Reserved"=0, "Timestamp"=0, "flags"=17, "Reserved 2"=0}, {"X  position"=12.422771, "Y  position"=-1.0955787, "Z  position"=0.38723844, "Echo width"=1.12, "Device ID "=120, "Layer"=1, "Echo"=0, "Reserved"=0, "Timestamp"=0, "flags"=16, "Reserved 2"=14}, {"X  position"=12.556785, "Y  position"=-1.1521685, "Z  position"=0.5137389, "Echo width"=0.79999995, "Device ID "=120, "Layer"=2, "Echo"=0, "Reserved"=0, "Timestamp"=0, "flags"=16, "Reserved 2"=14}, {"X  position"=14.508839, "Y  position"=-1.4005011, "Z  position"=0.68246084, "Echo width"=1.4, "Device ID "=120, "Layer"=3, "Echo"=0, "Reserved"=0, "Timestamp"=0, "flags"=16, "Reserved 2"=13}, {"X  position"=11.667714, "Y  position"=-1.0753, "Z  position"=0.27743447, "Echo width"=1.7199999, "Device ID "=120, "Layer"=0, "Echo"=0, "Reserved"=0, "Timestamp"=0, "flags"=4, "Reserved 2"=0}, {"X  position"=11.689136, "Y  position"=-1.0781202, "Z  position"=0.3923348, "Echo width"=1.76, "Device ID "=120, "Layer"=1, "Echo"=0, "Reserved"=0, "Timestamp"=0, "flags"=4, "Reserved 2"=0}, {"X  position"=11.525818, "Y  position"=-1.0922658, "Z  position"=0.50654817, "Echo width"=1.7199999, "Device ID "=120, "Layer"=2, "Echo"=0, "Reserved"=0, "Timestamp"=0, "flags"=4, "Reserved 2"=0}, {"X  position"=11.544065, "Y  position"=-1.0947493, "Z  position"=0.62005246, "Echo width"=1.76, "Device ID "=120, "Layer"=3, "Echo"=0, "Reserved"=0, "Timestamp"=0, "flags"=1, "Reserved 2"=0}, {"X  position"=11.267059, "Y  position"=-1.12617, "Z  position"=0.614398, "Echo width"=1.1999999, "Device ID "=120, "Layer"=3, "Echo"=0, "Reserved"=0, "Timestamp"=0, "flags"=17, "Reserved 2"=0}, {"X  position"=10.995096, "Y  position"=-1.1201496, "Z  position"=0.29125643, "Echo width"=1.0, "Device ID "=120, "Layer"=0, "Echo"=0, "Reserved"=0, "Timestamp"=0, "flags"=1, "Reserved 2"=0}, {"X  position"=11.237173, "Y  position"=-1.1908649, "Z  position"=0.6139791, "Echo width"=1.52, "Device ID "=120, "Layer"=3, "Echo"=0, "Reserved"=0, "Timestamp"=0, "flags"=0, "Reserved 2"=15}, {"X  position"=11.16728, "Y  position"=-1.248696, "Z  position"=0.6127226, "Echo width"=1.12, "Device ID "=120, "Layer"=3, "Echo"=0, "Reserved"=0, "Timestamp"=0, "flags"=16, "Reserved 2"=15}, {"X  position"=10.757469, "Y  position"=-1.2144839, "Z  position"=0.2958638, "Echo width"=0.91999996, "Device ID "=120, "Layer"=0, "Echo"=0, "Reserved"=0, "Timestamp"=0, "flags"=1, "Reserved 2"=0}, {"X  position"=10.827923, "Y  position"=-1.2262738, "Z  position"=0.39812922, "Echo width"=0.68, "Device ID "=120, "Layer"=1, "Echo"=0, "Reserved"=0, "Timestamp"=0, "flags"=4, "Reserved 2"=0}, {"X  position"=10.990044, "Y  position"=-1.2870249, "Z  position"=0.50305754, "Echo width"=1.8399999, "Device ID "=120, "Layer"=2, "Echo"=0, "Reserved"=0, "Timestamp"=0, "flags"=0, "Reserved 2"=15}, {"X  position"=11.116677, "Y  position"=-1.3087845, "Z  position"=0.6118849, "Echo width"=1.36, "Device ID "=120, "Layer"=3, "Echo"=0, "Reserved"=0, "Timestamp"=0, "flags"=4096, "Reserved 2"=15}, {"X  position"=14.289472, "Y  position"=-1.8539704, "Z  position"=0.6793195, "Echo width"=1.52, "Device ID "=120, "Layer"=3, "Echo"=1, "Reserved"=0, "Timestamp"=0, "flags"=4, "Reserved 2"=0}, {"X  position"=10.919486, "Y  position"=-1.3416617, "Z  position"=0.5026387, "Echo width"=1.56, "Device ID "=120, "Layer"=2, "Echo"=0, "Reserved"=0, "Timestamp"=0, "flags"=16, "Reserved 2"=15}, {"X  position"=11.026259, "Y  position"=-1.3609694, "Z  position"=0.61020947, "Echo width"=1.1999999, "Device ID "=120, "Layer"=3, "Echo"=0, "Reserved"=0, "Timestamp"=0, "flags"=16, "Reserved 2"=15}, {"X  position"=10.76466, "Y  position"=-1.3464252, "Z  position"=0.2952355, "Echo width"=1.12, "Device ID "=120, "Layer"=0, "Echo"=0, "Reserved"=0, "Timestamp"=0, "flags"=4, "Reserved 2"=0}, {"X  position"=10.805406, "Y  position"=-1.3539768, "Z  position"=0.39812922, "Echo width"=1.12, "Device ID "=120, "Layer"=1, "Echo"=0, "Reserved"=0, "Timestamp"=0, "flags"=4, "Reserved 2"=0}, {"X  position"=10.828901, "Y  position"=-1.3914355, "Z  position"=0.5020802, "Echo width"=1.64, "Device ID "=120, "Layer"=2, "Echo"=0, "Reserved"=0, "Timestamp"=0, "flags"=0, "Reserved 2"=15}, {"X  position"=10.974808, "Y  position"=-1.4191365, "Z  position"=0.6093718, "Echo width"=1.3199999, "Device ID "=120, "Layer"=3, "Echo"=0, "Reserved"=0, "Timestamp"=0, "flags"=4096, "Reserved 2"=15}, {"X  position"=14.16707, "Y  position"=-2.0252068, "Z  position"=0.6774347, "Echo width"=1.48, "Device ID "=120, "Layer"=3, "Echo"=1, "Reserved"=0, "Timestamp"=0, "flags"=4, "Reserved 2"=0}, {"X  position"=10.864081, "Y  position"=-1.4648069, "Z  position"=0.6072776, "Echo width"=0.91999996, "Device ID "=120, "Layer"=3, "Echo"=0, "Reserved"=0, "Timestamp"=0, "flags"=16, "Reserved 2"=15}, {"X  position"=10.740055, "Y  position"=-1.4730059, "Z  position"=0.2952355, "Echo width"=1.16, "Device ID "=120, "Layer"=0, "Echo"=0, "Reserved"=0, "Timestamp"=0, "flags"=4, "Reserved 2"=0}, {"X  position"=10.7414665, "Y  position"=-1.4732931, "Z  position"=0.39840847, "Echo width"=1.16, "Device ID "=120, "Layer"=1, "Echo"=0, "Reserved"=0, "Timestamp"=0, "flags"=4, "Reserved 2"=0}, {"X  position"=10.803501, "Y  position"=-1.5191305, "Z  position"=0.5020802, "Echo width"=1.28, "Device ID "=120, "Layer"=2, "Echo"=0, "Reserved"=0, "Timestamp"=0, "flags"=4, "Reserved 2"=0}, {"X  position"=10.8803835, "Y  position"=-1.535122, "Z  position"=0.60790586, "Echo width"=1.48, "Device ID "=120, "Layer"=3, "Echo"=0, "Reserved"=0, "Timestamp"=0, "flags"=4096, "Reserved 2"=15}, {"X  position"=14.276927, "Y  position"=-2.241604, "Z  position"=0.680576, "Echo width"=1.28, "Device ID "=120, "Layer"=3, "Echo"=1, "Reserved"=0, "Timestamp"=0, "flags"=4, "Reserved 2"=0}, {"X  position"=10.847166, "Y  position"=-1.5952262, "Z  position"=0.60748696, "Echo width"=1.04, "Device ID "=120, "Layer"=3, "Echo"=0, "Reserved"=0, "Timestamp"=0, "flags"=16, "Reserved 2"=15}, {"X  position"=10.644918, "Y  position"=-1.5839905, "Z  position"=0.2967015, "Echo width"=1.3199999, "Device ID "=120, "Layer"=0, "Echo"=0, "Reserved"=0, "Timestamp"=0, "flags"=0, "Reserved 2"=15}, {"X  position"=10.597499, "Y  position"=-1.5734776, "Z  position"=0.39924622, "Echo width"=1.24, "Device ID "=120, "Layer"=1, "Echo"=0, "Reserved"=0, "Timestamp"=0, "flags"=0, "Reserved 2"=15}, {"X  position"=10.746616, "Y  position"=-1.639742, "Z  position"=0.50187075, "Echo width"=1.8, "Device ID "=120, "Layer"=2, "Echo"=0, "Reserved"=0, "Timestamp"=0, "flags"=0, "Reserved 2"=15}, {"X  position"=10.823214, "Y  position"=-1.6570742, "Z  position"=0.6072776, "Echo width"=1.52, "Device ID "=120, "Layer"=3, "Echo"=0, "Reserved"=0, "Timestamp"=0, "flags"=4096, "Reserved 2"=15}, {"X  position"=14.197158, "Y  position"=-2.4205198, "Z  position"=0.6797383, "Echo width"=1.3199999, "Device ID "=120, "Layer"=3, "Echo"=1, "Reserved"=0, "Timestamp"=0, "flags"=4, "Reserved 2"=0}, {"X  position"=10.630824, "Y  position"=-1.6462805, "Z  position"=0.2967015, "Echo width"=1.1999999, "Device ID "=120, "Layer"=0, "Echo"=0, "Reserved"=0, "Timestamp"=0, "flags"=16, "Reserved 2"=15}, {"X  position"=10.690676, "Y  position"=-1.6600983, "Z  position"=0.3984783, "Echo width"=1.0, "Device ID "=120, "Layer"=1, "Echo"=0, "Reserved"=0, "Timestamp"=0, "flags"=16, "Reserved 2"=15}, {"X  position"=10.8099, "Y  position"=-1.7212529, "Z  position"=0.50242925, "Echo width"=1.0799999, "Device ID "=120, "Layer"=2, "Echo"=0, "Reserved"=0, "Timestamp"=0, "flags"=16, "Reserved 2"=15}, {"X  position"=10.77928, "Y  position"=-1.7140429, "Z  position"=0.6066493, "Echo width"=1.0, "Device ID "=120, "Layer"=3, "Echo"=0, "Reserved"=0, "Timestamp"=0, "flags"=16, "Reserved 2"=15}, {"X  position"=10.655072, "Y  position"=-1.717781, "Z  position"=0.2958638, "Echo width"=1.76, "Device ID "=120, "Layer"=0, "Echo"=0, "Reserved"=0, "Timestamp"=0, "flags"=0, "Reserved 2"=15}, {"X  position"=10.646744, "Y  position"=-1.7157817, "Z  position"=0.39868772, "Echo width"=2.0, "Device ID "=120, "Layer"=1, "Echo"=0, "Reserved"=0, "Timestamp"=0, "flags"=0, "Reserved 2"=15}, {"X  position"=10.804315, "Y  position"=-1.7873545, "Z  position"=0.50249904, "Echo width"=1.48, "Device ID "=120, "Layer"=2, "Echo"=0, "Reserved"=0, "Timestamp"=0, "flags"=0, "Reserved 2"=15}, {"X  position"=10.793179, "Y  position"=-1.7846295, "Z  position"=0.6072776, "Echo width"=1.52, "Device ID "=120, "Layer"=3, "Echo"=0, "Reserved"=0, "Timestamp"=0, "flags"=4096, "Reserved 2"=15}, {"X  position"=14.386356, "Y  position"=-2.6638746, "Z  position"=0.6847645, "Echo width"=1.4, "Device ID "=120, "Layer"=3, "Echo"=1, "Reserved"=0, "Timestamp"=0, "flags"=4, "Reserved 2"=0}, {"X  position"=10.668913, "Y  position"=-1.7874107, "Z  position"=0.2952355, "Echo width"=1.52, "Device ID "=120, "Layer"=0, "Echo"=0, "Reserved"=0, "Timestamp"=0, "flags"=16, "Reserved 2"=15}, {"X  position"=10.6315, "Y  position"=-1.7780826, "Z  position"=0.39868772, "Echo width"=1.92, "Device ID "=120, "Layer"=1, "Echo"=0, "Reserved"=0, "Timestamp"=0, "flags"=16, "Reserved 2"=15}, {"X  position"=10.807823, "Y  position"=-1.8559506, "Z  position"=0.5026387, "Echo width"=0.96, "Device ID "=120, "Layer"=2, "Echo"=0, "Reserved"=0, "Timestamp"=0, "flags"=16, "Reserved 2"=15}, {"X  position"=10.738566, "Y  position"=-1.8383617, "Z  position"=0.6064398, "Echo width"=0.88, "Device ID "=120, "Layer"=3, "Echo"=0, "Reserved"=0, "Timestamp"=0, "flags"=16, "Reserved 2"=15}, {"X  position"=10.624002, "Y  position"=-1.8423926, "Z  position"=0.2958638, "Echo width"=1.7199999, "Device ID "=120, "Layer"=0, "Echo"=0, "Reserved"=0, "Timestamp"=0, "flags"=0, "Reserved 2"=15}, {"X  position"=10.615711, "Y  position"=-1.8402481, "Z  position"=0.39868772, "Echo width"=2.04, "Device ID "=120, "Layer"=1, "Echo"=0, "Reserved"=0, "Timestamp"=0, "flags"=0, "Reserved 2"=15}, {"X  position"=10.84937, "Y  position"=-1.9349276, "Z  position"=0.50305754, "Echo width"=1.48, "Device ID "=120, "Layer"=2, "Echo"=0, "Reserved"=0, "Timestamp"=0, "flags"=0, "Reserved 2"=15}, {"X  position"=10.780258, "Y  position"=-1.9167321, "Z  position"=0.6076964, "Echo width"=1.4, "Device ID "=120, "Layer"=3, "Echo"=0, "Reserved"=0, "Timestamp"=0, "flags"=4096, "Reserved 2"=15}, {"X  position"=14.183514, "Y  position"=-2.8127344, "Z  position"=0.6814137, "Echo width"=1.28, "Device ID "=120, "Layer"=3, "Echo"=1, "Reserved"=0, "Timestamp"=0, "flags"=4, "Reserved 2"=0}, {"X  position"=10.636626, "Y  position"=-1.9122533, "Z  position"=0.2952355, "Echo width"=1.52, "Device ID "=120, "Layer"=0, "Echo"=0, "Reserved"=0, "Timestamp"=0, "flags"=16, "Reserved 2"=15}, {"X  position"=10.60904, "Y  position"=-1.9048617, "Z  position"=0.39861792, "Echo width"=1.88, "Device ID "=120, "Layer"=1, "Echo"=0, "Reserved"=0, "Timestamp"=0, "flags"=16, "Reserved 2"=15}, {"X  position"=10.822557, "Y  position"=-1.9963582, "Z  position"=0.50298774, "Echo width"=1.12, "Device ID "=120, "Layer"=2, "Echo"=0, "Reserved"=0, "Timestamp"=0, "flags"=16, "Reserved 2"=15}, {"X  position"=10.782546, "Y  position"=-1.98545, "Z  position"=0.60811526, "Echo width"=0.79999995, "Device ID "=120, "Layer"=3, "Echo"=0, "Reserved"=0, "Timestamp"=0, "flags"=4112, "Reserved 2"=15}, {"X  position"=14.669786, "Y  position"=-3.0452335, "Z  position"=0.6925132, "Echo width"=1.4399999, "Device ID "=120, "Layer"=3, "Echo"=1, "Reserved"=0, "Timestamp"=0, "flags"=16, "Reserved 2"=16}, {"X  position"=10.658203, "Y  position"=-1.9851456, "Z  position"=0.29439783, "Echo width"=1.88, "Device ID "=120, "Layer"=0, "Echo"=0, "Reserved"=0, "Timestamp"=0, "flags"=0, "Reserved 2"=15}, {"X  position"=10.621056, "Y  position"=-1.9748434, "Z  position"=0.39840847, "Echo width"=2.0, "Device ID "=120, "Layer"=1, "Echo"=0, "Reserved"=0, "Timestamp"=0, "flags"=0, "Reserved 2"=15}, {"X  position"=10.814481, "Y  position"=-2.062897, "Z  position"=0.50305754, "Echo width"=1.4399999, "Device ID "=120, "Layer"=2, "Echo"=0, "Reserved"=0, "Timestamp"=0, "flags"=0, "Reserved 2"=15}, {"X  position"=10.755321, "Y  position"=-2.0462122, "Z  position"=0.60790586, "Echo width"=1.48, "Device ID "=120, "Layer"=3, "Echo"=0, "Reserved"=0, "Timestamp"=0, "flags"=4096, "Reserved 2"=15}, {"X  position"=14.546562, "Y  position"=-3.1154528, "Z  position"=0.69041896, "Echo width"=1.76, "Device ID "=120, "Layer"=3, "Echo"=1, "Reserved"=0, "Timestamp"=0, "flags"=0, "Reserved 2"=16}, {"X  position"=10.640608, "Y  position"=-2.0475364, "Z  position"=0.29439783, "Echo width"=1.56, "Device ID "=120, "Layer"=0, "Echo"=0, "Reserved"=0, "Timestamp"=0, "flags"=16, "Reserved 2"=15}, {"X  position"=10.60355, "Y  position"=-2.0369103, "Z  position"=0.39840847, "Echo width"=1.92, "Device ID "=120, "Layer"=1, "Echo"=0, "Reserved"=0, "Timestamp"=0, "flags"=16, "Reserved 2"=15}, {"X  position"=10.777, "Y  position"=-2.1210523, "Z  position"=0.50291795, "Echo width"=0.91999996, "Device ID "=120, "Layer"=2, "Echo"=0, "Reserved"=0, "Timestamp"=0, "flags"=16, "Reserved 2"=15}, {"X  position"=10.871565, "Y  position"=-2.1486154, "Z  position"=0.61083776, "Echo width"=1.04, "Device ID "=120, "Layer"=3, "Echo"=0, "Reserved"=0, "Timestamp"=0, "flags"=4112, "Reserved 2"=15}, {"X  position"=14.173412, "Y  position"=-3.111016, "Z  position"=0.6828797, "Echo width"=1.0, "Device ID "=120, "Layer"=3, "Echo"=1, "Reserved"=0, "Timestamp"=0, "flags"=16, "Reserved 2"=16}, {"X  position"=10.670399, "Y  position"=-2.1239688, "Z  position"=0.2933507, "Echo width"=1.68, "Device ID "=120, "Layer"=0, "Echo"=0, "Reserved"=0, "Timestamp"=0, "flags"=0, "Reserved 2"=15}, {"X  position"=10.585505, "Y  position"=-2.0988224, "Z  position"=0.39840847, "Echo width"=2.0, "Device ID "=120, "Layer"=1, "Echo"=0, "Reserved"=0, "Timestamp"=0, "flags"=0, "Reserved 2"=15}, {"X  position"=10.815666, "Y  position"=-2.201766, "Z  position"=0.5033368, "Echo width"=1.4399999, "Device ID "=120, "Layer"=2, "Echo"=0, "Reserved"=0, "Timestamp"=0, "flags"=0, "Reserved 2"=15}, {"X  position"=10.871681, "Y  position"=-2.2186246, "Z  position"=0.6112566, "Echo width"=1.4399999, "Device ID "=120, "Layer"=3, "Echo"=0, "Reserved"=0, "Timestamp"=0, "flags"=4096, "Reserved 2"=15}, {"X  position"=14.097989, "Y  position"=-3.1896331, "Z  position"=0.68183255, "Echo width"=1.64, "Device ID "=120, "Layer"=3, "Echo"=1, "Reserved"=0, "Timestamp"=0, "flags"=0, "Reserved 2"=16}, {"X  position"=10.642029, "Y  position"=-2.1835377, "Z  position"=0.29356012, "Echo width"=1.48, "Device ID "=120, "Layer"=0, "Echo"=0, "Reserved"=0, "Timestamp"=0, "flags"=16, "Reserved 2"=15}, {"X  position"=10.643422, "Y  position"=-2.1839635, "Z  position"=0.39784998, "Echo width"=1.92, "Device ID "=120, "Layer"=1, "Echo"=0, "Reserved"=0, "Timestamp"=0, "flags"=16, "Reserved 2"=15}, {"X  position"=10.824824, "Y  position"=-2.2744186, "Z  position"=0.50354624, "Echo width"=1.12, "Device ID "=120, "Layer"=2, "Echo"=0, "Reserved"=0, "Timestamp"=0, "flags"=16, "Reserved 2"=15}, {"X  position"=10.909328, "Y  position"=-2.300658, "Z  position"=0.6125132, "Echo width"=1.04, "Device ID "=120, "Layer"=3, "Echo"=0, "Reserved"=0, "Timestamp"=0, "flags"=4112, "Reserved 2"=15}, {"X  position"=14.088848, "Y  position"=-3.287925, "Z  position"=0.68225145, "Echo width"=1.12, "Device ID "=120, "Layer"=3, "Echo"=1, "Reserved"=0, "Timestamp"=0, "flags"=16, "Reserved 2"=16}, {"X  position"=10.748072, "Y  position"=-2.2853081, "Z  position"=0.3969424, "Echo width"=0.88, "Device ID "=120, "Layer"=1, "Echo"=0, "Reserved"=0, "Timestamp"=0, "flags"=0, "Reserved 2"=15}, {"X  position"=10.728508, "Y  position"=-2.3138638, "Z  position"=0.50298774, "Echo width"=1.04, "Device ID "=120, "Layer"=2, "Echo"=0, "Reserved"=0, "Timestamp"=0, "flags"=0, "Reserved 2"=15}, {"X  position"=10.84136, "Y  position"=-2.3499882, "Z  position"=0.61146605, "Echo width"=1.64, "Device ID "=120, "Layer"=3, "Echo"=0, "Reserved"=0, "Timestamp"=0, "flags"=4096, "Reserved 2"=15}, {"X  position"=14.35493, "Y  position"=-3.4746907, "Z  position"=0.6887436, "Echo width"=1.1999999, "Device ID "=120, "Layer"=3, "Echo"=1, "Reserved"=0, "Timestamp"=0, "flags"=0, "Reserved 2"=16}, {"X  position"=10.716936, "Y  position"=-2.3449244, "Z  position"=0.29104704, "Echo width"=1.04, "Device ID "=120, "Layer"=0, "Echo"=0, "Reserved"=0, "Timestamp"=0, "flags"=16, "Reserved 2"=15}, {"X  position"=11.200371, "Y  position"=-2.5392015, "Z  position"=0.619843, "Echo width"=1.7199999, "Device ID "=120, "Layer"=3, "Echo"=0, "Reserved"=0, "Timestamp"=0, "flags"=16, "Reserved 2"=15}, {"X  position"=10.667754, "Y  position"=-2.398297, "Z  position"=0.2916753, "Echo width"=0.88, "Device ID "=120, "Layer"=0, "Echo"=0, "Reserved"=0, "Timestamp"=0, "flags"=0, "Reserved 2"=15}, {"X  position"=10.659669, "Y  position"=-2.3955917, "Z  position"=0.39729148, "Echo width"=0.79999995, "Device ID "=120, "Layer"=1, "Echo"=0, "Reserved"=0, "Timestamp"=0, "flags"=4, "Reserved 2"=0}, {"X  position"=10.791183, "Y  position"=-2.4750233, "Z  position"=0.5037557, "Echo width"=1.28, "Device ID "=120, "Layer"=2, "Echo"=0, "Reserved"=0, "Timestamp"=0, "flags"=0, "Reserved 2"=15}, {"X  position"=10.998041, "Y  position"=-2.5452418, "Z  position"=0.6158639, "Echo width"=1.7199999, "Device ID "=120, "Layer"=3, "Echo"=0, "Reserved"=0, "Timestamp"=0, "flags"=0, "Reserved 2"=15}, {"X  position"=10.79763, "Y  position"=-2.5484464, "Z  position"=0.50396514, "Echo width"=1.4399999, "Device ID "=120, "Layer"=2, "Echo"=0, "Reserved"=0, "Timestamp"=0, "flags"=16, "Reserved 2"=15}, {"X  position"=10.918911, "Y  position"=-2.5907998, "Z  position"=0.6146074, "Echo width"=1.3199999, "Device ID "=120, "Layer"=3, "Echo"=0, "Reserved"=0, "Timestamp"=0, "flags"=16, "Reserved 2"=15}, {"X  position"=10.944521, "Y  position"=-2.672856, "Z  position"=0.5052217, "Echo width"=1.8, "Device ID "=120, "Layer"=2, "Echo"=0, "Reserved"=0, "Timestamp"=0, "flags"=0, "Reserved 2"=15}, {"X  position"=11.065395, "Y  position"=-2.7162547, "Z  position"=0.61837703, "Echo width"=1.68, "Device ID "=120, "Layer"=3, "Echo"=0, "Reserved"=0, "Timestamp"=0, "flags"=0, "Reserved 2"=15}, {"X  position"=15.055982, "Y  position"=-4.263227, "Z  position"=0.70801055, "Echo width"=3.36, "Device ID "=120, "Layer"=3, "Echo"=0, "Reserved"=0, "Timestamp"=0, "flags"=16, "Reserved 2"=17}, {"X  position"=10.851264, "Y  position"=-2.748525, "Z  position"=0.28560197, "Echo width"=0.79999995, "Device ID "=120, "Layer"=0, "Echo"=0, "Reserved"=0, "Timestamp"=0, "flags"=4, "Reserved 2"=0}, {"X  position"=13.430894, "Y  position"=-3.7624793, "Z  position"=0.52414095, "Echo width"=1.5999999, "Device ID "=120, "Layer"=2, "Echo"=0, "Reserved"=0, "Timestamp"=0, "flags"=4100, "Reserved 2"=0}, {"X  position"=21.837553, "Y  position"=-6.9474773, "Z  position"=0.5869025, "Echo width"=0.91999996, "Device ID "=120, "Layer"=2, "Echo"=1, "Reserved"=0, "Timestamp"=0, "flags"=4096, "Reserved 2"=18}, {"X  position"=23.511404, "Y  position"=-7.581643, "Z  position"=0.599399, "Echo width"=0.64, "Device ID "=120, "Layer"=2, "Echo"=2, "Reserved"=0, "Timestamp"=0, "flags"=2, "Reserved 2"=19}, {"X  position"=14.644366, "Y  position"=-4.222223, "Z  position"=0.6996336, "Echo width"=4.16, "Device ID "=120, "Layer"=3, "Echo"=0, "Reserved"=0, "Timestamp"=0, "flags"=4, "Reserved 2"=0}, {"X  position"=12.779563, "Y  position"=-3.5620904, "Z  position"=0.38060626, "Echo width"=0.59999996, "Device ID "=120, "Layer"=1, "Echo"=0, "Reserved"=0, "Timestamp"=0, "flags"=20, "Reserved 2"=0}, {"X  position"=21.74827, "Y  position"=-7.096364, "Z  position"=0.58669305, "Echo width"=0.96, "Device ID "=120, "Layer"=2, "Echo"=0, "Reserved"=0, "Timestamp"=0, "flags"=0, "Reserved 2"=18}, {"X  position"=15.063681, "Y  position"=-4.4968696, "Z  position"=0.7098954, "Echo width"=4.36, "Device ID "=120, "Layer"=3, "Echo"=0, "Reserved"=0, "Timestamp"=0, "flags"=16, "Reserved 2"=17}, {"X  position"=12.4672575, "Y  position"=-3.532297, "Z  position"=0.24811508, "Echo width"=1.28, "Device ID "=120, "Layer"=0, "Echo"=0, "Reserved"=0, "Timestamp"=0, "flags"=0, "Reserved 2"=20}, {"X  position"=12.506222, "Y  position"=-3.5476456, "Z  position"=0.3824214, "Echo width"=1.3199999, "Device ID "=120, "Layer"=1, "Echo"=0, "Reserved"=0, "Timestamp"=0, "flags"=0, "Reserved 2"=20}, {"X  position"=12.537096, "Y  position"=-3.6054356, "Z  position"=0.51792765, "Echo width"=1.12, "Device ID "=120, "Layer"=2, "Echo"=0, "Reserved"=0, "Timestamp"=0, "flags"=4100, "Reserved 2"=0}, {"X  position"=17.719727, "Y  position"=-5.6730957, "Z  position"=0.5568831, "Echo width"=1.04, "Device ID "=120, "Layer"=2, "Echo"=1, "Reserved"=0, "Timestamp"=0, "flags"=0, "Reserved 2"=21}, {"X  position"=14.606126, "Y  position"=-4.430895, "Z  position"=0.70047134, "Echo width"=4.56, "Device ID "=120, "Layer"=3, "Echo"=0, "Reserved"=0, "Timestamp"=0, "flags"=0, "Reserved 2"=17}, {"X  position"=12.176537, "Y  position"=-3.5055482, "Z  position"=0.25397897, "Echo width"=1.0, "Device ID "=120, "Layer"=0, "Echo"=0, "Reserved"=0, "Timestamp"=0, "flags"=16, "Reserved 2"=20}, {"X  position"=12.24313, "Y  position"=-3.5324538, "Z  position"=0.38416672, "Echo width"=1.16, "Device ID "=120, "Layer"=1, "Echo"=0, "Reserved"=0, "Timestamp"=0, "flags"=16, "Reserved 2"=20}, {"X  position"=17.715954, "Y  position"=-5.815901, "Z  position"=0.55723214, "Echo width"=0.39999998, "Device ID "=120, "Layer"=2, "Echo"=0, "Reserved"=0, "Timestamp"=0, "flags"=0, "Reserved 2"=21}, {"X  position"=14.474503, "Y  position"=-4.489787, "Z  position"=0.6983771, "Echo width"=1.3199999, "Device ID "=120, "Layer"=3, "Echo"=0, "Reserved"=0, "Timestamp"=0, "flags"=4112, "Reserved 2"=17}, {"X  position"=16.232643, "Y  position"=-5.2090616, "Z  position"=0.73816764, "Echo width"=2.52, "Device ID "=120, "Layer"=3, "Echo"=1, "Reserved"=0, "Timestamp"=0, "flags"=16, "Reserved 2"=22}, {"X  position"=12.099431, "Y  position"=-3.5620015, "Z  position"=0.25502607, "Echo width"=1.5999999, "Device ID "=120, "Layer"=0, "Echo"=0, "Reserved"=0, "Timestamp"=0, "flags"=0, "Reserved 2"=20}, {"X  position"=11.981007, "Y  position"=-3.512948, "Z  position"=0.38591203, "Echo width"=1.64, "Device ID "=120, "Layer"=1, "Echo"=0, "Reserved"=0, "Timestamp"=0, "flags"=0, "Reserved 2"=20}, {"X  position"=11.937933, "Y  position"=-3.5383189, "Z  position"=0.5138785, "Echo width"=1.36, "Device ID "=120, "Layer"=2, "Echo"=0, "Reserved"=0, "Timestamp"=0, "flags"=0, "Reserved 2"=20}, {"X  position"=11.936288, "Y  position"=-3.5376294, "Z  position"=0.64162314, "Echo width"=1.52, "Device ID "=120, "Layer"=3, "Echo"=0, "Reserved"=0, "Timestamp"=0, "flags"=0, "Reserved 2"=20}, {"X  position"=11.745914, "Y  position"=-3.500183, "Z  position"=0.26235592, "Echo width"=1.24, "Device ID "=120, "Layer"=0, "Echo"=0, "Reserved"=0, "Timestamp"=0, "flags"=16, "Reserved 2"=20}, {"X  position"=11.848775, "Y  position"=-3.543845, "Z  position"=0.38667995, "Echo width"=1.24, "Device ID "=120, "Layer"=1, "Echo"=0, "Reserved"=0, "Timestamp"=0, "flags"=16, "Reserved 2"=20}, {"X  position"=11.759731, "Y  position"=-3.548661, "Z  position"=0.51276153, "Echo width"=1.16, "Device ID "=120, "Layer"=2, "Echo"=0, "Reserved"=0, "Timestamp"=0, "flags"=16, "Reserved 2"=20}, {"X  position"=11.693819, "Y  position"=-3.520343, "Z  position"=0.63680637, "Echo width"=1.0, "Device ID "=120, "Layer"=3, "Echo"=0, "Reserved"=0, "Timestamp"=0, "flags"=16, "Reserved 2"=20}, {"X  position"=11.605033, "Y  position"=-3.524169, "Z  position"=0.26486897, "Echo width"=1.68, "Device ID "=120, "Layer"=0, "Echo"=0, "Reserved"=0, "Timestamp"=0, "flags"=0, "Reserved 2"=20}, {"X  position"=11.606613, "Y  position"=-3.524856, "Z  position"=0.38828564, "Echo width"=1.4, "Device ID "=120, "Layer"=1, "Echo"=0, "Reserved"=0, "Timestamp"=0, "flags"=0, "Reserved 2"=20}, {"X  position"=11.545391, "Y  position"=-3.5400572, "Z  position"=0.5113653, "Echo width"=1.8, "Device ID "=120, "Layer"=2, "Echo"=0, "Reserved"=0, "Timestamp"=0, "flags"=0, "Reserved 2"=20}, {"X  position"=11.507219, "Y  position"=-3.5232608, "Z  position"=0.6332462, "Echo width"=1.52, "Device ID "=120, "Layer"=3, "Echo"=0, "Reserved"=0, "Timestamp"=0, "flags"=0, "Reserved 2"=20}, {"X  position"=11.436968, "Y  position"=-3.5337658, "Z  position"=0.26801038, "Echo width"=1.3199999, "Device ID "=120, "Layer"=0, "Echo"=0, "Reserved"=0, "Timestamp"=0, "flags"=16, "Reserved 2"=20}, {"X  position"=11.465921, "Y  position"=-3.546657, "Z  position"=0.3891234, "Echo width"=1.4399999, "Device ID "=120, "Layer"=1, "Echo"=0, "Reserved"=0, "Timestamp"=0, "flags"=16, "Reserved 2"=20}, {"X  position"=11.368315, "Y  position"=-3.5444171, "Z  position"=0.51024824, "Echo width"=1.24, "Device ID "=120, "Layer"=2, "Echo"=0, "Reserved"=0, "Timestamp"=0, "flags"=16, "Reserved 2"=20}, {"X  position"=11.394127, "Y  position"=-3.556045, "Z  position"=0.63136137, "Echo width"=1.3199999, "Device ID "=120, "Layer"=3, "Echo"=0, "Reserved"=0, "Timestamp"=0, "flags"=16, "Reserved 2"=20}, {"X  position"=11.305756, "Y  position"=-3.557288, "Z  position"=0.27031404, "Echo width"=1.52, "Device ID "=120, "Layer"=0, "Echo"=0, "Reserved"=0, "Timestamp"=0, "flags"=0, "Reserved 2"=20}, {"X  position"=11.325476, "Y  position"=-3.566275, "Z  position"=0.38996115, "Echo width"=1.36, "Device ID "=120, "Layer"=1, "Echo"=0, "Reserved"=0, "Timestamp"=0, "flags"=0, "Reserved 2"=20}, {"X  position"=11.391571, "Y  position"=-3.6380644, "Z  position"=0.51066715, "Echo width"=1.52, "Device ID "=120, "Layer"=2, "Echo"=0, "Reserved"=0, "Timestamp"=0, "flags"=0, "Reserved 2"=20}, {"X  position"=11.408192, "Y  position"=-3.6457267, "Z  position"=0.6324085, "Echo width"=1.52, "Device ID "=120, "Layer"=3, "Echo"=0, "Reserved"=0, "Timestamp"=0, "flags"=0, "Reserved 2"=20}, {"X  position"=11.201926, "Y  position"=-3.5914674, "Z  position"=0.2719894, "Echo width"=1.36, "Device ID "=120, "Layer"=0, "Echo"=0, "Reserved"=0, "Timestamp"=0, "flags"=16, "Reserved 2"=20}, {"X  position"=11.21249, "Y  position"=-3.5963938, "Z  position"=0.39058948, "Echo width"=1.36, "Device ID "=120, "Layer"=1, "Echo"=0, "Reserved"=0, "Timestamp"=0, "flags"=16, "Reserved 2"=20}, {"X  position"=11.241947, "Y  position"=-3.651339, "Z  position"=0.50975955, "Echo width"=0.39999998, "Device ID "=120, "Layer"=2, "Echo"=0, "Reserved"=0, "Timestamp"=0, "flags"=16, "Reserved 2"=20}, {"X  position"=14.314911, "Y  position"=-5.100643, "Z  position"=0.70047134, "Echo width"=0.96, "Device ID "=120, "Layer"=3, "Echo"=0, "Reserved"=0, "Timestamp"=0, "flags"=16, "Reserved 2"=23}, {"X  position"=11.188339, "Y  position"=-3.6671498, "Z  position"=0.27157056, "Echo width"=1.68, "Device ID "=120, "Layer"=0, "Echo"=0, "Reserved"=0, "Timestamp"=0, "flags"=0, "Reserved 2"=20}, {"X  position"=11.171788, "Y  position"=-3.6592555, "Z  position"=0.39065927, "Echo width"=1.64, "Device ID "=120, "Layer"=1, "Echo"=0, "Reserved"=0, "Timestamp"=0, "flags"=0, "Reserved 2"=20}, {"X  position"=11.200782, "Y  position"=-3.7144163, "Z  position"=0.50968975, "Echo width"=1.36, "Device ID "=120, "Layer"=2, "Echo"=0, "Reserved"=0, "Timestamp"=0, "flags"=0, "Reserved 2"=20}, {"X  position"=11.307341, "Y  position"=-3.7658143, "Z  position"=0.63157076, "Echo width"=1.12, "Device ID "=120, "Layer"=3, "Echo"=0, "Reserved"=0, "Timestamp"=0, "flags"=4100, "Reserved 2"=0}, {"X  position"=14.179937, "Y  position"=-5.1513906, "Z  position"=0.6983771, "Echo width"=1.4399999, "Device ID "=120, "Layer"=3, "Echo"=1, "Reserved"=0, "Timestamp"=0, "flags"=0, "Reserved 2"=23}, {"X  position"=11.218947, "Y  position"=-3.7647824, "Z  position"=0.2701046, "Echo width"=1.56, "Device ID "=120, "Layer"=0, "Echo"=0, "Reserved"=0, "Timestamp"=0, "flags"=16, "Reserved 2"=20}, {"X  position"=11.157537, "Y  position"=-3.734831, "Z  position"=0.39051965, "Echo width"=1.52, "Device ID "=120, "Layer"=1, "Echo"=0, "Reserved"=0, "Timestamp"=0, "flags"=16, "Reserved 2"=20}, {"X  position"=14.287012, "Y  position"=-5.3195662, "Z  position"=0.7019373, "Echo width"=0.79999995, "Device ID "=120, "Layer"=3, "Echo"=0, "Reserved"=0, "Timestamp"=0, "flags"=16, "Reserved 2"=23}, {"X  position"=11.051589, "Y  position"=-3.7650833, "Z  position"=0.273246, "Echo width"=1.68, "Device ID "=120, "Layer"=0, "Echo"=0, "Reserved"=0, "Timestamp"=0, "flags"=0, "Reserved 2"=20}, {"X  position"=11.070961, "Y  position"=-3.7747416, "Z  position"=0.39093852, "Echo width"=1.68, "Device ID "=120, "Layer"=1, "Echo"=0, "Reserved"=0, "Timestamp"=0, "flags"=0, "Reserved 2"=20}, {"X  position"=11.116924, "Y  position"=-3.839246, "Z  position"=0.50955015, "Echo width"=1.1999999, "Device ID "=120, "Layer"=2, "Echo"=0, "Reserved"=0, "Timestamp"=0, "flags"=4, "Reserved 2"=0}, {"X  position"=11.356491, "Y  position"=-3.9599977, "Z  position"=0.6342933, "Echo width"=1.24, "Device ID "=120, "Layer"=3, "Echo"=0, "Reserved"=0, "Timestamp"=0, "flags"=4100, "Reserved 2"=0}, {"X  position"=14.499087, "Y  position"=-5.5439963, "Z  position"=0.70801055, "Echo width"=1.8, "Device ID "=120, "Layer"=3, "Echo"=1, "Reserved"=0, "Timestamp"=0, "flags"=0, "Reserved 2"=23}, {"X  position"=10.973904, "Y  position"=-3.8081446, "Z  position"=0.2742931, "Echo width"=1.4399999, "Device ID "=120, "Layer"=0, "Echo"=0, "Reserved"=0, "Timestamp"=0, "flags"=16, "Reserved 2"=20}, {"X  position"=10.993182, "Y  position"=-3.8179672, "Z  position"=0.3912876, "Echo width"=1.5999999, "Device ID "=120, "Layer"=1, "Echo"=0, "Reserved"=0, "Timestamp"=0, "flags"=16, "Reserved 2"=20}, {"X  position"=14.325853, "Y  position"=-5.575681, "Z  position"=0.70507866, "Echo width"=1.36, "Device ID "=120, "Layer"=3, "Echo"=0, "Reserved"=0, "Timestamp"=0, "flags"=16, "Reserved 2"=23}, {"X  position"=10.904916, "Y  position"=-3.8547554, "Z  position"=0.2751308, "Echo width"=1.8399999, "Device ID "=120, "Layer"=0, "Echo"=0, "Reserved"=0, "Timestamp"=0, "flags"=0, "Reserved 2"=20}, {"X  position"=11.003929, "Y  position"=-3.9062984, "Z  position"=0.39093852, "Echo width"=1.76, "Device ID "=120, "Layer"=1, "Echo"=0, "Reserved"=0, "Timestamp"=0, "flags"=0, "Reserved 2"=20}, {"X  position"=11.084159, "Y  position"=-3.990219, "Z  position"=0.5098294, "Echo width"=1.24, "Device ID "=120, "Layer"=2, "Echo"=0, "Reserved"=0, "Timestamp"=0, "flags"=4, "Reserved 2"=0}, {"X  position"=11.374662, "Y  position"=-4.14306, "Z  position"=0.6363875, "Echo width"=1.0799999, "Device ID "=120, "Layer"=3, "Echo"=0, "Reserved"=0, "Timestamp"=0, "flags"=4100, "Reserved 2"=0}, {"X  position"=14.223698, "Y  position"=-5.64201, "Z  position"=0.70382214, "Echo width"=1.76, "Device ID "=120, "Layer"=3, "Echo"=1, "Reserved"=0, "Timestamp"=0, "flags"=0, "Reserved 2"=23}, {"X  position"=10.906304, "Y  position"=-3.938002, "Z  position"=0.2742931, "Echo width"=1.4399999, "Device ID "=120, "Layer"=0, "Echo"=0, "Reserved"=0, "Timestamp"=0, "flags"=16, "Reserved 2"=20}, {"X  position"=10.925407, "Y  position"=-3.9481597, "Z  position"=0.3912876, "Echo width"=1.5999999, "Device ID "=120, "Layer"=1, "Echo"=0, "Reserved"=0, "Timestamp"=0, "flags"=16, "Reserved 2"=20}, {"X  position"=14.341386, "Y  position"=-5.8252873, "Z  position"=0.70780116, "Echo width"=1.7199999, "Device ID "=120, "Layer"=3, "Echo"=0, "Reserved"=0, "Timestamp"=0, "flags"=16, "Reserved 2"=23}, {"X  position"=10.871657, "Y  position"=-4.002484, "Z  position"=0.2742931, "Echo width"=1.64, "Device ID "=120, "Layer"=0, "Echo"=0, "Reserved"=0, "Timestamp"=0, "flags"=0, "Reserved 2"=20}, {"X  position"=10.996126, "Y  position"=-4.070065, "Z  position"=0.39044985, "Echo width"=1.8399999, "Device ID "=120, "Layer"=1, "Echo"=0, "Reserved"=0, "Timestamp"=0, "flags"=0, "Reserved 2"=20}, {"X  position"=11.092269, "Y  position"=-4.1652613, "Z  position"=0.5104577, "Echo width"=1.3199999, "Device ID "=120, "Layer"=2, "Echo"=0, "Reserved"=0, "Timestamp"=0, "flags"=4, "Reserved 2"=0}, {"X  position"=11.344984, "Y  position"=-4.3039055, "Z  position"=0.63743466, "Echo width"=1.16, "Device ID "=120, "Layer"=3, "Echo"=0, "Reserved"=0, "Timestamp"=0, "flags"=4100, "Reserved 2"=0}, {"X  position"=14.053474, "Y  position"=-5.7898345, "Z  position"=0.7021467, "Echo width"=1.7199999, "Device ID "=120, "Layer"=3, "Echo"=1, "Reserved"=0, "Timestamp"=0, "flags"=0, "Reserved 2"=23}, {"X  position"=11.011335, "Y  position"=-4.163601, "Z  position"=0.2701046, "Echo width"=1.56, "Device ID "=120, "Layer"=0, "Echo"=0, "Reserved"=0, "Timestamp"=0, "flags"=16, "Reserved 2"=20}, {"X  position"=10.986562, "Y  position"=-4.1498685, "Z  position"=0.3902404, "Echo width"=1.56, "Device ID "=120, "Layer"=1, "Echo"=0, "Reserved"=0, "Timestamp"=0, "flags"=16, "Reserved 2"=20}, {"X  position"=10.974715, "Y  position"=-4.2289906, "Z  position"=0.2701046, "Echo width"=1.92, "Device ID "=120, "Layer"=0, "Echo"=0, "Reserved"=0, "Timestamp"=0, "flags"=0, "Reserved 2"=20}, {"X  position"=10.889139, "Y  position"=-4.180574, "Z  position"=0.3907291, "Echo width"=1.88, "Device ID "=120, "Layer"=1, "Echo"=0, "Reserved"=0, "Timestamp"=0, "flags"=0, "Reserved 2"=20}, {"X  position"=11.018419, "Y  position"=-4.2971306, "Z  position"=0.5104577, "Echo width"=1.3199999, "Device ID "=120, "Layer"=2, "Echo"=0, "Reserved"=0, "Timestamp"=0, "flags"=4, "Reserved 2"=0}, {"X  position"=11.372835, "Y  position"=-4.4996967, "Z  position"=0.6399477, "Echo width"=1.12, "Device ID "=120, "Layer"=3, "Echo"=0, "Reserved"=0, "Timestamp"=0, "flags"=4100, "Reserved 2"=0}, {"X  position"=14.358785, "Y  position"=-6.206307, "Z  position"=0.71198964, "Echo width"=1.64, "Device ID "=120, "Layer"=3, "Echo"=1, "Reserved"=0, "Timestamp"=0, "flags"=4, "Reserved 2"=0}, {"X  position"=10.902893, "Y  position"=-4.274062, "Z  position"=0.2709423, "Echo width"=1.7199999, "Device ID "=120, "Layer"=0, "Echo"=0, "Reserved"=0, "Timestamp"=0, "flags"=16, "Reserved 2"=20}, {"X  position"=10.826397, "Y  position"=-4.229897, "Z  position"=0.39093852, "Echo width"=1.76, "Device ID "=120, "Layer"=1, "Echo"=0, "Reserved"=0, "Timestamp"=0, "flags"=16, "Reserved 2"=20}, {"X  position"=10.934229, "Y  position"=-4.3790956, "Z  position"=0.2692669, "Echo width"=1.9599999, "Device ID "=120, "Layer"=0, "Echo"=0, "Reserved"=0, "Timestamp"=0, "flags"=0, "Reserved 2"=20}, {"X  position"=10.875364, "Y  position"=-4.3444223, "Z  position"=0.3902404, "Echo width"=1.92, "Device ID "=120, "Layer"=1, "Echo"=0, "Reserved"=0, "Timestamp"=0, "flags"=0, "Reserved 2"=20}, {"X  position"=11.079781, "Y  position"=-4.5094953, "Z  position"=0.5115747, "Echo width"=1.28, "Device ID "=120, "Layer"=2, "Echo"=0, "Reserved"=0, "Timestamp"=0, "flags"=0, "Reserved 2"=20}, {"X  position"=11.310291, "Y  position"=-4.646635, "Z  position"=0.64036655, "Echo width"=1.28, "Device ID "=120, "Layer"=3, "Echo"=0, "Reserved"=0, "Timestamp"=0, "flags"=4100, "Reserved 2"=0}, {"X  position"=14.532358, "Y  position"=-6.563564, "Z  position"=0.7189007, "Echo width"=2.0, "Device ID "=120, "Layer"=3, "Echo"=1, "Reserved"=0, "Timestamp"=0, "flags"=4, "Reserved 2"=0}, {"X  position"=10.895731, "Y  position"=-4.4438043, "Z  position"=0.2692669, "Echo width"=1.64, "Device ID "=120, "Layer"=0, "Echo"=0, "Reserved"=0, "Timestamp"=0, "flags"=16, "Reserved 2"=20}, {"X  position"=10.854317, "Y  position"=-4.4189196, "Z  position"=0.39010078, "Echo width"=1.8, "Device ID "=120, "Layer"=1, "Echo"=0, "Reserved"=0, "Timestamp"=0, "flags"=16, "Reserved 2"=20}, {"X  position"=11.099981, "Y  position"=-4.6117816, "Z  position"=0.5120634, "Echo width"=0.64, "Device ID "=120, "Layer"=2, "Echo"=0, "Reserved"=0, "Timestamp"=0, "flags"=16, "Reserved 2"=20}, {"X  position"=11.8079195, "Y  position"=-5.0413694, "Z  position"=0.6535603, "Echo width"=1.0, "Device ID "=120, "Layer"=3, "Echo"=0, "Reserved"=0, "Timestamp"=0, "flags"=16, "Reserved 2"=24}, {"X  position"=10.958965, "Y  position"=-4.57086, "Z  position"=0.26675382, "Echo width"=1.88, "Device ID "=120, "Layer"=0, "Echo"=0, "Reserved"=0, "Timestamp"=0, "flags"=0, "Reserved 2"=20}, {"X  position"=10.841053, "Y  position"=-4.498603, "Z  position"=0.38989133, "Echo width"=1.8399999, "Device ID "=120, "Layer"=1, "Echo"=0, "Reserved"=0, "Timestamp"=0, "flags"=0, "Reserved 2"=20}, {"X  position"=11.076453, "Y  position"=-4.688452, "Z  position"=0.51220304, "Echo width"=1.36, "Device ID "=120, "Layer"=2, "Echo"=0, "Reserved"=0, "Timestamp"=0, "flags"=0, "Reserved 2"=20}, {"X  position"=11.695597, "Y  position"=-5.0715895, "Z  position"=0.6518849, "Echo width"=1.76, "Device ID "=120, "Layer"=3, "Echo"=0, "Reserved"=0, "Timestamp"=0, "flags"=0, "Reserved 2"=24}, {"X  position"=10.884879, "Y  position"=-4.6145844, "Z  position"=0.2675915, "Echo width"=1.48, "Device ID "=120, "Layer"=0, "Echo"=0, "Reserved"=0, "Timestamp"=0, "flags"=16, "Reserved 2"=20}, {"X  position"=10.843918, "Y  position"=-4.5889893, "Z  position"=0.38954228, "Echo width"=1.8, "Device ID "=120, "Layer"=1, "Echo"=0, "Reserved"=0, "Timestamp"=0, "flags"=16, "Reserved 2"=20}, {"X  position"=11.00988, "Y  position"=-4.7383814, "Z  position"=0.5119936, "Echo width"=0.76, "Device ID "=120, "Layer"=2, "Echo"=0, "Reserved"=0, "Timestamp"=0, "flags"=16, "Reserved 2"=20}, {"X  position"=11.769403, "Y  position"=-5.217605, "Z  position"=0.65481687, "Echo width"=1.28, "Device ID "=120, "Layer"=3, "Echo"=0, "Reserved"=0, "Timestamp"=0, "flags"=16, "Reserved 2"=24}, {"X  position"=10.93708, "Y  position"=-4.7379427, "Z  position"=0.26528785, "Echo width"=1.52, "Device ID "=120, "Layer"=0, "Echo"=0, "Reserved"=0, "Timestamp"=0, "flags"=0, "Reserved 2"=20}, {"X  position"=10.896362, "Y  position"=-4.7120028, "Z  position"=0.38877434, "Echo width"=1.8399999, "Device ID "=120, "Layer"=1, "Echo"=0, "Reserved"=0, "Timestamp"=0, "flags"=0, "Reserved 2"=20}, {"X  position"=11.052345, "Y  position"=-4.857832, "Z  position"=0.5126917, "Echo width"=1.3199999, "Device ID "=120, "Layer"=2, "Echo"=0, "Reserved"=0, "Timestamp"=0, "flags"=0, "Reserved 2"=20}, {"X  position"=11.462893, "Y  position"=-5.1219044, "Z  position"=0.64832467, "Echo width"=1.52, "Device ID "=120, "Layer"=3, "Echo"=0, "Reserved"=0, "Timestamp"=0, "flags"=0, "Reserved 2"=24}, {"X  position"=10.912222, "Y  position"=-4.8135533, "Z  position"=0.26486897, "Echo width"=0.96, "Device ID "=120, "Layer"=0, "Echo"=0, "Reserved"=0, "Timestamp"=0, "flags"=16, "Reserved 2"=20}, {"X  position"=10.938826, "Y  position"=-4.8308306, "Z  position"=0.38807622, "Echo width"=1.12, "Device ID "=120, "Layer"=1, "Echo"=0, "Reserved"=0, "Timestamp"=0, "flags"=16, "Reserved 2"=20}, {"X  position"=11.401171, "Y  position"=-5.180235, "Z  position"=0.6479058, "Echo width"=1.12, "Device ID "=120, "Layer"=3, "Echo"=0, "Reserved"=0, "Timestamp"=0, "flags"=16, "Reserved 2"=24}, {"X  position"=10.936629, "Y  position"=-4.922198, "Z  position"=0.2631936, "Echo width"=1.28, "Device ID "=120, "Layer"=0, "Echo"=0, "Reserved"=0, "Timestamp"=0, "flags"=0, "Reserved 2"=20}, {"X  position"=10.971435, "Y  position"=-4.945235, "Z  position"=0.3874479, "Echo width"=1.28, "Device ID "=120, "Layer"=1, "Echo"=0, "Reserved"=0, "Timestamp"=0, "flags"=0, "Reserved 2"=20}, {"X  position"=11.199221, "Y  position"=-5.144455, "Z  position"=0.5146465, "Echo width"=1.3199999, "Device ID "=120, "Layer"=2, "Echo"=0, "Reserved"=0, "Timestamp"=0, "flags"=4, "Reserved 2"=0}, {"X  position"=11.397228, "Y  position"=-5.2767596, "Z  position"=0.64895296, "Echo width"=1.48, "Device ID "=120, "Layer"=3, "Echo"=0, "Reserved"=0, "Timestamp"=0, "flags"=4096, "Reserved 2"=24}, {"X  position"=13.616766, "Y  position"=-6.759807, "Z  position"=0.7048693, "Echo width"=0.32, "Device ID "=120, "Layer"=3, "Echo"=1, "Reserved"=0, "Timestamp"=0, "flags"=4100, "Reserved 2"=0}, {"X  position"=14.639249, "Y  position"=-7.443008, "Z  position"=0.7306284, "Echo width"=1.1999999, "Device ID "=120, "Layer"=3, "Echo"=2, "Reserved"=0, "Timestamp"=0, "flags"=0, "Reserved 2"=25}, {"X  position"=12.220309, "Y  position"=-5.937447, "Z  position"=0.5236523, "Echo width"=1.24, "Device ID "=120, "Layer"=2, "Echo"=0, "Reserved"=0, "Timestamp"=0, "flags"=16, "Reserved 2"=26}, {"X  position"=12.375627, "Y  position"=-6.043199, "Z  position"=0.6749216, "Echo width"=0.76, "Device ID "=120, "Layer"=3, "Echo"=0, "Reserved"=0, "Timestamp"=0, "flags"=4112, "Reserved 2"=26}, {"X  position"=14.325951, "Y  position"=-7.371127, "Z  position"=0.7243457, "Echo width"=1.48, "Device ID "=120, "Layer"=3, "Echo"=1, "Reserved"=0, "Timestamp"=0, "flags"=16, "Reserved 2"=25}, {"X  position"=12.052554, "Y  position"=-5.8780074, "Z  position"=0.23261766, "Echo width"=1.56, "Device ID "=120, "Layer"=0, "Echo"=0, "Reserved"=0, "Timestamp"=0, "flags"=0, "Reserved 2"=26}, {"X  position"=12.177837, "Y  position"=-5.9641123, "Z  position"=0.3764873, "Echo width"=1.52, "Device ID "=120, "Layer"=1, "Echo"=0, "Reserved"=0, "Timestamp"=0, "flags"=0, "Reserved 2"=26}, {"X  position"=12.061353, "Y  position"=-5.939222, "Z  position"=0.5227447, "Echo width"=1.7199999, "Device ID "=120, "Layer"=2, "Echo"=0, "Reserved"=0, "Timestamp"=0, "flags"=0, "Reserved 2"=26}, {"X  position"=12.067897, "Y  position"=-5.943762, "Z  position"=0.66842943, "Echo width"=1.5999999, "Device ID "=120, "Layer"=3, "Echo"=0, "Reserved"=0, "Timestamp"=0, "flags"=0, "Reserved 2"=26}, {"X  position"=11.9927435, "Y  position"=-5.946683, "Z  position"=0.2328271, "Echo width"=1.28, "Device ID "=120, "Layer"=0, "Echo"=0, "Reserved"=0, "Timestamp"=0, "flags"=16, "Reserved 2"=26}, {"X  position"=11.978016, "Y  position"=-5.936371, "Z  position"=0.37774396, "Echo width"=1.36, "Device ID "=120, "Layer"=1, "Echo"=0, "Reserved"=0, "Timestamp"=0, "flags"=16, "Reserved 2"=26}, {"X  position"=11.878538, "Y  position"=-5.9213657, "Z  position"=0.5216277, "Echo width"=1.56, "Device ID "=120, "Layer"=2, "Echo"=0, "Reserved"=0, "Timestamp"=0, "flags"=16, "Reserved 2"=26}, {"X  position"=11.909563, "Y  position"=-5.943292, "Z  position"=0.66570693, "Echo width"=1.4399999, "Device ID "=120, "Layer"=3, "Echo"=0, "Reserved"=0, "Timestamp"=0, "flags"=16, "Reserved 2"=26}, {"X  position"=11.956804, "Y  position"=-6.03218, "Z  position"=0.23240826, "Echo width"=1.9599999, "Device ID "=120, "Layer"=0, "Echo"=0, "Reserved"=0, "Timestamp"=0, "flags"=0, "Reserved 2"=26}, {"X  position"=11.820058, "Y  position"=-5.9346395, "Z  position"=0.3786515, "Echo width"=1.68, "Device ID "=120, "Layer"=1, "Echo"=0, "Reserved"=0, "Timestamp"=0, "flags"=0, "Reserved 2"=26}, {"X  position"=11.729159, "Y  position"=-5.924147, "Z  position"=0.52079, "Echo width"=1.7199999, "Device ID "=120, "Layer"=2, "Echo"=0, "Reserved"=0, "Timestamp"=0, "flags"=0, "Reserved 2"=26}, {"X  position"=11.743783, "Y  position"=-5.9346743, "Z  position"=0.662775, "Echo width"=1.76, "Device ID "=120, "Layer"=3, "Echo"=0, "Reserved"=0, "Timestamp"=0, "flags"=0, "Reserved 2"=26}, {"X  position"=11.645014, "Y  position"=-5.917699, "Z  position"=0.23910983, "Echo width"=1.4399999, "Device ID "=120, "Layer"=0, "Echo"=0, "Reserved"=0, "Timestamp"=0, "flags"=16, "Reserved 2"=26}, {"X  position"=11.646603, "Y  position"=-5.9188533, "Z  position"=0.3796987, "Echo width"=1.24, "Device ID "=120, "Layer"=1, "Echo"=0, "Reserved"=0, "Timestamp"=0, "flags"=16, "Reserved 2"=26}, {"X  position"=11.588442, "Y  position"=-5.9306912, "Z  position"=0.52002203, "Echo width"=1.12, "Device ID "=120, "Layer"=2, "Echo"=0, "Reserved"=0, "Timestamp"=0, "flags"=16, "Reserved 2"=26}, {"X  position"=11.57074, "Y  position"=-5.9177117, "Z  position"=0.65963364, "Echo width"=1.16, "Device ID "=120, "Layer"=3, "Echo"=0, "Reserved"=0, "Timestamp"=0, "flags"=16, "Reserved 2"=26}, {"X  position"=11.536805, "Y  position"=-5.9469237, "Z  position"=0.24057579, "Echo width"=1.7199999, "Device ID "=120, "Layer"=0, "Echo"=0, "Reserved"=0, "Timestamp"=0, "flags"=0, "Reserved 2"=26}, {"X  position"=11.522296, "Y  position"=-5.936187, "Z  position"=0.38032702, "Echo width"=1.68, "Device ID "=120, "Layer"=1, "Echo"=0, "Reserved"=0, "Timestamp"=0, "flags"=0, "Reserved 2"=26}, {"X  position"=11.464268, "Y  position"=-5.9472013, "Z  position"=0.5193937, "Echo width"=1.68, "Device ID "=120, "Layer"=2, "Echo"=0, "Reserved"=0, "Timestamp"=0, "flags"=0, "Reserved 2"=26}, {"X  position"=11.534813, "Y  position"=-5.9998794, "Z  position"=0.6600524, "Echo width"=1.52, "Device ID "=120, "Layer"=3, "Echo"=0, "Reserved"=0, "Timestamp"=0, "flags"=0, "Reserved 2"=26}, {"X  position"=11.436695, "Y  position"=-5.980729, "Z  position"=0.24183235, "Echo width"=1.4, "Device ID "=120, "Layer"=0, "Echo"=0, "Reserved"=0, "Timestamp"=0, "flags"=16, "Reserved 2"=26}, {"X  position"=11.422271, "Y  position"=-5.9698596, "Z  position"=0.3807459, "Echo width"=1.48, "Device ID "=120, "Layer"=1, "Echo"=0, "Reserved"=0, "Timestamp"=0, "flags"=16, "Reserved 2"=26}, {"X  position"=11.364307, "Y  position"=-5.980159, "Z  position"=0.51897484, "Echo width"=1.36, "Device ID "=120, "Layer"=2, "Echo"=0, "Reserved"=0, "Timestamp"=0, "flags"=16, "Reserved 2"=26}, {"X  position"=11.402565, "Y  position"=-6.0092506, "Z  position"=0.6579582, "Echo width"=1.1999999, "Device ID "=120, "Layer"=3, "Echo"=0, "Reserved"=0, "Timestamp"=0, "flags"=4112, "Reserved 2"=26}, {"X  position"=14.410793, "Y  position"=-8.296761, "Z  position"=0.73712057, "Echo width"=0.35999998, "Device ID "=120, "Layer"=3, "Echo"=1, "Reserved"=0, "Timestamp"=0, "flags"=16, "Reserved 2"=27}, {"X  position"=11.400066, "Y  position"=-6.061934, "Z  position"=0.24141349, "Echo width"=1.8, "Device ID "=120, "Layer"=0, "Echo"=0, "Reserved"=0, "Timestamp"=0, "flags"=0, "Reserved 2"=26}, {"X  position"=11.322273, "Y  position"=-6.002241, "Z  position"=0.38116476, "Echo width"=1.68, "Device ID "=120, "Layer"=1, "Echo"=0, "Reserved"=0, "Timestamp"=0, "flags"=0, "Reserved 2"=26}, {"X  position"=11.272289, "Y  position"=-6.0179496, "Z  position"=0.5186258, "Echo width"=1.76, "Device ID "=120, "Layer"=2, "Echo"=0, "Reserved"=0, "Timestamp"=0, "flags"=0, "Reserved 2"=26}, {"X  position"=11.3103, "Y  position"=-6.0473804, "Z  position"=0.65691113, "Echo width"=1.68, "Device ID "=120, "Layer"=3, "Echo"=0, "Reserved"=0, "Timestamp"=0, "flags"=4096, "Reserved 2"=26}, {"X  position"=13.8794775, "Y  position"=-8.03665, "Z  position"=0.724974, "Echo width"=1.3199999, "Device ID "=120, "Layer"=3, "Echo"=1, "Reserved"=0, "Timestamp"=0, "flags"=4, "Reserved 2"=0}, {"X  position"=11.268082, "Y  position"=-6.0690904, "Z  position"=0.24350774, "Echo width"=1.36, "Device ID "=120, "Layer"=0, "Echo"=0, "Reserved"=0, "Timestamp"=0, "flags"=16, "Reserved 2"=26}, {"X  position"=11.206557, "Y  position"=-6.0210223, "Z  position"=0.38172325, "Echo width"=1.8, "Device ID "=120, "Layer"=1, "Echo"=0, "Reserved"=0, "Timestamp"=0, "flags"=16, "Reserved 2"=26}, {"X  position"=11.156652, "Y  position"=-6.036019, "Z  position"=0.5180673, "Echo width"=1.64, "Device ID "=120, "Layer"=2, "Echo"=0, "Reserved"=0, "Timestamp"=0, "flags"=16, "Reserved 2"=26}, {"X  position"=11.210119, "Y  position"=-6.078169, "Z  position"=0.65565455, "Echo width"=1.56, "Device ID "=120, "Layer"=3, "Echo"=0, "Reserved"=0, "Timestamp"=0, "flags"=16, "Reserved 2"=26}, {"X  position"=11.308716, "Y  position"=-6.2113338, "Z  position"=0.24099465, "Echo width"=1.52, "Device ID "=120, "Layer"=0, "Echo"=0, "Reserved"=0, "Timestamp"=0, "flags"=0, "Reserved 2"=26}, {"X  position"=11.169373, "Y  position"=-6.100495, "Z  position"=0.38158363, "Echo width"=1.92, "Device ID "=120, "Layer"=1, "Echo"=0, "Reserved"=0, "Timestamp"=0, "flags"=0, "Reserved 2"=26}, {"X  position"=11.166078, "Y  position"=-6.1526785, "Z  position"=0.5186258, "Echo width"=1.76, "Device ID "=120, "Layer"=2, "Echo"=0, "Reserved"=0, "Timestamp"=0, "flags"=0, "Reserved 2"=26}, {"X  position"=11.17238, "Y  position"=-6.157737, "Z  position"=0.6560734, "Echo width"=1.8, "Device ID "=120, "Layer"=3, "Echo"=0, "Reserved"=0, "Timestamp"=0, "flags"=0, "Reserved 2"=26}, {"X  position"=11.300834, "Y  position"=-6.316991, "Z  position"=0.23973809, "Echo width"=0.91999996, "Device ID "=120, "Layer"=0, "Echo"=0, "Reserved"=0, "Timestamp"=0, "flags"=16, "Reserved 2"=26}, {"X  position"=11.123615, "Y  position"=-6.173482, "Z  position"=0.38151383, "Echo width"=1.64, "Device ID "=120, "Layer"=1, "Echo"=0, "Reserved"=0, "Timestamp"=0, "flags"=16, "Reserved 2"=26}, {"X  position"=11.096606, "Y  position"=-6.2066875, "Z  position"=0.51848614, "Echo width"=1.76, "Device ID "=120, "Layer"=2, "Echo"=0, "Reserved"=0, "Timestamp"=0, "flags"=16, "Reserved 2"=26}, {"X  position"=11.102867, "Y  position"=-6.211803, "Z  position"=0.65565455, "Echo width"=1.48, "Device ID "=120, "Layer"=3, "Echo"=0, "Reserved"=0, "Timestamp"=0, "flags"=16, "Reserved 2"=26}, {"X  position"=11.152836, "Y  position"=-6.3085117, "Z  position"=0.24225119, "Echo width"=1.8, "Device ID "=120, "Layer"=0, "Echo"=0, "Reserved"=0, "Timestamp"=0, "flags"=0, "Reserved 2"=26}, {"X  position"=11.108032, "Y  position"=-6.2715783, "Z  position"=0.38116476, "Echo width"=1.8, "Device ID "=120, "Layer"=1, "Echo"=0, "Reserved"=0, "Timestamp"=0, "flags"=0, "Reserved 2"=26}, {"X  position"=11.088284, "Y  position"=-6.311109, "Z  position"=0.51890504, "Echo width"=1.8, "Device ID "=120, "Layer"=2, "Echo"=0, "Reserved"=0, "Timestamp"=0, "flags"=0, "Reserved 2"=26}, {"X  position"=11.317406, "Y  position"=-6.501668, "Z  position"=0.6629844, "Echo width"=1.4, "Device ID "=120, "Layer"=3, "Echo"=0, "Reserved"=0, "Timestamp"=0, "flags"=4096, "Reserved 2"=26}, {"X  position"=13.984701, "Y  position"=-8.720035, "Z  position"=0.7356546, "Echo width"=1.1999999, "Device ID "=120, "Layer"=3, "Echo"=1, "Reserved"=0, "Timestamp"=0, "flags"=0, "Reserved 2"=28}, {"X  position"=11.112812, "Y  position"=-6.3879075, "Z  position"=0.24183235, "Echo width"=1.4, "Device ID "=120, "Layer"=0, "Echo"=0, "Reserved"=0, "Timestamp"=0, "flags"=16, "Reserved 2"=26}, {"X  position"=11.0759945, "Y  position"=-6.357014, "Z  position"=0.38095534, "Echo width"=1.64, "Device ID "=120, "Layer"=1, "Echo"=0, "Reserved"=0, "Timestamp"=0, "flags"=16, "Reserved 2"=26}, {"X  position"=11.185564, "Y  position"=-6.50631, "Z  position"=0.5203013, "Echo width"=1.28, "Device ID "=120, "Layer"=2, "Echo"=0, "Reserved"=0, "Timestamp"=0, "flags"=16, "Reserved 2"=26}, {"X  position"=13.999775, "Y  position"=-8.888716, "Z  position"=0.73816764, "Echo width"=0.48, "Device ID "=120, "Layer"=3, "Echo"=0, "Reserved"=0, "Timestamp"=0, "flags"=16, "Reserved 2"=28}, {"X  position"=11.216428, "Y  position"=-6.590452, "Z  position"=0.23743443, "Echo width"=1.5999999, "Device ID "=120, "Layer"=0, "Echo"=0, "Reserved"=0, "Timestamp"=0, "flags"=0, "Reserved 2"=26}, {"X  position"=11.05825, "Y  position"=-6.4553566, "Z  position"=0.38060626, "Echo width"=1.7199999, "Device ID "=120, "Layer"=1, "Echo"=0, "Reserved"=0, "Timestamp"=0, "flags"=0, "Reserved 2"=26}, {"X  position"=11.151219, "Y  position"=-6.592713, "Z  position"=0.52051073, "Echo width"=1.64, "Device ID "=120, "Layer"=2, "Echo"=0, "Reserved"=0, "Timestamp"=0, "flags"=0, "Reserved 2"=26}, {"X  position"=11.505705, "Y  position"=-6.8981576, "Z  position"=0.6713613, "Echo width"=1.8399999, "Device ID "=120, "Layer"=3, "Echo"=0, "Reserved"=0, "Timestamp"=0, "flags"=4, "Reserved 2"=0}, {"X  position"=11.135985, "Y  position"=-6.637861, "Z  position"=0.23806271, "Echo width"=1.0, "Device ID "=120, "Layer"=0, "Echo"=0, "Reserved"=0, "Timestamp"=0, "flags"=16, "Reserved 2"=26}, {"X  position"=10.994083, "Y  position"=-6.514507, "Z  position"=0.3806761, "Echo width"=1.64, "Device ID "=120, "Layer"=1, "Echo"=0, "Reserved"=0, "Timestamp"=0, "flags"=16, "Reserved 2"=26}, {"X  position"=11.070842, "Y  position"=-6.639451, "Z  position"=0.5203013, "Echo width"=1.1999999, "Device ID "=120, "Layer"=2, "Echo"=0, "Reserved"=0, "Timestamp"=0, "flags"=16, "Reserved 2"=26}, {"X  position"=11.077769, "Y  position"=-6.7042437, "Z  position"=0.23806271, "Echo width"=1.3199999, "Device ID "=120, "Layer"=0, "Echo"=0, "Reserved"=0, "Timestamp"=0, "flags"=0, "Reserved 2"=26}, {"X  position"=10.996864, "Y  position"=-6.632665, "Z  position"=0.38011757, "Echo width"=1.88, "Device ID "=120, "Layer"=1, "Echo"=0, "Reserved"=0, "Timestamp"=0, "flags"=0, "Reserved 2"=26}, {"X  position"=11.094678, "Y  position"=-6.77851, "Z  position"=0.5210692, "Echo width"=1.68, "Device ID "=120, "Layer"=2, "Echo"=0, "Reserved"=0, "Timestamp"=0, "flags"=0, "Reserved 2"=26}, {"X  position"=11.540734, "Y  position"=-7.17663, "Z  position"=0.67575926, "Echo width"=2.12, "Device ID "=120, "Layer"=3, "Echo"=0, "Reserved"=0, "Timestamp"=0, "flags"=0, "Reserved 2"=26}, {"X  position"=11.167572, "Y  position"=-6.903913, "Z  position"=0.23387422, "Echo width"=1.1999999, "Device ID "=120, "Layer"=0, "Echo"=0, "Reserved"=0, "Timestamp"=0, "flags"=16, "Reserved 2"=26}, {"X  position"=10.990717, "Y  position"=-6.744672, "Z  position"=0.3796289, "Echo width"=1.68, "Device ID "=120, "Layer"=1, "Echo"=0, "Reserved"=0, "Timestamp"=0, "flags"=16, "Reserved 2"=26}, {"X  position"=11.109257, "Y  position"=-6.9117618, "Z  position"=0.5217673, "Echo width"=1.4, "Device ID "=120, "Layer"=2, "Echo"=0, "Reserved"=0, "Timestamp"=0, "flags"=16, "Reserved 2"=26}, {"X  position"=11.507402, "Y  position"=-7.2734127, "Z  position"=0.676597, "Echo width"=0.76, "Device ID "=120, "Layer"=3, "Echo"=0, "Reserved"=0, "Timestamp"=0, "flags"=16, "Reserved 2"=26}, {"X  position"=11.180744, "Y  position"=-7.038106, "Z  position"=0.23177998, "Echo width"=1.52, "Device ID "=120, "Layer"=0, "Echo"=0, "Reserved"=0, "Timestamp"=0, "flags"=0, "Reserved 2"=26}, {"X  position"=11.0053005, "Y  position"=-6.8773403, "Z  position"=0.37893075, "Echo width"=1.76, "Device ID "=120, "Layer"=1, "Echo"=0, "Reserved"=0, "Timestamp"=0, "flags"=0, "Reserved 2"=26}, {"X  position"=11.026622, "Y  position"=-6.957538, "Z  position"=0.5215579, "Echo width"=1.56, "Device ID "=120, "Layer"=2, "Echo"=0, "Reserved"=0, "Timestamp"=0, "flags"=0, "Reserved 2"=26}, {"X  position"=11.480335, "Y  position"=-7.376946, "Z  position"=0.6776441, "Echo width"=1.52, "Device ID "=120, "Layer"=3, "Echo"=0, "Reserved"=0, "Timestamp"=0, "flags"=0, "Reserved 2"=26}, {"X  position"=11.133657, "Y  position"=-7.118501, "Z  position"=0.23136114, "Echo width"=1.12, "Device ID "=120, "Layer"=0, "Echo"=0, "Reserved"=0, "Timestamp"=0, "flags"=16, "Reserved 2"=26}, {"X  position"=11.018132, "Y  position"=-7.010772, "Z  position"=0.37823263, "Echo width"=1.56, "Device ID "=120, "Layer"=1, "Echo"=0, "Reserved"=0, "Timestamp"=0, "flags"=16, "Reserved 2"=26}, {"X  position"=11.089441, "Y  position"=-7.139433, "Z  position"=0.5227447, "Echo width"=0.88, "Device ID "=120, "Layer"=2, "Echo"=0, "Reserved"=0, "Timestamp"=0, "flags"=16, "Reserved 2"=26}, {"X  position"=14.306654, "Y  position"=-10.165885, "Z  position"=0.76078546, "Echo width"=2.04, "Device ID "=120, "Layer"=3, "Echo"=0, "Reserved"=0, "Timestamp"=0, "flags"=0, "Reserved 2"=29}, {"X  position"=11.303316, "Y  position"=-7.4050703, "Z  position"=0.22465955, "Echo width"=1.4, "Device ID "=120, "Layer"=0, "Echo"=0, "Reserved"=0, "Timestamp"=0, "flags"=0, "Reserved 2"=26}, {"X  position"=11.108992, "Y  position"=-7.220663, "Z  position"=0.37676656, "Echo width"=1.4399999, "Device ID "=120, "Layer"=1, "Echo"=0, "Reserved"=0, "Timestamp"=0, "flags"=0, "Reserved 2"=26}, {"X  position"=11.120754, "Y  position"=-7.2952847, "Z  position"=0.5236523, "Echo width"=1.36, "Device ID "=120, "Layer"=2, "Echo"=0, "Reserved"=0, "Timestamp"=0, "flags"=0, "Reserved 2"=26}, {"X  position"=11.133712, "Y  position"=-7.3076897, "Z  position"=0.6713613, "Echo width"=1.36, "Device ID "=120, "Layer"=3, "Echo"=0, "Reserved"=0, "Timestamp"=0, "flags"=4100, "Reserved 2"=0}, {"X  position"=14.506412, "Y  position"=-10.536347, "Z  position"=0.7691624, "Echo width"=2.1599998, "Device ID "=120, "Layer"=3, "Echo"=1, "Reserved"=0, "Timestamp"=0, "flags"=0, "Reserved 2"=29}, {"X  position"=12.1445675, "Y  position"=-8.347961, "Z  position"=0.19827211, "Echo width"=1.4, "Device ID "=120, "Layer"=0, "Echo"=0, "Reserved"=0, "Timestamp"=0, "flags"=16, "Reserved 2"=30}, {"X  position"=12.225379, "Y  position"=-8.426002, "Z  position"=0.36531729, "Echo width"=0.79999995, "Device ID "=120, "Layer"=1, "Echo"=0, "Reserved"=0, "Timestamp"=0, "flags"=16, "Reserved 2"=30}, {"X  position"=12.088251, "Y  position"=-8.366304, "Z  position"=0.5337053, "Echo width"=1.16, "Device ID "=120, "Layer"=2, "Echo"=0, "Reserved"=0, "Timestamp"=0, "flags"=16, "Reserved 2"=30}, {"X  position"=14.2564945, "Y  position"=-10.478514, "Z  position"=0.7645551, "Echo width"=2.12, "Device ID "=120, "Layer"=3, "Echo"=0, "Reserved"=0, "Timestamp"=0, "flags"=0, "Reserved 2"=29}, {"X  position"=12.114176, "Y  position"=-8.465127, "Z  position"=0.19701555, "Echo width"=1.4, "Device ID "=120, "Layer"=0, "Echo"=0, "Reserved"=0, "Timestamp"=0, "flags"=0, "Reserved 2"=30}, {"X  position"=12.037399, "Y  position"=-8.389679, "Z  position"=0.3664343, "Echo width"=1.4399999, "Device ID "=120, "Layer"=1, "Echo"=0, "Reserved"=0, "Timestamp"=0, "flags"=0, "Reserved 2"=30}, {"X  position"=12.0149145, "Y  position"=-8.440931, "Z  position"=0.5337053, "Echo width"=1.76, "Device ID "=120, "Layer"=2, "Echo"=0, "Reserved"=0, "Timestamp"=0, "flags"=0, "Reserved 2"=30}, {"X  position"=11.984854, "Y  position"=-8.411132, "Z  position"=0.7002619, "Echo width"=1.5999999, "Device ID "=120, "Layer"=3, "Echo"=0, "Reserved"=0, "Timestamp"=0, "flags"=0, "Reserved 2"=30}, {"X  position"=11.98342, "Y  position"=-8.48342, "Z  position"=0.19869095, "Echo width"=0.96, "Device ID "=120, "Layer"=0, "Echo"=0, "Reserved"=0, "Timestamp"=0, "flags"=16, "Reserved 2"=30}, {"X  position"=11.985074, "Y  position"=-8.485074, "Z  position"=0.36622488, "Echo width"=1.4399999, "Device ID "=120, "Layer"=1, "Echo"=0, "Reserved"=0, "Timestamp"=0, "flags"=16, "Reserved 2"=30}, {"X  position"=11.842371, "Y  position"=-8.415491, "Z  position"=0.5327279, "Echo width"=1.68, "Device ID "=120, "Layer"=2, "Echo"=0, "Reserved"=0, "Timestamp"=0, "flags"=16, "Reserved 2"=30}, {"X  position"=11.875937, "Y  position"=-8.449351, "Z  position"=0.69921476, "Echo width"=1.36, "Device ID "=120, "Layer"=3, "Echo"=0, "Reserved"=0, "Timestamp"=0, "flags"=16, "Reserved 2"=30}, {"X  position"=11.782929, "Y  position"=-8.428771, "Z  position"=0.20246059, "Echo width"=1.56, "Device ID "=120, "Layer"=0, "Echo"=0, "Reserved"=0, "Timestamp"=0, "flags"=0, "Reserved 2"=30}, {"X  position"=11.924724, "Y  position"=-8.573061, "Z  position"=0.36608523, "Echo width"=1.7199999, "Device ID "=120, "Layer"=1, "Echo"=0, "Reserved"=0, "Timestamp"=0, "flags"=0, "Reserved 2"=30}, {"X  position"=11.7337265, "Y  position"=-8.452157, "Z  position"=0.53237885, "Echo width"=1.8399999, "Device ID "=120, "Layer"=2, "Echo"=0, "Reserved"=0, "Timestamp"=0, "flags"=0, "Reserved 2"=30}, {"X  position"=11.69724, "Y  position"=-8.414702, "Z  position"=0.6960734, "Echo width"=1.64, "Device ID "=120, "Layer"=3, "Echo"=0, "Reserved"=0, "Timestamp"=0, "flags"=0, "Reserved 2"=30}, {"X  position"=11.639609, "Y  position"=-8.428813, "Z  position"=0.20455484, "Echo width"=0.96, "Device ID "=120, "Layer"=0, "Echo"=0, "Reserved"=0, "Timestamp"=0, "flags"=16, "Reserved 2"=30}, {"X  position"=11.634251, "Y  position"=-8.4232645, "Z  position"=0.36824942, "Echo width"=1.3199999, "Device ID "=120, "Layer"=1, "Echo"=0, "Reserved"=0, "Timestamp"=0, "flags"=16, "Reserved 2"=30}, {"X  position"=11.562845, "Y  position"=-8.422558, "Z  position"=0.53140146, "Echo width"=1.56, "Device ID "=120, "Layer"=2, "Echo"=0, "Reserved"=0, "Timestamp"=0, "flags"=16, "Reserved 2"=30}, {"X  position"=11.519792, "Y  position"=-8.3775835, "Z  position"=0.692932, "Echo width"=1.0799999, "Device ID "=120, "Layer"=3, "Echo"=0, "Reserved"=0, "Timestamp"=0, "flags"=16, "Reserved 2"=30}, {"X  position"=11.44187, "Y  position"=-8.368984, "Z  position"=0.20832446, "Echo width"=1.56, "Device ID "=120, "Layer"=0, "Echo"=0, "Reserved"=0, "Timestamp"=0, "flags"=0, "Reserved 2"=30}, {"X  position"=11.484717, "Y  position"=-8.414137, "Z  position"=0.36901736, "Echo width"=1.4, "Device ID "=120, "Layer"=1, "Echo"=0, "Reserved"=0, "Timestamp"=0, "flags"=0, "Reserved 2"=30}, {"X  position"=11.386263, "Y  position"=-8.383345, "Z  position"=0.53035426, "Echo width"=1.4, "Device ID "=120, "Layer"=2, "Echo"=0, "Reserved"=0, "Timestamp"=0, "flags"=0, "Reserved 2"=30}, {"X  position"=11.480631, "Y  position"=-8.483661, "Z  position"=0.69397914, "Echo width"=1.28, "Device ID "=120, "Layer"=3, "Echo"=0, "Reserved"=0, "Timestamp"=0, "flags"=0, "Reserved 2"=30}, {"X  position"=11.34808, "Y  position"=-8.416035, "Z  position"=0.20895275, "Echo width"=1.52, "Device ID "=120, "Layer"=0, "Echo"=0, "Reserved"=0, "Timestamp"=0, "flags"=16, "Reserved 2"=30}, {"X  position"=11.376889, "Y  position"=-8.44693, "Z  position"=0.36936644, "Echo width"=1.36, "Device ID "=120, "Layer"=1, "Echo"=0, "Reserved"=0, "Timestamp"=0, "flags"=16, "Reserved 2"=30}, {"X  position"=11.367109, "Y  position"=-8.5105915, "Z  position"=0.5309128, "Echo width"=1.0799999, "Device ID "=120, "Layer"=2, "Echo"=0, "Reserved"=0, "Timestamp"=0, "flags"=16, "Reserved 2"=30}, {"X  position"=14.514519, "Y  position"=-11.9154415, "Z  position"=0.7898954, "Echo width"=2.32, "Device ID "=120, "Layer"=3, "Echo"=0, "Reserved"=0, "Timestamp"=0, "flags"=0, "Reserved 2"=31}, {"X  position"=11.2270565, "Y  position"=-8.432603, "Z  position"=0.21041872, "Echo width"=1.8, "Device ID "=120, "Layer"=0, "Echo"=0, "Reserved"=0, "Timestamp"=0, "flags"=0, "Reserved 2"=30}, {"X  position"=11.269098, "Y  position"=-8.478482, "Z  position"=0.3697155, "Echo width"=1.8, "Device ID "=120, "Layer"=1, "Echo"=0, "Reserved"=0, "Timestamp"=0, "flags"=0, "Reserved 2"=30}, {"X  position"=11.285818, "Y  position"=-8.571517, "Z  position"=0.53084296, "Echo width"=1.5999999, "Device ID "=120, "Layer"=2, "Echo"=0, "Reserved"=0, "Timestamp"=0, "flags"=0, "Reserved 2"=30}, {"X  position"=11.5262985, "Y  position"=-8.8362665, "Z  position"=0.7000525, "Echo width"=0.91999996, "Device ID "=120, "Layer"=3, "Echo"=0, "Reserved"=0, "Timestamp"=0, "flags"=4100, "Reserved 2"=0}, {"X  position"=14.571452, "Y  position"=-12.188719, "Z  position"=0.79492164, "Echo width"=1.16, "Device ID "=120, "Layer"=3, "Echo"=1, "Reserved"=0, "Timestamp"=0, "flags"=0, "Reserved 2"=31}, {"X  position"=11.119724, "Y  position"=-8.462563, "Z  position"=0.21146584, "Echo width"=1.64, "Device ID "=120, "Layer"=0, "Echo"=0, "Reserved"=0, "Timestamp"=0, "flags"=16, "Reserved 2"=30}, {"X  position"=11.194814, "Y  position"=-8.545958, "Z  position"=0.3697155, "Echo width"=1.76, "Device ID "=120, "Layer"=1, "Echo"=0, "Reserved"=0, "Timestamp"=0, "flags"=16, "Reserved 2"=30}, {"X  position"=11.164111, "Y  position"=-8.586911, "Z  position"=0.53035426, "Echo width"=1.04, "Device ID "=120, "Layer"=2, "Echo"=0, "Reserved"=0, "Timestamp"=0, "flags"=16, "Reserved 2"=30}, {"X  position"=14.424722, "Y  position"=-12.240116, "Z  position"=0.79366505, "Echo width"=1.4, "Device ID "=120, "Layer"=3, "Echo"=0, "Reserved"=0, "Timestamp"=0, "flags"=0, "Reserved 2"=31}, {"X  position"=11.078711, "Y  position"=-8.566174, "Z  position"=0.21041872, "Echo width"=1.8, "Device ID "=120, "Layer"=0, "Echo"=0, "Reserved"=0, "Timestamp"=0, "flags"=0, "Reserved 2"=30}, {"X  position"=11.06031, "Y  position"=-8.545376, "Z  position"=0.3703438, "Echo width"=1.88, "Device ID "=120, "Layer"=1, "Echo"=0, "Reserved"=0, "Timestamp"=0, "flags"=0, "Reserved 2"=30}, {"X  position"=11.128445, "Y  position"=-8.698574, "Z  position"=0.53077316, "Echo width"=1.52, "Device ID "=120, "Layer"=2, "Echo"=0, "Reserved"=0, "Timestamp"=0, "flags"=0, "Reserved 2"=30}, {"X  position"=14.83826, "Y  position"=-12.928807, "Z  position"=0.8102096, "Echo width"=1.76, "Device ID "=120, "Layer"=3, "Echo"=0, "Reserved"=0, "Timestamp"=0, "flags"=0, "Reserved 2"=32}, {"X  position"=11.010227, "Y  position"=-8.639529, "Z  position"=0.21020928, "Echo width"=1.3199999, "Device ID "=120, "Layer"=0, "Echo"=0, "Reserved"=0, "Timestamp"=0, "flags"=16, "Reserved 2"=30}, {"X  position"=11.031374, "Y  position"=-8.663855, "Z  position"=0.36985514, "Echo width"=1.48, "Device ID "=120, "Layer"=1, "Echo"=0, "Reserved"=0, "Timestamp"=0, "flags"=16, "Reserved 2"=30}, {"X  position"=14.607534, "Y  position"=-12.890929, "Z  position"=0.80644, "Echo width"=1.4399999, "Device ID "=120, "Layer"=3, "Echo"=0, "Reserved"=0, "Timestamp"=0, "flags"=0, "Reserved 2"=32}, {"X  position"=10.986493, "Y  position"=-8.765557, "Z  position"=0.2085339, "Echo width"=1.48, "Device ID "=120, "Layer"=0, "Echo"=0, "Reserved"=0, "Timestamp"=0, "flags"=0, "Reserved 2"=30}, {"X  position"=10.987953, "Y  position"=-8.767266, "Z  position"=0.36950606, "Echo width"=1.56, "Device ID "=120, "Layer"=1, "Echo"=0, "Reserved"=0, "Timestamp"=0, "flags"=0, "Reserved 2"=30}, {"X  position"=11.078849, "Y  position"=-8.952498, "Z  position"=0.53189015, "Echo width"=0.91999996, "Device ID "=120, "Layer"=2, "Echo"=0, "Reserved"=0, "Timestamp"=0, "flags"=4, "Reserved 2"=0}, {"X  position"=11.968827, "Y  position"=-10.003783, "Z  position"=0.72455513, "Echo width"=1.52, "Device ID "=120, "Layer"=3, "Echo"=0, "Reserved"=0, "Timestamp"=0, "flags"=4, "Reserved 2"=0}]}, "Header"=w320, "Scan header"=w319, "Scanner info"=w317, "Scan points"=w316) -> ()  [unwired: 1 out]
                            }
                          }
                        }
                        frame 8737 {
                          n131 = disable-structure shown="Enabled" {
                            disable-tunnel: w331 -> [w345 _]
                            disable-tunnel: w330 -> [w340 _]
                            disable-tunnel: w329 -> [w335 _]
                            disable-tunnel: [w333 _] -> w328
                            frame Enabled {
                              w341 = cluster{"NTP time":u64, "Number of objects":u16} {"NTP time"=20, "Number of objects"=0}  # Object header
                              n132 = String Subset(string=w345, length (rest)=10 ("length (rest)")) -> (substring=w348:string)  [unwired: 1 in]
                              n133 = Unflatten From String(type=w341, binary string=w348, data includes array or string size? (T)=FALSE, byte order (0:big-endian, network order)=T5."little-endian", error in (no error)=w335) -> (value=w336:cluster{"NTP time":u64, "Number of objects":u16}, error out=w334:errorcluster)  [unwired: 1 out]
                              n134 = String Subset(string=w345, offset (0)=10 ("length (rest)")) -> (substring=w344:string)  [unwired: 1 in]
                              n135 = Unbundle By Name(w336) -> ("Number of objects"=w343:u16)
                              n136 = for {
                                N: w343 -> [_]
                                shift-right: [w368] -> w338
                                shift-left: w344 -> [w370]
                                tunnel: [w366] -> w342 mode=indexing
                                shift-right: [w360] -> w333
                                shift-left: w334 -> [w362]
                                w365 = T17 {"Object ID"=0, "Object age "=0, "Object prediction age"=0, "Relative timestamp"=0, "Reference point X"=0, "Reference point Y"=0, "Reference point sigma X"=0, "Reference point sigma Y"=0, "Closest point X"=0, "Closest point Y"=0, "Bounding box center X"=0, "Bounding box center Y"=0, "Bounding box size X"=0, "Bounding box size Y"=0, "Object box center X"=0, "Object box center Y"=0, "Object box size X"=0, "Object box size Y"=0, "Object box orientation"=0, "Absolute velocity X"=0, "Absolute velocity Y"=0, "Absolute velocity sigma X"=0, "Absolute velocity sigma Y"=0, "Relative velocity X"=0, "Relative velocity Y"=0, "Classification"=0, "Classification age"=0, "Classification certainty"=0, "Number of contour points"=0}  # object
                                n137 = Unflatten From String(type=w365, binary string=w370, data includes array or string size? (T)=FALSE, byte order (0:big-endian, network order)=T5."little-endian", error in (no error)=w362) -> (rest of the binary string=w369:string, value=w364:T17, error out=w361:errorcluster)
                                n138 = disable-structure shown="Enabled" {
                                disable-tunnel: w364 -> [w373 _]
                                disable-tunnel: [w372 1] -> w358
                                frame Disabled {
                                n139 = Unbundle By Name(w373) -> ("Number of contour points"=w372:u16)
                                }
                                frame Enabled {
                                }
                                }
                                n140 = for {
                                N: w358 -> [_]
                                shift-right: [w424] -> w368
                                shift-left: w369 -> [w425]
                                tunnel: [w419] -> w367 mode=indexing
                                shift-right: [w417] -> w360
                                shift-left: w361 -> [w418]
                                w423 = T18 {"contour points X"=0, "contour points Y"=0}  # contour point
                                n141 = Unflatten From String(type=w423, binary string=w425, data includes array or string size? (T)=FALSE, byte order (0:big-endian, network order)=T5."little-endian", error in (no error)=w418) -> (rest of the binary string=w424:string, value=w422:T18, error out=w417:errorcluster)
                                n142 = To Double Precision Float(number=w422) -> (double precision float=w421:T19)
                                n143 = Multiply(x=w421, y=0.01) -> (x*y=w419:T19)
                                }
                                n144 = flat-sequence {
                                tunnel: w364 -> [w411]
                                tunnel: [w409] -> w363
                                frame #0 {
                                w412 = T20 {"Object ID"=0, "Object age "=0, "Object prediction age"=0, "Relative timestamp"=0, "Reference point X"=0.0, "Reference point Y"=0.0, "Reference point sigma X"=0.0, "Reference point sigma Y"=0.0, "Closest point X"=0.0, "Closest point Y"=0.0, "Bounding box center X"=0.0, "Bounding box center Y"=0.0, "Bounding box size X"=0.0, "Bounding box size Y"=0.0, "Object box center X"=0.0, "Object box center Y"=0.0, "Object box size X"=0.0, "Object box size Y"=0.0, "Object box orientation"=0.0, "Absolute velocity X"=0.0, "Absolute velocity Y"=0.0, "Absolute velocity sigma X"=0.0, "Absolute velocity sigma Y"=0.0, "Relative velocity X"=0.0, "Relative velocity Y"=0.0, "Classification"=0, "Classification age"=0, "Classification certainty"=0, "Number of contour points"=0}  # object
                                n145 = To Double Precision Float(number=w411) -> (double precision float=w415:T21)
                                n146 = Divide(x=3.141592653589793, y=32.0) -> (x/y=w375:dbl)
                                n147 = Unbundle By Name(w411) -> ("Object box orientation"=w379:i16, "Object ID"=w410:u16, "Object age"=w408:u16, "Object prediction age"=w407:u16, "Relative timestamp"=w406:u16, "Classification"=w405:u16, "Classification age"=w404:u16, "Classification certainty"=w403:u16, "Number of contour points"=w402:u16)
                                n148 = Divide(x=w375, y=180.0) -> (x/y=w378:dbl)
                                n149 = Multiply(x=w415, y=0.01) -> (x*y=w413:T21)
                                n150 = Unbundle By Name(w413) -> ("Reference point X"=w401:dbl, "Reference point Y"=w400:dbl, "Reference point sigma X"=w399:dbl, "Reference point sigma Y"=w398:dbl, "Closest point X"=w397:dbl, "Closest point Y"=w396:dbl, "Bounding box center X"=w395:dbl, "Bounding box center Y"=w394:dbl, "Bounding box size X"=w393:dbl, "Bounding box size Y"=w392:dbl, "Object box center X"=w391:dbl, "Object box center Y"=w390:dbl, "Object box size X"=w389:dbl, "Object box size Y"=w388:dbl, "Absolute velocity X"=w387:dbl, "Absolute velocity Y"=w386:dbl, "Absolute velocity sigma X"=w385:dbl, "Absolute velocity sigma Y"=w384:dbl, "Relative velocity X"=w383:dbl, "Relative velocity Y"=w382:dbl)
                                n151 = Multiply(x=w378, y=w379) -> (x*y=w377:dbl)
                                n152 = Bundle By Name(cluster=w412, "Object box orientation"=w377, "Object ID"=w410, "Object age"=w408, "Object prediction age"=w407, "Relative timestamp"=w406, "Classification"=w405, "Classification age"=w404, "Classification certainty"=w403, "Number of contour points"=w402, "Reference point X"=w401, "Reference point Y"=w400, "Reference point sigma X"=w399, "Reference point sigma Y"=w398, "Closest point X"=w397, "Closest point Y"=w396, "Bounding box center X"=w395, "Bounding box center Y"=w394, "Bounding box size X"=w393, "Bounding box size Y"=w392, "Object box center X"=w391, "Object box center Y"=w390, "Object box size X"=w389, "Object box size Y"=w388, "Absolute velocity X"=w387, "Absolute velocity Y"=w386, "Absolute velocity sigma X"=w385, "Absolute velocity sigma Y"=w384, "Relative velocity X"=w383, "Relative velocity Y"=w382) -> (w409:T20)
                                }
                                }
                                n153 = Bundle("object"=w363, w367) -> (w366:T22)  [unwired: 1 in]
                              }
                              n154 = Equal?(x=w338, y="") -> (x = y?=w337:bool)
                              n155 = case shown="True" w337 {
                                tunnel: w342 -> [_ w357]
                                tunnel: w336 -> [_ w356]
                                tunnel: w340 -> [_ w355]
                                frame False {
                                }
                                frame True {
                                n156 = Bundle(cluster=T2 {"Header"={"Size of prev messages"=0, "Size of this messages"=0, "Reserved"=0, "DeviceID"=0, "Data type"=0, "NTP time"=0}, "Object header"={"NTP time"=0, "Number of objects"=0}, "Objects"=[]} ("object data 2221"), "Header"=w355, "Object header"=w356, "Objects"=w357) -> (w351:T2)
                                "output cluster 2" <- w351
                                n157 = Flatten To String(anything=w351, prepend array or string size? (T)=FALSE, byte order (0:big-endian, network order)=T5."native, host order") -> (data string=w350:string)  [unwired: 1 in, 2 out]
                                "object data 2221" <- w350
                                n158 = global write "G_SEN.vi" "B_object data 2221"(w350) -> ()
                                }
                              }
                            }
                            frame Disabled {
                            }
                          }
                        }
                        frame 8741 {
                          w440 = cluster{"NTP time":u64, "Number of objects":u16} {"NTP time"=20, "Number of objects"=0}  # Object header
                          n159 = String Subset(string=w438, length (rest)=10 ("length (rest)")) -> (substring=w442:string)  [unwired: 1 in]
                          n160 = Unflatten From String(type=w440, binary string=w442, data includes array or string size? (T)=FALSE, error in (no error)=w429) -> (value=w434:cluster{"NTP time":u64, "Number of objects":u16}, error out=w428:errorcluster)  [unwired: 1 in, 1 out]
                          n161 = String Subset(string=w438, offset (0)=10 ("length (rest)")) -> (substring=w437:string)  [unwired: 1 in]
                          n162 = Unbundle By Name(w434) -> ("Number of objects"=w436:u16)
                          n163 = for {
                            N: w436 -> [_]
                            shift-right: [w454] -> w431
                            shift-left: w437 -> [w457]
                            tunnel: [w451] -> w433 mode=indexing
                            shift-right: [w448] -> w427
                            shift-left: w428 -> [w450]
                            w458 = T23 {"Object ID"=0, "Reserved 2 1"=0, "Object age "=0, "Timestamp NTP "=0, "Object hidden status age"=0, "Classification"=0, "Classification certainty"=0, "Classification age"=0, "Bounding box center X"=0.0, "Bounding box center Y"=0.0, "Bounding box size X"=0.0, "Bounding box size Y"=0.0, "Object box center X"=0.0, "Object box center Y"=0.0, "Object box center sigma X"=0.0, "Object box center sigma Y"=0.0, "Object box size X"=0.0, "Object box size Y"=0.0, "Reserved 8 1"=0, "Yaw angle"=0.0, "Reserved 4"=0, "Relative velocity X"=0.0, "Relative velocity Y"=0.0, "Relative velocity sigma X"=0.0, "Relative velocity sigma Y"=0.0, "Absolute velocity X"=0.0, "Absolute velocity Y"=0.0, "Absolute velocity sigma X"=0.0, "Absolute velocity sigma Y"=0.0, "Reserved 8 3"=0, "Reserved 8 4"=0, "Reserved 2 2"=0, "Number of contour points"=0, "Index of closest point"=0}  # object
                            n164 = Unflatten From String(type=w458, binary string=w457, data includes array or string size? (T)=FALSE, error in (no error)=w450) -> (rest of the binary string=w455:string, value=w453:T23, error out=w449:errorcluster)  [unwired: 1 in]
                            n165 = Unbundle By Name(w453) -> ("Number of contour points"=w456:u8)
                            n166 = for {
                              N: w456 -> [_]
                              shift-right: [w464] -> w454
                              shift-left: w455 -> [w465]
                              tunnel: [w463] -> w452 mode=indexing
                              shift-right: [w460] -> w448
                              shift-left: w449 -> [w461]
                              w462 = T24 {"contour points X"=0.0, "contour points Y"=0.0}  # contour point
                              n167 = Unflatten From String(type=w462, binary string=w465, data includes array or string size? (T)=FALSE, error in (no error)=w461) -> (rest of the binary string=w464:string, value=w463:T24, error out=w460:errorcluster)  [unwired: 1 in]
                            }
                            n168 = Bundle("object"=w453, w452) -> (w451:T25)  [unwired: 1 in]
                          }
                          n169 = Equal?(x=w431, y="") -> (x = y?=w430:bool)
                          n170 = case shown="True" w430 {
                            tunnel: w435 -> [_ w446]
                            tunnel: w434 -> [_ w445]
                            tunnel: w433 -> [_ w444]
                            frame False {
                            }
                            frame True {
                              n171 = Bundle By Name(cluster=T9 {"Header"={"Size of prev messages"=0, "Size of this messages"=0, "Reserved"=0, "DeviceID"=0, "Data type"=0, "NTP time"=0}, "Object header"={"NTP time"=0, "Number of objects"=0}, "Objects"=[]} ("output cluster"), "Header"=w446, "Object header"=w445, "Objects"=w444) -> ()  [unwired: 1 out]
                            }
                          }
                        }
                      }
                      n172 = feedback #2(w146) -> (w145:dbl)
                      n173 = feedback-in #2(w146) -> ()
                      n174 = Subtract(x=w146, y=w145) -> (x-y=→"time IBEO":dbl)
                    }
                  }
                }
              }
            }
          }
          "Ibeo error out" <- w82
        }
        n175 = Not Equal?(x=refnum<k5> refnum, y=w76) -> (x != y?=w79:bool)
        n176 = case shown="True" w79 {
          tunnel: w76 -> [_ w80]
          frame False {
          }
          frame True {
            n177 = TCP Close Connection(connection ID=w80) -> ()  [unwired: 2 in, 2 out]
          }
        }
      }
    }
    n178 = Not(x="Ibeo reconn?") -> (.not. x?=w73:bool)
  }
